vi "CRYAnalysis Editor.vi"() -> ()   [LabVIEW 2013]
uses:
  <vilib>/Utility/miscctls.llb/LVBoundsTypeDef.ctl
  Typedef Control/CRYAnalysis Cluster.ctl
  CRYProject/CRYProject Editor Global.vi
  CRYMainGlobal.vi
  Hardware/CRYHardware Global.vi
  CRYStepSetup/CRYStepSetup Global.vi
panel:
  out "Changed Curve 2":string[][](array[string])
  out "Analysis Bk":T1={"Name"="", "Harmonics"=[1.0], " Algorithm"=0, "delay"=0.0, "THD(%)"=FALSE, "Rub&Buzz"=FALSE, "Imp"=FALSE, "Imp Ref resistor"=1.0, "Y data"=0, "Y prefix"="", "Y unit"="", "Y dB ref"=1.0, "Custom Curve Names"=[], "har list items"=[""], "Envelope"=FALSE, "use custom unit"=FALSE, "autodelay ch"=0.0, "impulse"=FALSE, " start ms"=1.0, " stop ms"=1.0, "Scaling"=1, "Default Overlap "=FALSE, "Advanced View"=FALSE, "Loose Particle"=FALSE, "Use default"=FALSE, "Auto-Correlation(Stimulus)"=FALSE, "Auto-Correlation(Response)"=FALSE, "Deconvolved Response"=FALSE, "Mic Current"=FALSE, "M List Vaiues"=0, "Type"=0, "Delay Method"=3, "Apply Correction Out"=FALSE, "Apply Correction In"=FALSE, "Harmonics @ meas.frq"=FALSE, "THD Normalized(%)"=FALSE, "Total Distortion"=FALSE, "THD+Noise(%)"=FALSE, "Rub&Buzz Norm'd(%)"=FALSE, "Standard Error"=FALSE, "Confidence Limits"=FALSE, "Total Diff"=FALSE, "Total Noise"=FALSE, "Total DFD(%)"=FALSE, "Total IMD(%)"=FALSE, "Total IM"=FALSE, "Total DFD+Noise(%)"=FALSE, "Use Channel Name"=FALSE, "Waveform In"="", "Waveform Out"="", "Method"=3, "Spectral Scaling"=3, "Appliied Unit"=1, "Length Unit"=1, "Applied Units"=1, "Sens Item"=0, "Tab"=1, "Distance Unit"=0, "discard cycles"=1.0, "Weigting"="", "Averaging Time"=0.0, "Max duration"=0.0, "Min duration"=0.0, "Attack Threshold"=0.0, "Hysteresis Up"=0.0, "Fmin(Hz)"=0.0, "Fmax(Hz)"=0.0, "Freq.Resolution"=0.0, "Over-samples Res."=0.0, "Win Resolution"=0.0, "distance"=0.0, "samples"=1.0, "Overlap"=1.0, "Record Length"=1.0, "No.of FFTs"=0.0, "Hz"=1.0, "record delay"=1.0, " Std Err"=1.0, "Response"=FALSE, "Coherent Power*"=FALSE, "Stimulus"=FALSE, "Measurement Confidence"=FALSE, "Auto Spectrum(Response)*"=FALSE, "Auto Spectrum(Stimulus)*"=FALSE, "Cross Spectrum*"=FALSE, "functions"=FALSE, "Frequency Response"=FALSE, "Non-Coherent Power*"=FALSE, "Coherence (%)"=FALSE, "Non-Coherence (%)"=FALSE, "Signal-Noise Ratio (dB)"=FALSE, "Non-Coherenct Distirtion*"=FALSE, "Result Waveforms"=FALSE, "Coupling"=FALSE, "Averaging"=0, "Harmonics"=0, "Custom Curve Names"=0, "unLabel"="", "Custom Curve Names"="", "Unit"="", "Total IMD + Noise(%) "=FALSE, "ResponseMe"=1, "Intermod"=[1.0], "Diff\n"=[1.0], "Cross-Correlation"=FALSE, "IM list items"=[""], "Diff list items"=[""], "TSR Window Type"="", "Help"="", "Custom Curve IDs"=[], "Default Curve Names"=[], "Loose Particle waveform"=FALSE, "Perceptual Rub&Buzz"=FALSE, "Imp Auto Mode"=0, "Mic Auto Mode"=0, "Mic Ref resistor"=1.0, "Curve Resolution"=3, "Curve Resolution Hz"=0.0, "Polarity"=FALSE} {"Curve Resolution Hz" format="%.2f"; "Mic Ref resistor" format="%.2f"; "Diff" format="%.2f"; "Intermod" format="%.2f"; "ResponseMe" items=["Absolute", "Relative"]; "Std Err" format="%.1f"; "record delay" format="%.1f"; "Hz" format="%.1f"; "No.of FFTs" format="%.2f"; "Record Length" format="%.1f"; "Overlap" format="%.1f"; "samples" format="%.1f"; "distance" format="%.2f"; "Win Resolution" format="%.2f"; "Over-samples Res." format="%.2f"; "Freq.Resolution" format="%.2f"; "Fmax(Hz)" format="%.2f"; "Fmin(Hz)" format="%.2f"; "Hysteresis Up" format="%.2f"; "Attack Threshold" format="%.2f"; "Min duration" format="%.2f"; "Max duration" format="%.2f"; "Averaging Time" format="%.2f"; "Distance Unit" items=["Absolute", "Relative"]; "Sens Item" items=["x", "y", "z"]; "Applied Units" items=["Absolute", "Relative"]; "Length Unit" items=["Absolute", "Relative"]; "Appliied Unit" items=["Absolute", "Relative"]; "Spectral Scaling" items=["Absolute", "Relative"]; "M List Vaiues" items=["x", "y", "z"]; "Scaling" format="%.1f"; "stop ms" format="%.1f"; "start ms" format="%.1f"; "Y data" items=["dB", "Lin"]; "Y dB ref" format="%.1f"; "Imp Ref resistor" format="%.2f"; "Harmonics" format="%.2f"; "delay" format="%.2f"}
  in  "CurLibChange":bool caption="Add Lib"
  in  "Change Use Channel?":bool
  in  "Manual Apply":bool caption="Apply"
  in  "Mode":string
  out "Old Name":string[](array[string])
  out "Changed Curve":string[][](array[string])
  in  "Change Curve Name?":bool
  out "EndFlag":bool
  in  "Add Lib":bool
  in  "AddStep":bool
  in  "CurveUpdate":bool
  out "Wave In Fs":dbl
  out "Wave Ou Sn":dbl
  out "Wave Out Fs":dbl
  in  "Delay Treat":u16(slide)
  out "Common dB #":u16
  out "Wave In Sn":i32
  in  "distance":dbl
  in  "Visible Update":bool
  in  "Diff checkoffs":bool[](array[boolean])
  out "Diff array out":dbl[](array[numeric]) format="%.2f"
  in  "IM checkoffs":bool[](array[boolean])
  out "IM array out":dbl[](array[numeric]) format="%.2f"
  out "Harmonics array out":dbl[](array[numeric]) format="%.2f"
  out "CurveArrayByType":string[](array[string])
  in  "Hardware In Fs":dbl
  out "Analysis":T1={"Name"="", "Harmonics"=[1.0], " Algorithm"=0, "delay"=0.0, "THD(%)"=FALSE, "Rub&Buzz"=FALSE, "Imp"=FALSE, "Imp Ref resistor"=1.0, "Y data"=0, "Y prefix"="", "Y unit"="", "Y dB ref"=1.0, "Custom Curve Names"=[], "har list items"=[""], "Envelope"=FALSE, "use custom unit"=FALSE, "autodelay ch"=0.0, "impulse"=FALSE, " start ms"=1.0, " stop ms"=1.0, "Scaling"=1, "Default Overlap "=FALSE, "Advanced View"=FALSE, "Loose Particle"=FALSE, "Use default"=FALSE, "Auto-Correlation(Stimulus)"=FALSE, "Auto-Correlation(Response)"=FALSE, "Deconvolved Response"=FALSE, "Mic Current"=FALSE, "M List Vaiues"=0, "Type"=0, "Delay Method"=3, "Apply Correction Out"=FALSE, "Apply Correction In"=FALSE, "Harmonics @ meas.frq"=FALSE, "THD Normalized(%)"=FALSE, "Total Distortion"=FALSE, "THD+Noise(%)"=FALSE, "Rub&Buzz Norm'd(%)"=FALSE, "Standard Error"=FALSE, "Confidence Limits"=FALSE, "Total Diff"=FALSE, "Total Noise"=FALSE, "Total DFD(%)"=FALSE, "Total IMD(%)"=FALSE, "Total IM"=FALSE, "Total DFD+Noise(%)"=FALSE, "Use Channel Name"=FALSE, "Waveform In"="", "Waveform Out"="", "Method"=3, "Spectral Scaling"=3, "Appliied Unit"=1, "Length Unit"=1, "Applied Units"=1, "Sens Item"=0, "Tab"=1, "Distance Unit"=0, "discard cycles"=1.0, "Weigting"="", "Averaging Time"=0.0, "Max duration"=0.0, "Min duration"=0.0, "Attack Threshold"=0.0, "Hysteresis Up"=0.0, "Fmin(Hz)"=0.0, "Fmax(Hz)"=0.0, "Freq.Resolution"=0.0, "Over-samples Res."=0.0, "Win Resolution"=0.0, "distance"=0.0, "samples"=1.0, "Overlap"=1.0, "Record Length"=1.0, "No.of FFTs"=0.0, "Hz"=1.0, "record delay"=1.0, " Std Err"=1.0, "Response"=FALSE, "Coherent Power*"=FALSE, "Stimulus"=FALSE, "Measurement Confidence"=FALSE, "Auto Spectrum(Response)*"=FALSE, "Auto Spectrum(Stimulus)*"=FALSE, "Cross Spectrum*"=FALSE, "functions"=FALSE, "Frequency Response"=FALSE, "Non-Coherent Power*"=FALSE, "Coherence (%)"=FALSE, "Non-Coherence (%)"=FALSE, "Signal-Noise Ratio (dB)"=FALSE, "Non-Coherenct Distirtion*"=FALSE, "Result Waveforms"=FALSE, "Coupling"=FALSE, "Averaging"=0, "Harmonics"=0, "Custom Curve Names"=0, "unLabel"="", "Custom Curve Names"="", "Unit"="", "Total IMD + Noise(%) "=FALSE, "ResponseMe"=1, "Intermod"=[1.0], "Diff\n"=[1.0], "Cross-Correlation"=FALSE, "IM list items"=[""], "Diff list items"=[""], "TSR Window Type"="", "Help"="", "Custom Curve IDs"=[], "Default Curve Names"=[], "Loose Particle waveform"=FALSE, "Perceptual Rub&Buzz"=FALSE, "Imp Auto Mode"=0, "Mic Auto Mode"=0, "Mic Ref resistor"=1.0, "Curve Resolution"=3, "Curve Resolution Hz"=0.0, "Polarity"=FALSE} {"Curve Resolution Hz" format="%.2f"; "Mic Ref resistor" format="%.2f"; "Diff" format="%.2f"; "Intermod" format="%.2f"; "ResponseMe" items=["Absolute", "Relative"]; "Std Err" format="%.1f"; "record delay" format="%.1f"; "Hz" format="%.1f"; "No.of FFTs" format="%.2f"; "Record Length" format="%.1f"; "Overlap" format="%.1f"; "samples" format="%.1f"; "distance" format="%.2f"; "Win Resolution" format="%.2f"; "Over-samples Res." format="%.2f"; "Freq.Resolution" format="%.2f"; "Fmax(Hz)" format="%.2f"; "Fmin(Hz)" format="%.2f"; "Hysteresis Up" format="%.2f"; "Attack Threshold" format="%.2f"; "Min duration" format="%.2f"; "Max duration" format="%.2f"; "Averaging Time" format="%.2f"; "Distance Unit" items=["Absolute", "Relative"]; "Sens Item" items=["x", "y", "z"]; "Applied Units" items=["Absolute", "Relative"]; "Length Unit" items=["Absolute", "Relative"]; "Appliied Unit" items=["Absolute", "Relative"]; "Spectral Scaling" items=["Absolute", "Relative"]; "M List Vaiues" items=["x", "y", "z"]; "Scaling" format="%.1f"; "stop ms" format="%.1f"; "start ms" format="%.1f"; "Y data" items=["dB", "Lin"]; "Y dB ref" format="%.1f"; "Imp Ref resistor" format="%.2f"; "Harmonics" format="%.2f"; "delay" format="%.2f"}
  in  "Load Test":bool
  out "Proper VI No":i32
  in  "Autodelay Channel":dbl
  out "VIMiniumBound":T2
  in  "Board Tab":enum32{"Page 1", "Page 2"}(tab)
  in  "Cancel":bool caption="Apply"
  in  "OK":bool caption="Apply"
  in  "Main Tab":T3(tab)
  in  "Use default":bool=TRUE caption="使用默认"
  in  "Use Channel Name":bool caption="使用频道名称"
  in  "Custom Curve Names":string[][](table) caption="自定义的曲线名称"
  in  "units":bool
  in  "Unit":string="Pa" caption="单位"
  in  "Applied Units":u16(ring) caption="应用单位" items=["seconds", "samples", "inches", "meters"]
  in  "Hz":dbl format="%#.3p"
  in  "LR":u16(ring) items=["unity cal-in sens-in", "CRY33x Mic 1 sens-in", "CRY33x Mic 2 sens-in", "CRY33x Mic 3 sens-in", "CRY33x Mic 4 sens-in", "USB In L sens-in", "USB In R sens-in", "unity cal-out sens-out", "CRY602 Mouth 1 sens-out", "CRY602 Mouth 2 sens-out", "USB Out R sens-out"]
  in  "Distance Unit":u16(ring) items=["英寸", "米"]
  in  "samples":dbl=44100000.0 caption="样本" min=1.0 format="%#.0f"
  in  "s":dbl caption="秒" format="%#.4f"
  in  "distance":dbl caption="距离" min=0.0 format="%#.2f"
  in  "Delay Method":u16(slide) caption="延迟方法"
  in  "Maxis":u16(slide) scale=0.0..2.0
  out "CurveLibValues":bool caption="曲线值"
  out "Record Delay":bool caption="记录延迟"
  in  "Polarity":bool caption="极性"
  out "Curve Resolution":bool caption="曲线分辨"
  out "Spectra":bool caption="频谱"
  in  "Auto-Spectrum(Response)*":bool caption="自动频谱(响应)"
  in  "Auto-Spectrum(Stimulus)*":bool caption="自动频谱(激励)"
  in  "Spectral Scaling*":u16(ring) caption="频谱缩放*" items=["有效值", "频谱密度"]
  in  "Non-Coherent Power*":bool caption="非相干功率*"
  in  "Coherent Power*":bool caption="相干功率*"
  in  "Cross-Spectrum*":bool caption="交叉频谱*"
  out "Functions":bool caption="功能"
  in  "Frequency Response":bool caption="频率响应"
  in  "Coherence (%)":bool=TRUE caption="相干(%)"
  in  "Non-Coherence (%)":bool=TRUE caption="非相干(%)"
  in  "Signal-Noise Ratio (dB)":bool=TRUE caption="信噪比(dB)"
  in  "Non-Coherent Distortion*":bool=TRUE caption="非相干失真"
  in  "Averaging1":u16(slide)
  out "Averaging":bool caption="平均"
  in  "Curve Step Resolution":u16(ring) caption="Resolution" items=["R10(1/3 Oct.)"=0, "R20(1/6 Oct.)"=1, "R40(1/12 Oct.)"=2, "R80(1/24 Oct.)"=3, "User Defined, Log"=5, "User Defined,Linear"=6]
  in  "Curve Resolution Hz":dbl=10.0 caption="Hz" min=0.0 max=100000000.0 format="%#_10p"
  in  "Hysteresis Up(dB)":dbl=20.0 caption="磁滞现象上升(dB)" format="%#_6p"
  in  "Min duration(s)":dbl=20.0 caption="最小持续时间(s)" min=0.001 format="%#_6p"
  in  "Attack Threshold(dB)":dbl=20.0 caption="激发界限(dB)" min=0.0 format="%#_6p"
  in  "Max duration(s)":dbl=20.0 caption="最大持续时间(s)" min=0.0 format="%#_6p"
  in  "Loose Particle":bool caption="松散离子"
  in  "Averaging Time(s)":dbl=20.0 caption="平均时间(s)" min=0.0 format="%#_6p"
  in  "Loose Particle Waveform":bool=TRUE caption="松散离子波形"
  out "Channel in":string="L" caption="输入通道"
  out "Type in":string="Frequency Stepped Sweep" caption="输入类型"
  in  "Waveforms In":u16(ring) caption="输入波形"
  in  "Apply Correction in":bool caption="应用输入修正"
  out "Channel Out":string="L" caption="输出通道"
  out "Type Out":string="Frequency Stepped Sweep" caption="输出类型"
  in  "Waveforms Out":u16(ring) caption="输出波形"
  in  "Apply Correction Out":bool caption="应用输出修正"
  out "Stimulus":bool caption="激励"
  out "Response":bool caption="响应"
  out "Response Measurement":bool caption="响应测量"
  in  "Response Measurement1":u16(slide)
  in  "Perceptual Rub & Buzz(phons)":bool caption="感知异音(phons)"
  in  "Total DFD + Noise(%)":bool caption="共有DFD+噪声(%)"
  in  "Total DFD (%)":bool caption="共有DFD(%)"
  in  "Total Diff":bool caption="总差异"
  in  "THD + Noise (%)":bool caption="总谐波失真+噪声(%)"
  in  "THD Normalized(%)":bool caption="总谐波失真(归一化)(%)"
  in  "Rub & Buzz Norm'd(%)":bool caption="异音(归一化)(%)"
  in  "Rub & Buzz(%)":bool
  in  "Total Distortion":bool caption="总失真"
  in  "Harmonics @ meas.frq":bool caption="谐波测量频率"
  in  "Total IMD + Noise(%)":bool caption="共有IMD+噪声(%)"
  in  "Total IMD(%)":bool caption="共有IMD(%)"
  in  "Total IM":bool caption="共有IM"
  in  "Total Noise":bool caption="总噪声"
  in  "+/-":dbl=1.0 caption="标准错误" min=1.0 max=6.0 format="%#_6p"
  in  "Confidence Limits":bool caption="置信界限"
  in  "Standard Error":bool caption="标准差"
  in  "THD(%)":bool caption="总谐波失真(%)"
  out "Measurement Confidence":bool caption="测量置信度"
  in  "Edit List":bool
  in  "Method":u16(slide)
  in  "Type":u16(slide) caption="类型"
  in  "Harmonics":i32(listbox) caption="谐波"
  in  "Orders IM":i32(listbox) caption="次数"
  in  "Orders Diff":i32(listbox) caption="次数"
  in  "TSR Window Type":u16(ring) caption="TSR窗函数类型" items=["None", "Cosine Tapered", "Half-Cosine Tapered", "Exponential", "Adrienne", "Half-Hanning", "Half-BH4"]
  in  "Cross-Correlation":bool caption="互相关"
  out "No.of FFTs":i32=1 caption="FFT数量"
  out "Record Length (s)":dbl caption="FFT长度(s)" format="%#_3p"
  in  "Freq.Resolution(Hz)":dbl=10.0 caption="频率响应(Hz)" min=0.0 max=100000000.0 format="%#_10p"
  out "Windowed Resolution(Hz)":dbl=40.0 caption="窗函数分辨率(Hz)" format="%#.3p"
  in  "Over-samples Res.(Hz)":dbl=5.0 caption="曲线分辨率(Hz)" min=0.0 format="%#_6p"
  in  "StopTime(s)":dbl=10.0 caption="停止时间(秒)" min=0.0 format="%#_6p"
  in  "Start Time(s)":dbl=14.0 caption="开始时间(秒)" min=0.0 format="%#_6p"
  in  "Auto-Correlation(Response)":bool caption="自动相关(响应)"
  in  "Auto-Correlation(Stimulus)":bool caption="自动相关(激励)"
  in  "Deconvolved Response":bool caption="逆卷积响应"
  in  "Discard Cycles":dbl caption="丢弃周期" min=0.0 max=1000.0 format="%#_6p"
  in  "Fmin(Hz)":dbl=20.0 caption="最低频率(Hz)" min=0.0 format="%#_6p"
  in  "Fmax(Hz)":dbl=20000.0 caption="最大频率(Hz)" min=0.0 format="%#_6p"
  in  "Default Overlap":bool caption="默认重叠"
  in  "Overlap(%)":dbl=85.0 caption="重叠(%)" min=0.0 max=100.0 format="%#_6p"
  in  "Weighting":u16(ring) caption="加权" items=["None"=0, "Hanning"=1, "4 Term B-Harris"=7, "7 Term B-Harris"=8, "Flat Top"=6]
  in  "Envelope?":bool caption="时间包络"
  in  "impulse resp?":bool caption="冲击响应"
  in  "Scaling":i32(ring) caption="刻度" items=["dB", "Linear"]
  out "Result Waveforms":bool caption="结果波形"
  in  "Mic Auto Mode":u16(slide) caption="File Name Mode1"
  in  "Mic Resistor(ohm)":dbl caption="麦克风电阻(ohm)" min=0.0 format="%#_6p"
  in  "Amp Auto Mode":u16(slide) caption="File Name Mode1"
  out "Impedance Frame":bool caption="阻抗"
  in  "Reference Resistor(ohm)":dbl caption="参考电阻(ohm)" min=0.0 format="%#_6p"
  in  "Mic Current":bool caption="麦克风电流"
  in  "Impedance":bool caption="阻抗"
  out "Mic Frame":bool caption="麦克风"
  in  "Help":string
  in  "Advanced View":bool caption="高级选项"
  in  "Apply":bool
  in  "Algorithm":u16(ring) caption="算法" items=["宽频带有效值分析", "FFT频谱", "谐波跟踪分析", "差频分析", "时间选择响应分析", "多音分析", "传递函数分析"]
  in  "Save As...":bool caption="Apply"
  in  "Revert":bool caption="Apply"
  in  "Load...":bool caption="Apply"
  in  "har checkoffs":bool[](array[boolean])
  in  "stop":bool
  in  "Y data":u16(ring)=1 items=["dB", "Lin"]
  in  "Y dB ref":dbl=1.0 format="%.1f"
  in  "Y unit":string
  in  "Y prefix":string
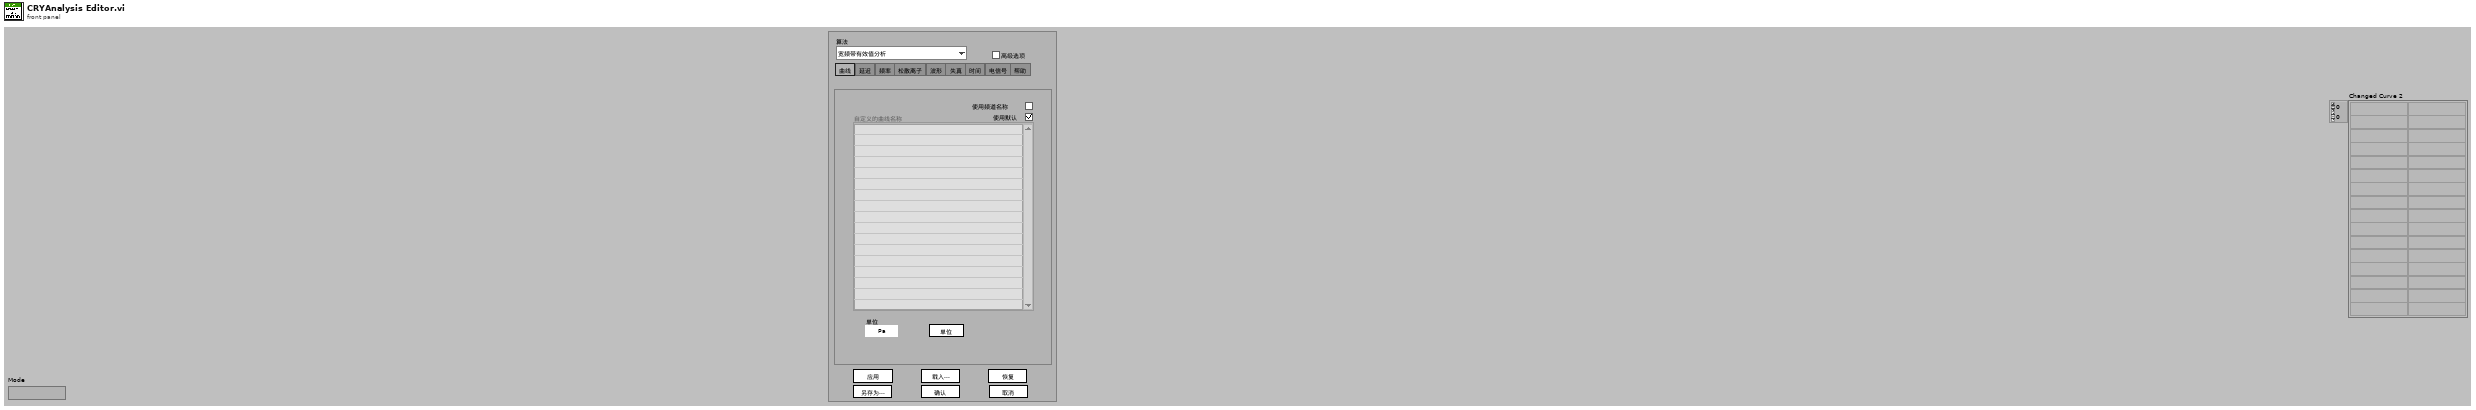
[diagram p1: front panel]
types:
  T1 = typedef "CRYAnalysis Cluster.ctl" = cluster{"Name":string, "Harmonics":dbl[], " Algorithm":u16, "delay":dbl, "THD(%)":bool, "Rub&Buzz":bool, "Imp":bool, "Imp Ref resistor":dbl, "Y data":u16, "Y prefix":string, "Y unit":string, "Y dB ref":dbl, "Custom Curve Names":string[], "har list items":string[], "Envelope":bool, "use custom unit":bool, "autodelay ch":dbl, "impulse":bool, " start ms":dbl, " stop ms":dbl, "Scaling":i32, "Default Overlap ":bool, "Advanced View":bool, "Loose Particle":bool, "Use default":bool, "Auto-Correlation(Stimulus)":bool, "Auto-Correlation(Response)":bool, "Deconvolved Response":bool, "Mic Current":bool, "M List Vaiues":u16, "Type":u16, "Delay Method":u16, "Apply Correction Out":bool, "Apply Correction In":bool, "Harmonics @ meas.frq":bool, "THD Normalized(%)":bool, "Total Distortion":bool, "THD+Noise(%)":bool, "Rub&Buzz Norm'd(%)":bool, "Standard Error":bool, "Confidence Limits":bool, "Total Diff":bool, "Total Noise":bool, "Total DFD(%)":bool, "Total IMD(%)":bool, "Total IM":bool, "Total DFD+Noise(%)":bool, "Use Channel Name":bool, "Waveform In":string, "Waveform Out":string, "Method":u16, "Spectral Scaling":u16, "Appliied Unit":u16, "Length Unit":u16, "Applied Units":u16, "Sens Item":u16, "Tab":i32, "Distance Unit":u16, "discard cycles":dbl, "Weigting":string, "Averaging Time":dbl, "Max duration":dbl, "Min duration":dbl, "Attack Threshold":dbl, "Hysteresis Up":dbl, "Fmin(Hz)":dbl, "Fmax(Hz)":dbl, "Freq.Resolution":dbl, "Over-samples Res.":dbl, "Win Resolution":dbl, "distance":dbl, "samples":dbl, "Overlap":dbl, "Record Length":dbl, "No.of FFTs":dbl, "Hz":dbl, "record delay":dbl, " Std Err":dbl, "Response":bool, "Coherent Power*":bool, "Stimulus":bool, "Measurement Confidence":bool, "Auto Spectrum(Response)*":bool, "Auto Spectrum(Stimulus)*":bool, "Cross Spectrum*":bool, "functions":bool, "Frequency Response":bool, "Non-Coherent Power*":bool, "Coherence (%)":bool, "Non-Coherence (%)":bool, "Signal-Noise Ratio (dB)":bool, "Non-Coherenct Distirtion*":bool, "Result Waveforms":bool, "Coupling":bool, "Averaging":u16, "Harmonics":i32, "Custom Curve Names":i32, "unLabel":string, "Custom Curve Names":string, "Unit":string, "Total IMD + Noise(%) ":bool, "ResponseMe":u16, "Intermod":dbl[], "Diff\n":dbl[], "Cross-Correlation":bool, "IM list items":string[], "Diff list items":string[], "TSR Window Type":string, "Help":string, "Custom Curve IDs":i32[], "Default Curve Names":string[], "Loose Particle waveform":bool, "Perceptual Rub&Buzz":bool, "Imp Auto Mode":u16, "Mic Auto Mode":u16, "Mic Ref resistor":dbl, "Curve Resolution":u16, "Curve Resolution Hz":dbl, "Polarity":bool}
  T2 = typedef "LVBoundsTypeDef.ctl" = cluster{"Width":u32, "Height":u32}
  T3 = enum32{"Curves", "Delay", "Frequency", "Loose Part    ", "Waveforms", "Distortion", "Time", "Eelectrical", "Help"}
  T4 = typedef "CRYStep.ctl" = cluster{"No.VI":i32, "Category":string, "StepName":string, "Seq setup flattened":string, "Comment":string, "Steps config.":bool[], "Jump config":i32[], "Start":dbl, "Increment":dbl, "Name":string, "Unit":string, "Y data":u16, "Y prefix":string, "Y dB ref":dbl, "Y unit":string, "Repeat State Array":cluster{"Start":dbl, "Increment":dbl, "Count":i32, "Num":i32}[]}
  T5 = typedef "CRYData Cluster Array.ctl" = T6[]
  T6 = typedef "CRYData Cluster.ctl" = cluster{"Name":string, "Curve":cluster{"x":dbl, "y":dbl, "z":dbl}[], "X data":u16, "Y data":u16, "Z data":u16, "X axis":u16, "Y axis":u16, "Z axis":u16, "X unit":string, "Y unit":string, "Z unit":string, "X dB ref":dbl, "Y dB ref":dbl, "Z dB ref":dbl, "single val":bool, "protected":bool, "display X":bool, "display Y":bool, "display Z":bool, "Test Info":string, "Step No.":i32, "Plot Settings":cluster{"Color":u32, "Interpolation":u8, "Point Style":u8, "Line Style":u8, "Point Color":u32, "Line Width":u8, "Bar Plot Style":u8, "Fill To":i16}, "AutoProtect":bool}
  T7 = enum16{"OK", "Yes", "YesNo", "YesNoCancel", "ReplaceAppend"}
  T8 = enum32{"Page Enabled", "Page Disabled", "Page Disabled & Grayed"}
  T9 = enum32{"Curves", "Delay", "Frequency", "Loose Part    ", "Waveforms", "Distortion", "Time", "Eelectrical"}
  T10 = enum16{"Broadband RMS", "Spectrum", "Hamonic Track", "Heterodyne", "Time Selective Response", "Multitone", "Transfer Function"}
  T11 = enum8{"Enabled", "Disabled", "Disabled and Grayed Out"}
  T12 = typedef "CRYWaveform Cluster Array.ctl" = T13[]
  T13 = typedef "CRYWaveform Cluster.ctl" = cluster{"Waveform":cluster{"X0":dbl, "dX":dbl, "Y":sgl[]}, "X data":u16, "Y data":u16, "Y axis":u16, "X unit":string, "Y unit":string, "Y dB ref":dbl, "display Y":bool, "display X":bool, "Overload?":bool, "Test Info":string, "Step No.":i32, "Name":string, "protected":bool, "Sqc history":string[], "Signal Channel ID":i32, "Plot Settings":cluster{"Color":u32, "Interpolation":u8, "Point Style":u8, "Line Style":u8, "Point Color":u32, "Line Width":u8, "Bar Plot Style":u8, "Fill To":i16}, "AutoProtect":bool}
  T14 = cluster{"Custom Curve Names":string, "Custom Curve IDs":i32, "Default Curve Names":string}[]
  T15 = typedef "CRYStimulus Test Infor Cluster.ctl" = cluster{"Stimulus Type":string, "Signal Type":string, "In/Out":bool, "FAPS":cluster{"freq":dbl, "ampl":dbl, "cycles":dbl, "samples":i32}[], "Sampling Rate":dbl, "Samples":i32, "Analysis Param":string, "Resolution":u16, "Steps":u32, "Analysis Value":dbl[], "Diff Freq":dbl, "FStart":dbl, "FStop":dbl, "Calibration Param":string, "Anti Alias":dbl, "Level Out1":dbl, "Level Out2":dbl, "EQ":bool}
  T16 = typedef "CRYCalibration All Cluster.ctl" = cluster{"Calibration 2D":T17[], "Help":string, "Tab Value":i32, "Input Signal Type":string, "Output Signal Type":string}
  T17 = typedef "CRYCalibration 2DCluster.ctl" = cluster{"Calibration":T18, "Corr Curve":T6, "EQ Curve":T6, "Sens Curve":T6}
  T18 = typedef "CRYCalibration Cluster.ctl" = cluster{"Calibration Step Name":string, "Device":string, "Correction Curve Name":string, "Equalization Curve Name":string, "Sensitivity Curve Name":string, "Corr Folder and File":string, "EQ Folder and File":string, "Sens Folder and File":string, "Corr Step size":u16, "EQ Step size":u16, "Input":bool, "Last Cal Date (sec)":timestamp, "Cha Name":string, "Corr Curve Found":bool, "EQ Curve Found":bool, "Sens Curve Found":bool, "Signal Type":string, "Calibrated Device":string, "Hz":u32}
  T19 = typedef "CRYHardware Channel Info.ctl" = cluster{"ID":i32, "Name":string, "Digital":bool, "Input":bool, "Device Name":string, "Hardware Ch ID":u8, "Vmax (V)":dbl, "Latency (samples)":dbl, "Sampling Rate (Hz)":u32, "Bit Depth":u32, "Anti-aliasing Factor (%fs)":sgl, "DAQmx Channel":tag, "term config":i32, "Coupling":i32, "IEPE en":bool, "ASIOChannel Name":string, "Audio Driver":u16, "ASIOChannel Index":u8}
  T20 = cluster{bool, "Check Option":string, "use custom unit":bool, "Custom Curve Names":string[], "Custom Curve IDs":i32[], "Default Curve Names":string[], "Use default":bool}
  T21 = typedef "CRYAnalysis CurveName Cluster.ctl" = cluster{"Custom Curve Name":string, "Custom Curve ID":i32, "Default Curve Name":string}[]
  T22 = cluster{"Custom Curve Name":string, "Custom Curve ID":i32, "Default Curve Name":string}
  T23 = cluster{bool, "units":bool, "Edit List":bool, "Load Test":bool, "Add Lib":bool, "OK":bool, "Cancel":bool}
  T24 = cluster{"Scale visible?":bool, "use custom unit":bool}
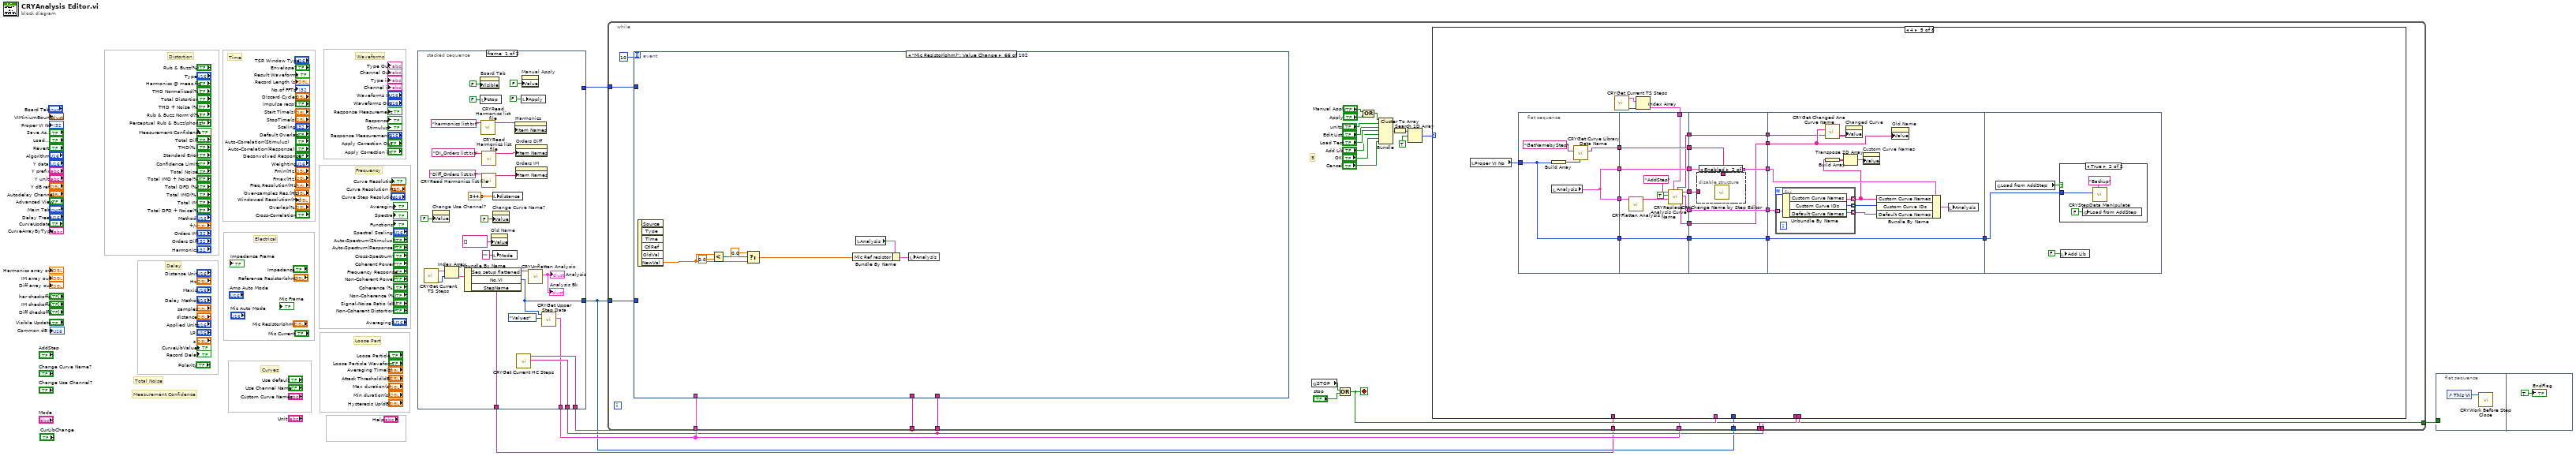
[diagram p0: block diagram]
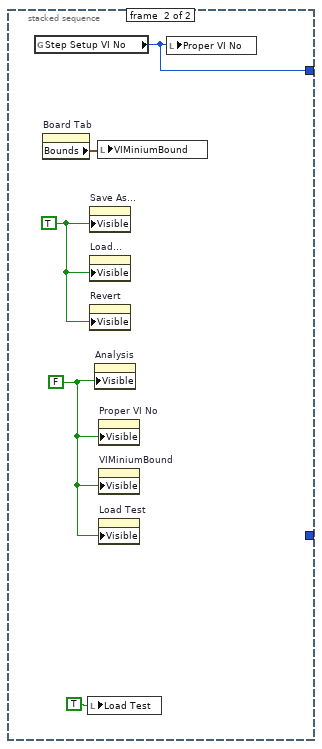
[diagram p2: hidden frame]
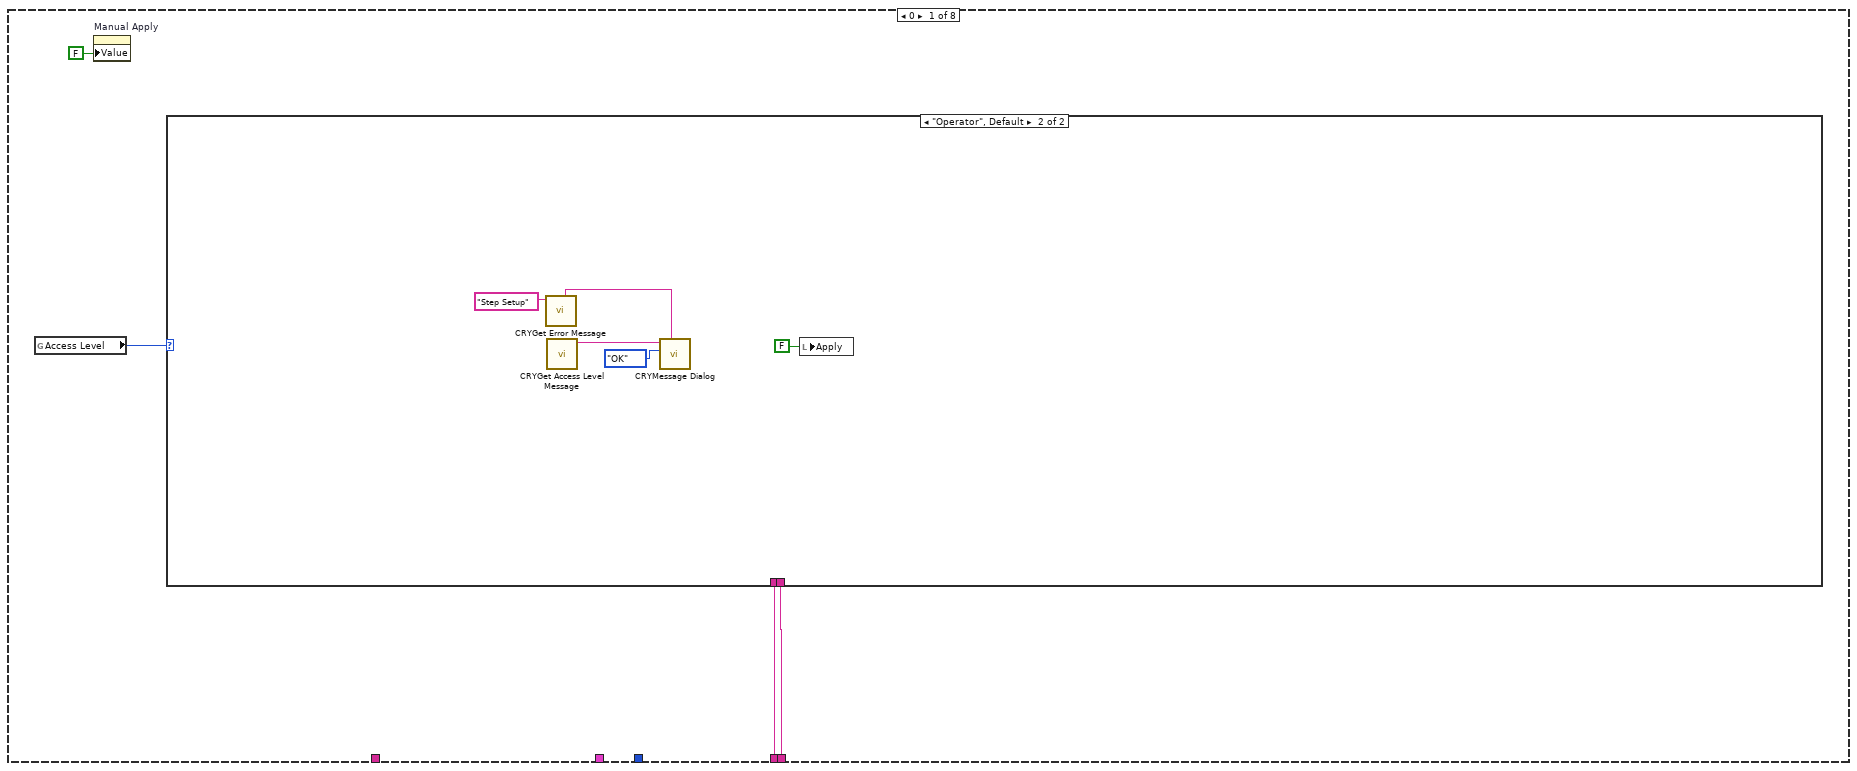
[diagram p3: hidden frame]
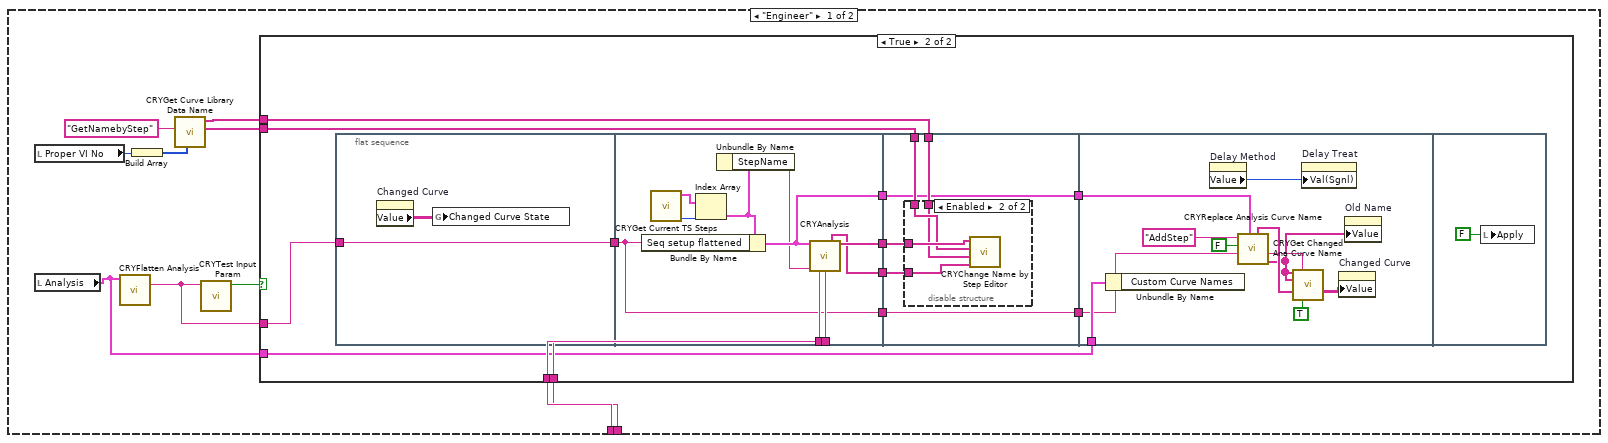
[diagram p4: hidden frame]
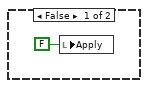
[diagram p5: hidden frame]
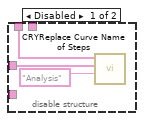
[diagram p6: hidden frame]
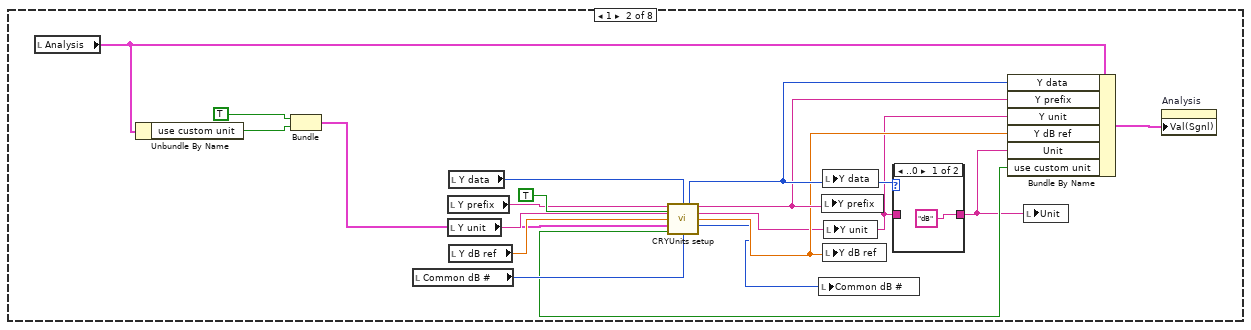
[diagram p7: hidden frame]
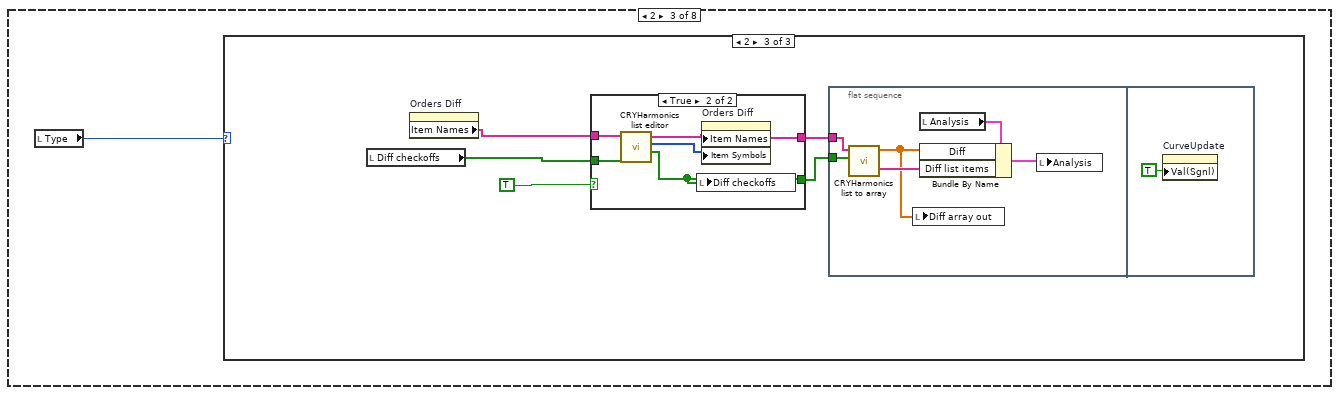
[diagram p9: hidden frame]
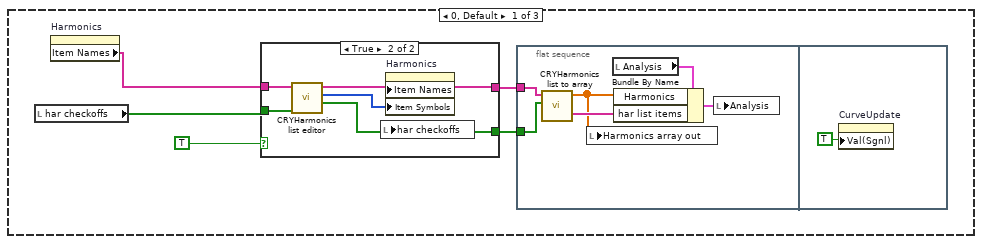
[diagram p10: hidden frame]
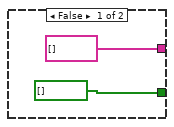
[diagram p11: hidden frame]
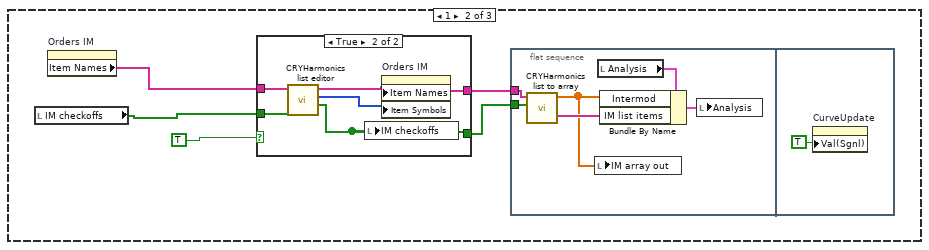
[diagram p12: hidden frame]
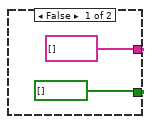
[diagram p13: hidden frame]
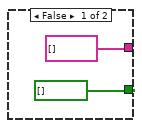
[diagram p14: hidden frame]
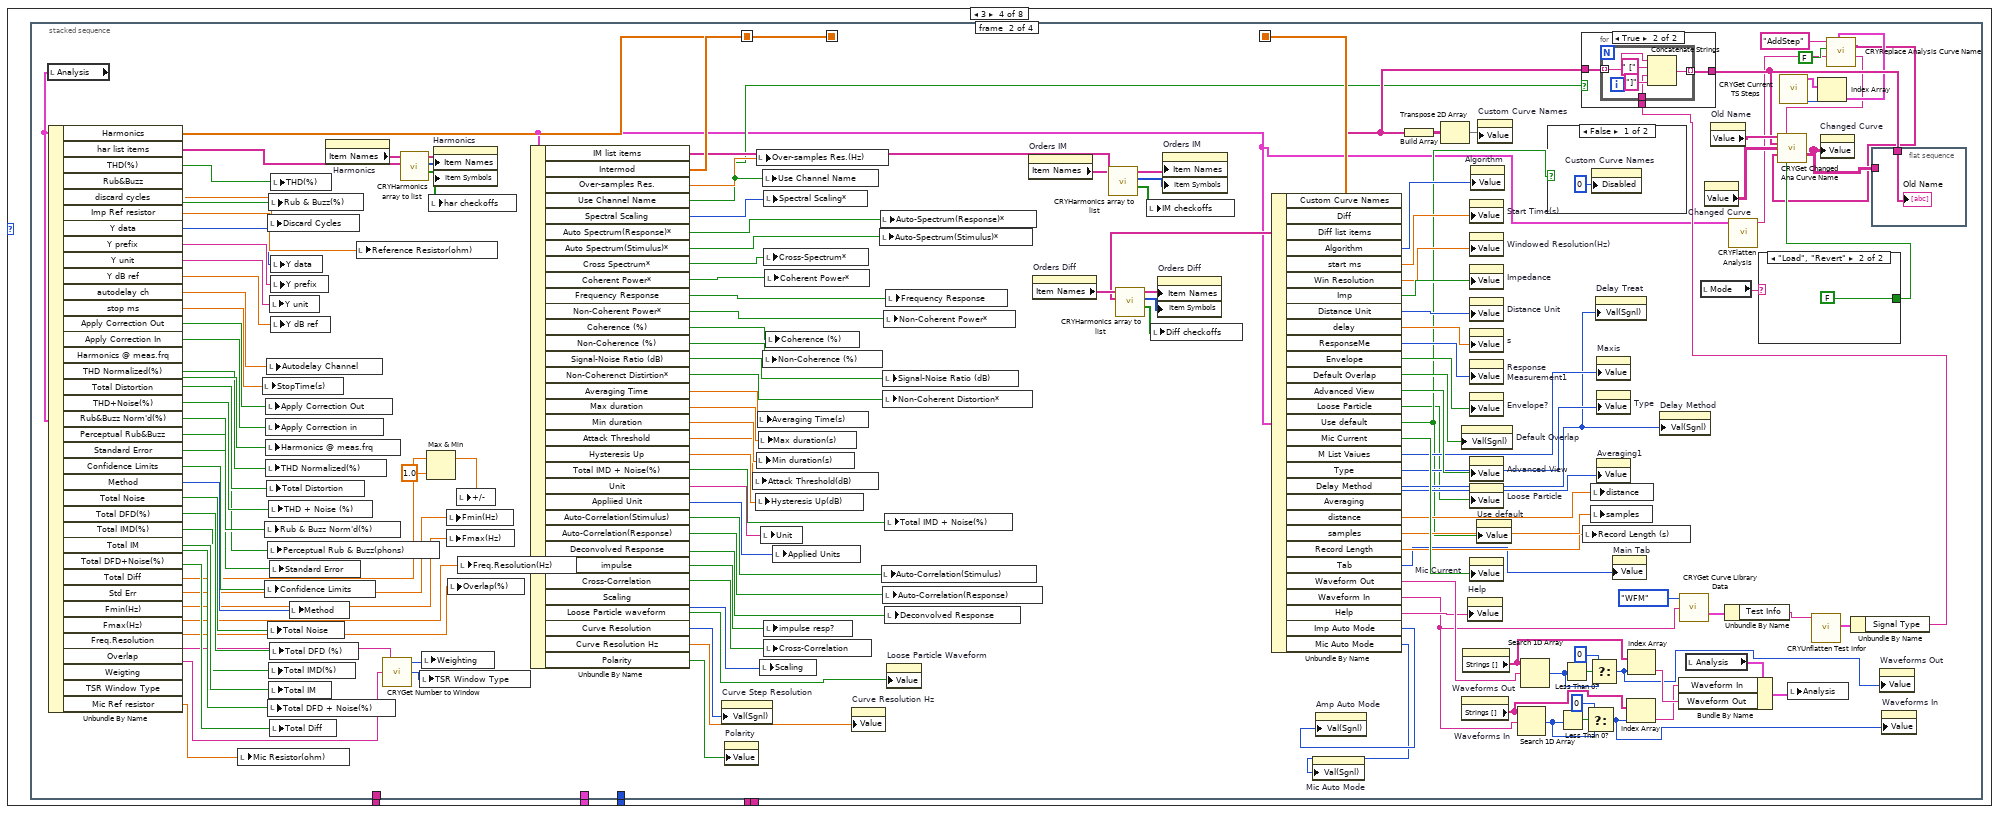
[diagram p15: hidden frame]
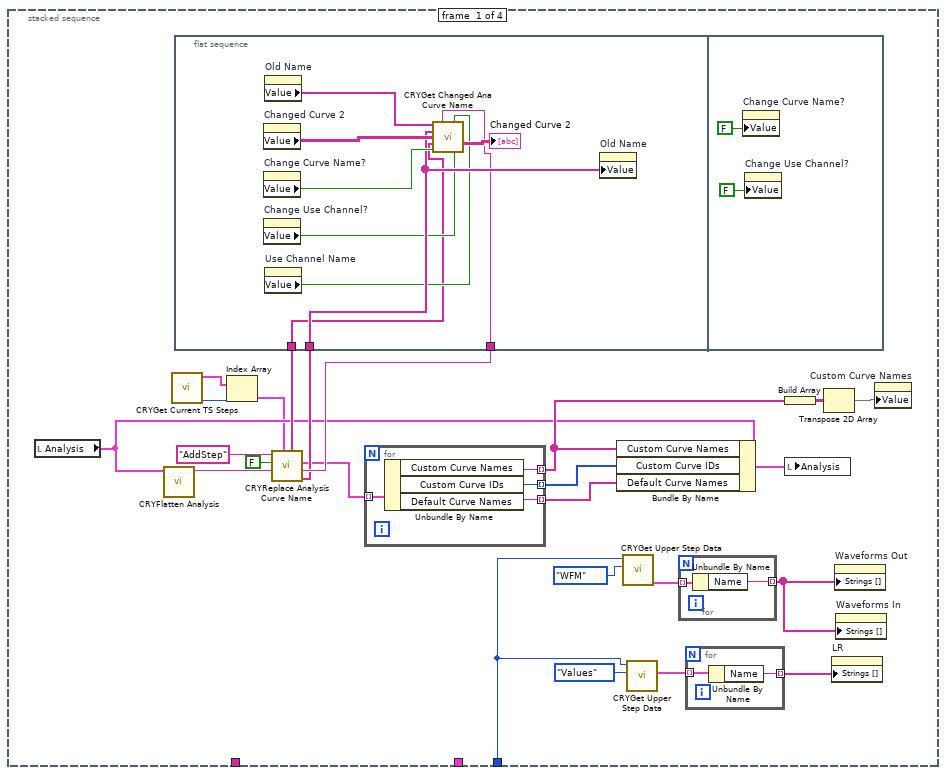
[diagram p16: hidden frame]
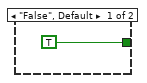
[diagram p18: hidden frame]
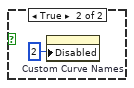
[diagram p19: hidden frame]
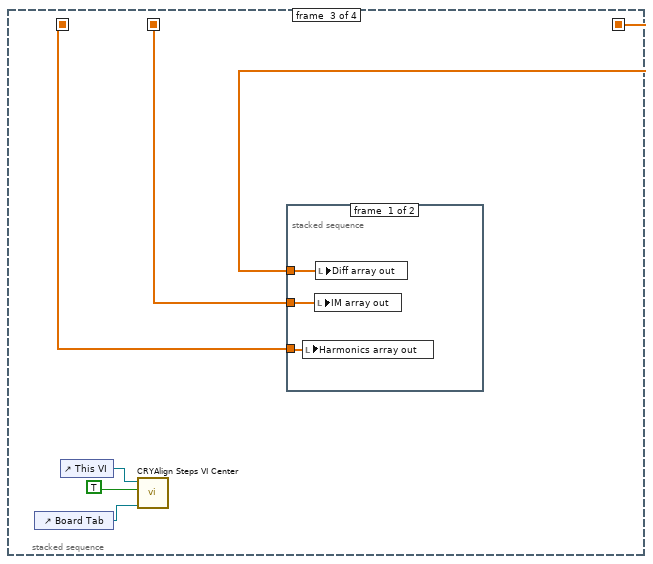
[diagram p20: hidden frame]
diagram:
  # "Measurement Confidence"
  # "Total Noise"
  # "Loose Part"
  # "Frequency"
  # "Delay"
  # "Curves"
  # "Electrical"
  # "Distortion"
  # "Waveforms"
  # "Time"
  n1 = stacked-sequence {
    tunnel: [w30 _] -> w7
    tunnel: [w29 _] -> w4
    tunnel: [w27 _] -> w6
    tunnel: [_ w37] -> w5
    tunnel: [w11 _] -> w1
    tunnel: [w8 _] -> w2
    frame #0 {
      n2 = call "CRYGet Current TS Steps.vi"() -> ("SelectStepNumber in Tree"=w17:i32, "Steps"=w18:T4[])  [unwired: 1 in, 9 out]
      n3 = property on="Change Use Channel?" class="Bool (strict)"("Value"=FALSE ("Change Use Channel?")) -> ()  [unwired: 2 in, 2 out]
      n4 = Index Array(array=w18, index=w17) -> (element=w19:T4)
      n5 = Unbundle By Name(w19) -> ("Seq setup flattened"=w20:string, "No.VI"=w11:i32, "StepName"=w8:string)
      n6 = property on="Board Tab" class="TabCtl (strict)"("Visible"=FALSE) -> ()  [unwired: 2 in, 2 out]
      n7 = local write "stop"(FALSE ("continue loop?")) -> ()
      n8 = call "CRYRead Harmonics list file.vi"("String"="harmonics list.txt") -> ("Harmonics list"=w26:string[])  [unwired: 10 out]
      n9 = call "CRYRead Harmonics list file.vi"("String"="DI_Orders list.txt") -> ("Harmonics list"=w24:string[])  [unwired: 10 out]
      n10 = call "CRYRead Harmonics list file.vi"("String"="Diff_Orders list.txt") -> ("Harmonics list"=w22:string[])  [unwired: 10 out]
      n11 = property on="Old Name" class="Arr (strict)"("Value"=string[] [] ("Old Name")) -> ()  [unwired: 2 in, 2 out]
      n12 = local write "distance"(344.0 ("distance")) -> ()
      n13 = property on="Change Curve Name?" class="Bool (strict)"("Value"=FALSE ("Change Curve Name?")) -> ()  [unwired: 2 in, 2 out]
      n14 = local write "Mode"("" ("Mode")) -> ()
      n15 = property on="Harmonics" class="LstBox (strict)"("Item Names"=w26) -> ()  [unwired: 2 in, 2 out]
      n16 = property on="Orders Diff" class="LstBox (strict)"("Item Names"=w24) -> ()  [unwired: 2 in, 2 out]
      n17 = property on="Orders IM" class="LstBox (strict)"("Item Names"=w22) -> ()  [unwired: 2 in, 2 out]
      n18 = call "CRYGet Current HC Steps.vi"() -> ("Calibration setup flattened Out"=w29:string, "Hardware setup flattened Out"=w30:string)  [unwired: 10 out]
      n19 = local write "Apply"(FALSE ("Apply")) -> ()
      n20 = property on="Manual Apply" class="Bool (strict)"("Value"=FALSE ("Manual Apply")) -> ()  [unwired: 2 in, 2 out]
      n21 = call "CRYUnflatten Analysis.vi"("Unflatten Analysis"=w20) -> ("Analysis"=→"Analysis" →"Analysis Bk":T1)  [unwired: 10 out]
      n22 = call "CRYGet Upper Step Data.vi"("Type In"=enum16{"Curves", "Values", "Results", "WFM"}."Values", "No.VI"=w11) -> ("Value array"=w27:T5)  [unwired: 9 out]
    }
    frame #1 {
      w35 = TRUE ("Visible")
      w34 = FALSE ("Visible")
      n23 = global read "CRYProject Editor Global.vi" "Step Setup VI No"() -> (w37:i32)
      n24 = property on="Board Tab" class="TabCtl (strict)"() -> ("Bounds"=w36:T2)  [unwired: 2 in, 2 out]
      n25 = local write "Load Test"(TRUE ("Visible")) -> ()
      n26 = property on="Save As..." class="Bool (strict)"("Visible"=w35) -> ()  [unwired: 2 in, 2 out]
      n27 = property on="Load..." class="Bool (strict)"("Visible"=w35) -> ()  [unwired: 2 in, 2 out]
      n28 = property on="Revert" class="Bool (strict)"("Visible"=w35) -> ()  [unwired: 2 in, 2 out]
      n29 = property on="Analysis" class="Clust (strict)"("Visible"=w34) -> ()  [unwired: 2 in, 2 out]
      n30 = local write "VIMiniumBound"(w36) -> ()
      n31 = property on="Proper VI No" class="DigNum (strict)"("Visible"=w34) -> ()  [unwired: 2 in, 2 out]
      n32 = property on="VIMiniumBound" class="Clust (strict)"("Visible"=w34) -> ()  [unwired: 2 in, 2 out]
      n33 = property on="Load Test" class="Bool (strict)"("Visible"=w34) -> ()  [unwired: 2 in, 2 out]
      n34 = local write "Proper VI No"(w37) -> ()
    }
  }
  n35 = while {
    tunnel: w7 -> [w57]
    tunnel: w4 -> [w51]
    tunnel: w7 -> [w56]
    tunnel: w6 -> [w55]
    tunnel: w6 -> [w54]
    tunnel: w5 -> [w50]
    tunnel: w4 -> [w48]
    tunnel: w1 -> [w45]
    tunnel: [w44] -> w3
    tunnel: w2 -> [w40]
    tunnel: w1 -> [w39]
    stop <- w44 stop-if-true
    # "5"
    n36 = event shown="[65] \"Mic Resistor(ohm)\": Value Change" {
      selector: _ -> [_ _ _ _ _ _ _ _ _ _ _ _ _ _ _ _ _ _ _ _ _ _ _ _ _ _ _ _ _ _ _ _ _ _ _ _ _ _ _ _ _ _ _ _ _ _ _ _ _ _ _ _ _ _ _ _ _ _ _ _ _ _ _ _ _ _ _ _ _ _ _ _ _ _ _ _ _ _ _ _ _ _ _ _ _ _ _ _ _ _ _ _ _ _ _ _ _ _ _ _ _ _]
      dyn-events: _ -> [_ _ _ _ _ _ _ _ _ _ _ _ _ _ _ _ _ _ _ _ _ _ _ _ _ _ _ _ _ _ _ _ _ _ _ _ _ _ _ _ _ _ _ _ _ _ _ _ _ _ _ _ _ _ _ _ _ _ _ _ _ _ _ _ _ _ _ _ _ _ _ _ _ _ _ _ _ _ _ _ _ _ _ _ _ _ _ _ _ _ _ _ _ _ _ _ _ _ _ _ _ _]
      timeout: 10 -> [_ _ _ _ _ _ _ _ _ _ _ _ _ _ _ _ _ _ _ _ _ _ _ _ _ _ _ _ _ _ _ _ _ _ _ _ _ _ _ _ _ _ _ _ _ _ _ _ _ _ _ _ _ _ _ _ _ _ _ _ _ _ _ _ _ _ _ _ _ _ _ _ _ _ _ _ _ _ _ _ _ _ _ _ _ _ _ _ _ _ _ _ _ _ _ _ _ _ _ _ _ _]
      tunnel: w56 -> [_ _ _ _ _ _ _ _ _ _ _ _ _ _ w1149 _ _ _ _ _ _ _ _ _ _ _ _ _ _ _ _ _ _ _ _ _ _ _ _ _ _ _ _ _ _ _ _ _ _ _ _ _ _ _ _ _ _ _ _ _ _ _ _ _ _ _ _ _ _ _ _ _ _ _ _ _ _ _ _ _ _ _ _ _ _ _ _ _ _ _ _ _ _ _ _ _ _ _ _ _ _ _]
      tunnel: w54 -> [_ _ _ _ _ _ _ _ _ _ _ _ _ _ _ _ _ _ _ _ _ _ _ _ _ _ _ _ _ _ _ w1297 _ _ _ _ _ _ _ _ _ _ _ _ _ _ _ _ _ _ _ _ _ _ _ _ _ _ _ _ _ _ _ _ _ _ _ _ _ _ _ _ _ _ _ _ _ _ _ _ _ _ _ _ _ _ _ _ _ _ _ _ _ _ _ _ _ _ _ _ _ _]
      tunnel: w50 -> [_ _ _ _ _ _ _ _ _ _ _ _ _ _ _ _ _ _ _ _ _ _ _ _ _ _ _ _ _ _ _ _ _ _ _ _ _ _ _ _ _ _ _ _ _ _ _ _ _ _ _ _ _ _ _ _ _ _ _ _ _ _ _ _ _ _ _ _ _ _ _ _ _ _ _ _ _ _ _ _ _ _ _ _ _ _ _ _ _ _ _ _ _ _ _ _ _ _ _ _ _ _]
      tunnel: w48 -> [_ _ _ _ _ _ _ _ _ _ _ _ _ _ w1140 _ _ _ _ _ _ _ _ _ _ _ _ _ _ _ _ _ _ _ _ _ _ _ _ _ _ _ _ _ _ _ _ _ _ _ _ _ _ _ _ _ _ _ _ _ _ _ _ _ _ _ _ _ _ _ _ _ _ _ _ _ _ _ _ _ _ _ _ _ _ _ _ _ _ _ _ _ _ _ _ _ _ _ _ _ _ _]
      tunnel: w45 -> [_ _ _ _ _ _ w596 _ _ _ _ _ _ _ _ _ _ _ _ _ _ _ _ _ _ _ _ _ _ _ _ _ _ _ _ _ _ _ _ _ _ _ _ _ _ _ _ _ _ _ _ _ _ _ _ _ _ _ _ _ _ _ _ _ _ _ _ _ _ _ _ _ _ _ _ _ _ _ _ _ _ _ _ _ _ _ _ _ _ _ _ _ _ _ _ _ _ _ _ _ _ _]
      event Timeout {
        n37 = event-data() -> ()  [unwired: 3 out]
      }
      event Pane Size {
        n38 = event-data() -> ()  [unwired: 7 out]
        n39 = control-ref of="Board Tab"() -> (w535:refnum<vi>)
        n40 = control-ref of="This VI"() -> (w536:refnum<vi>)
        n41 = call "CRYAlign Steps VI Center.vi"("Tab2"=w535, "Input/Output"=TRUE ("Preview"), "VIRef"=w536) -> ()  [unwired: 1 in, 8 out]
      }
      event "Load...": Value Change {
        n42 = event-data() -> ("CtlRef"=w538:refnum<vi>)  [unwired: 6 out]
        n43 = property class="Bool (strict)"(reference=w538, "Value"=FALSE) -> ()  [unwired: 1 in, 2 out]
        n44 = local read "Load Test"() -> (w540:bool)
        n45 = case shown="False" w540 {
          frame True {
          }
          frame False {
            n46 = global read "CRYMainGlobal.vi" "Steps path"() -> (w546:path)
            n47 = local read "Proper VI No"() -> (w542:i32)
            n48 = Build Path(base path=w546, name or relative path="CRYAnalysis") -> (appended path=w545:path)
            n49 = call "CRYStep Read.vi"("Category Name"="Analysis" ("Step File Name"), "Proper VI No"=w542, "Step File Path"=w545) -> ("status"=w544:bool, "selected path"=w541:path, "Flatten Step"=w543:string)  [unwired: 1 in, 3 out]
            n50 = case shown="True" w544 {
              tunnel: w543 -> [_ w550]
              tunnel: w542 -> [_ w551]
              tunnel: w541 -> [_ w549]
              frame False {
              }
              frame True {
                n51 = call "CRYUnflatten Analysis.vi"("Unflatten Analysis"=w550) -> ("Error?"=w552:bool, "Analysis"=w553:T1)  [unwired: 1 in, 8 out]
                n52 = case shown="False" w552 {
                  tunnel: w553 -> [w559 _]
                  tunnel: w551 -> [w556 _]
                  tunnel: w550 -> [w555 _]
                  tunnel: w549 -> [w554 _]
                  frame False {
                    n53 = flat-sequence {
                      tunnel: w559 -> [w572]
                      tunnel: [w572] -> w557
                      tunnel: w556 -> [w569]
                      tunnel: w555 -> [w568]
                      tunnel: w554 -> [w567]
                      tunnel: [w573] -> w558
                      tunnel: w557 -> [w573]
                      tunnel: w558 -> [w575]
                      frame #0 {
                        n54 = Strip Path(path=w567) -> (name=w562:string)  [unwired: 1 out]
                        n55 = Reverse String(1:w562) -> (0:w564:string)
                        n56 = Match Pattern(string=w564, regular expression="[.]") -> (after substring=w565:string)  [unwired: 4 out]
                        n57 = Reverse String(1:w565) -> (0:w561:string)
                        n58 = call "CRYPreUpdate Sequence.vi"("EventName"="Load", "StepName Arg3"=w561, "Proper VI No"=w569, "Project View Step Name Identifier Arg1"="", "Step flattened Arg2"=w568, "AllChangeFlg"=TRUE ("Name/Identifier")) -> ()  [unwired: 10 in]
                        n59 = local write "Mode"("Load" ("Mode")) -> ()
                        n60 = local write "Analysis"(w572) -> ()
                      }
                      frame #1 {
                        n61 = local write "Load Test"(TRUE ("Load Test")) -> ()
                      }
                      frame #2 {
                        n62 = disable-structure shown="Disabled" {
                          disable-tunnel: w575 -> [w576 _]
                          frame Disabled {
                            n63 = property on="Analysis" class="Clust (strict)"("Val(Sgnl)"=w576) -> ()  [unwired: 2 in, 2 out]
                          }
                          frame Enabled {
                          }
                        }
                      }
                    }
                  }
                  frame True {
                  }
                }
              }
            }
          }
        }
      }
      event "Save As...": Value Change {
        n64 = event-data() -> ("CtlRef"=w577:refnum<vi>)  [unwired: 6 out]
        n65 = property class="Bool (strict)"(reference=w577, "Value"=FALSE) -> ()  [unwired: 1 in, 2 out]
        n66 = local read "Analysis"() -> (w579:T1)
        n67 = call "CRYFlatten Analysis.vi"("Analysis"=w579) -> ("Analysis flattened"=w580:string)  [unwired: 10 out]
        n68 = global read "CRYMainGlobal.vi" "Steps path"() -> (w582:path)
        n69 = local read "Proper VI No"() -> (w587:i32)
        n70 = Build Path(base path=w582, name or relative path="CRYAnalysis") -> (appended path=w581:path)
        n71 = call "CRYStep Write.vi"("StepIdentifier"="", "Default"=FALSE, "Proper VI No"=w587, "Category Name"="Analysis" ("Step File Name"), "Step File Path"=w581, "Step flattened"=w580, "Step File Name"="Analysis") -> ()  [unwired: 1 in, 4 out]
      }
      event "Revert": Value Change {
        n72 = event-data() -> ("CtlRef"=w590:refnum<vi>)  [unwired: 6 out]
        n73 = property class="Bool (strict)"(reference=w590, "Value"=FALSE) -> ()  [unwired: 1 in, 2 out]
        n74 = flat-sequence {
          frame #0 {
            n75 = local read "Analysis Bk"() -> (w591:T1)
            n76 = local write "Mode"("Revert" ("Mode")) -> ()
            n77 = local write "Analysis"(w591) -> ()
          }
          frame #1 {
            n78 = local write "Load Test"(TRUE ("Visible")) -> ()
          }
        }
      }
      event Panel Close {
        n79 = event-data() -> ()  [unwired: 5 out]
        n80 = control-ref of="This VI"() -> (w595:refnum<vi>)
        n81 = local write "Cancel"(TRUE ("Cancel")) -> ()
        n82 = call "CRYWork Before Step Close.vi"("StepVI Ref"=w595) -> ()  [unwired: 11 in]
      }
      event "CurLibChange": Value Change {
        n83 = event-data() -> ()  [unwired: 7 out]
        n84 = flat-sequence {
          tunnel: [w601] -> w598
          tunnel: [w600] -> w597
          tunnel: w596 -> [w599]
          frame #0 {
            n85 = call "CRYGet Upper Step Data.vi"("Type In"=enum16{"Curves", "Values", "Results", "WFM"}."Values", "No.VI"=w599) -> ("Value array"=w602:T5)  [unwired: 9 out]
            n86 = call "CRYGet Upper Step Data.vi"("Type In"=enum16{"Curves", "Values", "Results", "WFM"}."WFM" ("Type"), "No.VI"=w599) -> ("Waveform Array"=w604:T12)  [unwired: 6 in, 3 out]
            n87 = for {
              tunnel: w602 -> [w609] mode=indexing
              tunnel: [w608] -> w601 mode=indexing
              n88 = Unbundle By Name(w609) -> ("Name"=w608:string)
            }
            n89 = for {
              tunnel: w604 -> [w607] mode=indexing
              tunnel: [w606] -> w600 mode=indexing
              n90 = Unbundle By Name(w607) -> ("Name"=w606:string)
            }
            n91 = property on="LR" class="Ring (strict)"("Strings []"=w601) -> ()  [unwired: 2 in, 2 out]
            n92 = property on="Waveforms Out" class="Ring (strict)"("Strings []"=w600) -> ()  [unwired: 2 in, 2 out]
            n93 = property on="Waveforms In" class="Ring (strict)"("Strings []"=w600) -> ()  [unwired: 2 in, 2 out]
          }
        }
        n94 = flat-sequence {
          tunnel: w598 -> [w615]
          tunnel: w597 -> [w613]
          frame #0 {
            n95 = local read "Analysis"() -> (w614:T1)
            n96 = Unbundle By Name(w614) -> ("Waveform Out"=w612:string, "Waveform In"=w611:string, "unLabel"=w610:string)
            n97 = Search 1D Array(1D array=w615, element=w610) -> (index of element=w618:i32)  [unwired: 1 out]
            n98 = Search 1D Array(1D array=w613, element=w611) -> (index of element=w626:i32)  [unwired: 1 out]
            n99 = Search 1D Array(1D array=w613, element=w612) -> (index of element=w624:i32)  [unwired: 1 out]
            n100 = Not Equal?(x=w618, y=-1) -> (x != y?=w620:bool)
            n101 = Less Than 0?(x=w626) -> (x < 0?=w628:bool)
            n102 = Less Than 0?(x=w624) -> (x < 0?=w623:bool)
            n103 = Select(t=w618, s=w620, f=0) -> (s? t:f=w617:i32)
            n104 = Select(t=0 ("index of element"), s=w628, f=w626) -> (s? t:f=w622:i32)
            n105 = Select(t=0 ("index of element"), s=w623, f=w624) -> (s? t:f=w621:i32)
            n106 = local write "LR"(w617) -> ()
            n107 = property on="Waveforms In" class="Ring (strict)"("Val(Sgnl)"=w622) -> ()  [unwired: 2 in, 2 out]
            n108 = property on="Waveforms Out" class="Ring (strict)"("Val(Sgnl)"=w621) -> ()  [unwired: 2 in, 2 out]
          }
        }
      }
      event "Algorithm": Value Change {
        n109 = event-data() -> ("NewVal"=w630:u16)  [unwired: 6 out]
        n110 = case shown="5" w630 {
          tunnel: [u16 0 ("Algorithm") u16 1 ("Algorithm") u16 2 ("Algorithm") u16 3 ("Algorithm") u16 4 ("Algorithm") u16 5 ("Algorithm") u16 6 ("Algorithm")] -> w629
          frame 0, Default {
          }
          frame 1 {
          }
          frame 2 {
          }
          frame 3 {
          }
          frame 4 {
          }
          frame 5 {
          }
          frame 6 {
          }
        }
        n111 = flat-sequence {
          tunnel: w629 -> [w633]
          frame #0 {
            n112 = local read "Analysis"() -> (w634:T1)
            n113 = Bundle By Name(cluster=w634, "Algorithm"=w633) -> (w632:T1)
            n114 = local write "Analysis"(w632) -> ()
          }
          frame #1 {
            n115 = property on="CurveUpdate" class="Bool (strict)"("Val(Sgnl)"=TRUE ("Value (Signaling)")) -> ()  [unwired: 2 in, 2 out]
          }
        }
        n116 = property on="Visible Update" class="Bool (strict)"("Val(Sgnl)"=TRUE ("Value (Signaling)")) -> ()  [unwired: 2 in, 2 out]
      }
      event "Visible Update": Value Change {
        n117 = event-data() -> ("CtlRef"=w646:refnum<vi>)  [unwired: 6 out]
        n118 = property class="Bool (strict)"(reference=w646, "Value"=FALSE) -> ()  [unwired: 1 in, 2 out]
        n119 = property on="Advanced View" class="Bool (strict)"() -> ("Value"=w644:bool)  [unwired: 2 in, 2 out]
        n120 = property on="Algorithm" class="Ring (strict)"() -> ("Value"=w643:u16)  [unwired: 2 in, 2 out]
        n121 = stacked-sequence {
          tunnel: w644 -> [w678 w946]
          tunnel: w643 -> [w661 w959]
          frame #0 {
            # "Time"
            n122 = case shown="True" w678 {
              tunnel: w661 -> [w709 w821]
              tunnel: [w692 TRUE ("Visible")] -> w677
              tunnel: [w701 w819] -> w653
              tunnel: [w700 w818] -> w676
              tunnel: [w699 w817] -> w675
              tunnel: [w698 w816] -> w674
              tunnel: [w697 w815] -> w673
              tunnel: [w696 w814] -> w672
              tunnel: [w708 w813] -> w671
              tunnel: [w705 w812] -> w670
              tunnel: [w704 w811] -> w669
              tunnel: [w707 w810] -> w668
              tunnel: [w706 w809] -> w667
              tunnel: [w703 w808] -> w666
              tunnel: [w695 w807] -> w665
              tunnel: [w694 w806] -> w664
              tunnel: [w693 w805] -> w663
              tunnel: [w702 w804] -> w662
              tunnel: [w692 w803] -> w655
              frame False {
                w692 = FALSE ("Visible")
                n123 = case shown="4" w709 {
                  tunnel: [_ w724 _ _ w762 w774 w790] -> w708
                  tunnel: [_ w724 _ _ w762 w774 w790] -> w707
                  tunnel: [_ w724 _ _ w762 w774 w790] -> w706
                  tunnel: [_ w723 _ _ w762 w772 w788] -> w705
                  tunnel: [_ w723 _ _ w762 w772 w788] -> w704
                  tunnel: [_ w723 _ _ w762 w773 w788] -> w703
                  tunnel: [_ w723 _ _ w762 w773 w788] -> w702
                  tunnel: [_ w722 _ _ w763 w772 w789] -> w701
                  tunnel: [_ w722 _ _ w763 w772 w789] -> w700
                  tunnel: [_ w722 _ _ w763 w772 w789] -> w699
                  tunnel: [_ w722 _ _ w763 w772 w789] -> w698
                  tunnel: [_ w722 _ _ w762 w772 w789] -> w697
                  tunnel: [_ w722 _ _ w762 w772 w789] -> w696
                  tunnel: [_ w722 _ _ w762 w772 w789] -> w695
                  tunnel: [_ w722 _ _ w762 w772 w789] -> w694
                  tunnel: [_ w722 _ _ w762 w772 w789] -> w693
                  frame 0, Default {
                    n124 = property on="Main Tab" class="TabCtl (strict)"() -> ("Pages"=w710:refnum<vi>[])  [unwired: 2 in, 2 out]
                    n125 = for {
                      N: 8 -> [_]
                      tunnel: w710 -> [w715]
                      i -> [w714]
                      n126 = Index Array(array=w715, index=w714) -> (element=w712:refnum<vi>)
                      n127 = case shown="0..2, 5, 6" w714 {
                        selector: w714 -> [_ w719]
                        tunnel: [T8."Page Enabled" ("Page Enabled State") T8."Page Disabled & Grayed" ("Page Enabled State")] -> w713
                        frame Default {
                        }
                        frame 0..2, 5, 6 {
                          n128 = property on="Main Tab" class="TabCtl (strict)"() -> ("Value"=w720:T3)  [unwired: 2 in, 2 out]
                          n129 = Equal?(x=w720, y=w719) -> (x = y?=w718:bool)
                          n130 = case shown="True" w718 {
                            frame False {
                            }
                            frame True {
                              n131 = property on="Main Tab" class="TabCtl (strict)"("Value"=T9."Waveforms" ("Tab")) -> ()  [unwired: 2 in, 2 out]
                            }
                          }
                        }
                      }
                      n132 = property class="Page"(reference=w712, "PageEnb"=w713) -> ()  [unwired: 1 in, 2 out]
                    }
                  }
                  frame 1 {
                    w722 = FALSE ("Visible")
                    w723 = FALSE ("Visible")
                    w724 = TRUE ("Visible")
                    w725 = u8 2 ("Disabled")
                    n133 = property on="Main Tab" class="TabCtl (strict)"() -> ("Pages"=w726:refnum<vi>[])  [unwired: 2 in, 2 out]
                    n134 = for {
                      N: 8 -> [_]
                      tunnel: w726 -> [w731]
                      i -> [w730]
                      n135 = Index Array(array=w731, index=w730) -> (element=w728:refnum<vi>)
                      n136 = case shown="0..2, 5, 7" w730 {
                        selector: w730 -> [_ w735]
                        tunnel: [T8."Page Enabled" ("Page Enabled State") T8."Page Disabled & Grayed" ("Page Enabled State")] -> w729
                        frame Default {
                        }
                        frame 0..2, 5, 7 {
                          n137 = property on="Main Tab" class="TabCtl (strict)"() -> ("Value"=w736:T3)  [unwired: 2 in, 2 out]
                          n138 = Equal?(x=w736, y=w735) -> (x = y?=w734:bool)
                          n139 = case shown="True" w734 {
                            frame False {
                            }
                            frame True {
                              n140 = property on="Main Tab" class="TabCtl (strict)"("Value"=T9."Waveforms" ("Tab")) -> ()  [unwired: 2 in, 2 out]
                            }
                          }
                        }
                      }
                      n141 = property class="Page"(reference=w728, "PageEnb"=w729) -> ()  [unwired: 1 in, 2 out]
                    }
                    n142 = property on="Auto-Spectrum(Stimulus)*" class="Bool (strict)"("Disabled"=w725) -> ()  [unwired: 2 in, 2 out]
                    n143 = property on="Response Measurement1" class="Slide (strict)"("Disabled"=w725) -> ()  [unwired: 2 in, 2 out]
                  }
                  frame 2 {
                    n144 = property on="Main Tab" class="TabCtl (strict)"() -> ("Pages"=w738:refnum<vi>[])  [unwired: 2 in, 2 out]
                    n145 = for {
                      N: 8 -> [_]
                      tunnel: w738 -> [w743]
                      i -> [w742]
                      n146 = Index Array(array=w743, index=w742) -> (element=w740:refnum<vi>)
                      n147 = case shown="0..2, 6" w742 {
                        selector: w742 -> [_ w747]
                        tunnel: [T8."Page Enabled" ("Page Enabled State") T8."Page Disabled & Grayed" ("Page Enabled State")] -> w741
                        frame Default {
                        }
                        frame 0..2, 6 {
                          n148 = property on="Main Tab" class="TabCtl (strict)"() -> ("Value"=w748:T3)  [unwired: 2 in, 2 out]
                          n149 = Equal?(x=w748, y=w747) -> (x = y?=w746:bool)
                          n150 = case shown="True" w746 {
                            frame False {
                            }
                            frame True {
                              n151 = property on="Main Tab" class="TabCtl (strict)"("Value"=T9."Waveforms" ("Tab")) -> ()  [unwired: 2 in, 2 out]
                            }
                          }
                        }
                      }
                      n152 = property class="Page"(reference=w740, "PageEnb"=w741) -> ()  [unwired: 1 in, 2 out]
                    }
                  }
                  frame 3 {
                    n153 = property on="Main Tab" class="TabCtl (strict)"() -> ("Pages"=w750:refnum<vi>[])  [unwired: 2 in, 2 out]
                    n154 = for {
                      N: 8 -> [_]
                      tunnel: w750 -> [w755]
                      i -> [w754]
                      n155 = Index Array(array=w755, index=w754) -> (element=w752:refnum<vi>)
                      n156 = case shown="0..2, 5, 6" w754 {
                        selector: w754 -> [_ w759]
                        tunnel: [T8."Page Enabled" ("Page Enabled State") T8."Page Disabled & Grayed" ("Page Enabled State")] -> w753
                        frame Default {
                        }
                        frame 0..2, 5, 6 {
                          n157 = property on="Main Tab" class="TabCtl (strict)"() -> ("Value"=w760:T3)  [unwired: 2 in, 2 out]
                          n158 = Equal?(x=w760, y=w759) -> (x = y?=w758:bool)
                          n159 = case shown="True" w758 {
                            frame False {
                            }
                            frame True {
                              n160 = property on="Main Tab" class="TabCtl (strict)"("Value"=T9."Waveforms" ("Tab")) -> ()  [unwired: 2 in, 2 out]
                            }
                          }
                        }
                      }
                      n161 = property class="Page"(reference=w752, "PageEnb"=w753) -> ()  [unwired: 1 in, 2 out]
                    }
                  }
                  frame 4 {
                    w762 = FALSE ("Visible")
                    w763 = TRUE ("Visible")
                    n162 = property on="Main Tab" class="TabCtl (strict)"() -> ("Pages"=w764:refnum<vi>[])  [unwired: 2 in, 2 out]
                    n163 = for {
                      N: 8 -> [_]
                      tunnel: w764 -> [w769]
                      i -> [w768]
                      n164 = Index Array(array=w769, index=w768) -> (element=w766:refnum<vi>)
                      n165 = case shown="Default" w768 {
                        tunnel: [T8."Page Enabled" ("Page Enabled State") T8."Page Disabled & Grayed" ("Page Enabled State")] -> w767
                        frame Default {
                        }
                        frame 0, 1 {
                        }
                      }
                      n166 = property class="Page"(reference=w766, "PageEnb"=w767) -> ()  [unwired: 1 in, 2 out]
                    }
                  }
                  frame 5 {
                    w772 = FALSE ("Visible")
                    w773 = FALSE ("Visible")
                    w774 = TRUE ("Visible")
                    n167 = property on="Main Tab" class="TabCtl (strict)"() -> ("Pages"=w776:refnum<vi>[])  [unwired: 2 in, 2 out]
                    n168 = for {
                      N: 8 -> [_]
                      tunnel: w776 -> [w781]
                      i -> [w780]
                      n169 = Index Array(array=w781, index=w780) -> (element=w778:refnum<vi>)
                      n170 = case shown="0..2, 5" w780 {
                        selector: w780 -> [_ w785]
                        tunnel: [T8."Page Enabled" ("Page Enabled State") T8."Page Disabled & Grayed" ("Page Enabled State")] -> w779
                        frame Default {
                        }
                        frame 0..2, 5 {
                          n171 = property on="Main Tab" class="TabCtl (strict)"() -> ("Value"=w786:T3)  [unwired: 2 in, 2 out]
                          n172 = Equal?(x=w786, y=w785) -> (x = y?=w784:bool)
                          n173 = case shown="True" w784 {
                            frame False {
                            }
                            frame True {
                              n174 = property on="Main Tab" class="TabCtl (strict)"("Value"=T9."Waveforms" ("Tab")) -> ()  [unwired: 2 in, 2 out]
                            }
                          }
                        }
                      }
                      n175 = property class="Page"(reference=w778, "PageEnb"=w779) -> ()  [unwired: 1 in, 2 out]
                    }
                    n176 = property on="Auto-Spectrum(Stimulus)*" class="Bool (strict)"("Disabled"=u8 0) -> ()  [unwired: 2 in, 2 out]
                  }
                  frame 6 {
                    w789 = FALSE ("Visible")
                    w788 = FALSE ("Visible")
                    w790 = TRUE ("Visible")
                    n177 = property on="Main Tab" class="TabCtl (strict)"() -> ("Pages"=w791:refnum<vi>[])  [unwired: 2 in, 2 out]
                    n178 = for {
                      N: 8 -> [_]
                      tunnel: w791 -> [w796]
                      i -> [w795]
                      n179 = Index Array(array=w796, index=w795) -> (element=w793:refnum<vi>)
                      n180 = case shown="1, 2, 5" w795 {
                        selector: w795 -> [_ w800]
                        tunnel: [T8."Page Enabled" ("Page Enabled State") T8."Page Disabled & Grayed" ("Page Enabled State")] -> w794
                        frame Default {
                        }
                        frame 1, 2, 5 {
                          n181 = property on="Main Tab" class="TabCtl (strict)"() -> ("Value"=w801:T3)  [unwired: 2 in, 2 out]
                          n182 = Equal?(x=w801, y=w800) -> (x = y?=w799:bool)
                          n183 = case shown="True" w799 {
                            frame False {
                            }
                            frame True {
                              n184 = property on="Main Tab" class="TabCtl (strict)"("Value"=T9."Waveforms" ("Tab")) -> ()  [unwired: 2 in, 2 out]
                            }
                          }
                        }
                      }
                      n185 = property class="Page"(reference=w793, "PageEnb"=w794) -> ()  [unwired: 1 in, 2 out]
                    }
                  }
                }
              }
              frame True {
                n186 = case shown="6" w821 {
                  tunnel: [w824 w839 w857 w872 w893 w904 w929] -> w819
                  tunnel: [w824 w839 w857 w872 w893 w904 w929] -> w818
                  tunnel: [w824 w839 w857 w872 w893 w904 w929] -> w817
                  tunnel: [w824 w839 w857 w872 w893 w904 w929] -> w816
                  tunnel: [w824 w839 w857 w872 w893 w904 w926] -> w815
                  tunnel: [w824 w839 w857 w872 w893 w904 w929] -> w814
                  tunnel: [w824 w840 w857 w872 w892 w905 w930] -> w813
                  tunnel: [w824 w840 w858 TRUE ("Visible") w892 w905 w930] -> w812
                  tunnel: [w824 w840 w857 w873 w892 w905 w930] -> w811
                  tunnel: [w824 w840 w857 w873 w892 w905 w930] -> w810
                  tunnel: [w824 w840 w857 w873 w892 w905 w930] -> w809
                  tunnel: [w824 w840 w857 w873 w892 w905 w930] -> w808
                  tunnel: [w824 w839 w857 w872 w892 w904 w927] -> w807
                  tunnel: [w824 w839 w857 w872 w892 w904 w927] -> w806
                  tunnel: [w824 w839 w857 w872 w892 w904 w926] -> w805
                  tunnel: [TRUE ("Visible") FALSE ("Visible") w858 TRUE ("Visible") w892 FALSE ("Visible") FALSE ("Visible")] -> w804
                  tunnel: [w822 w838 w856 w871 w888 w903 w920] -> w803
                  frame 0, Default {
                    w824 = FALSE ("Visible")
                    n187 = property on="Main Tab" class="TabCtl (strict)"() -> ("Pages"=w825:refnum<vi>[])  [unwired: 2 in, 2 out]
                    n188 = for {
                      N: 8 -> [_]
                      tunnel: w825 -> [w830]
                      i -> [w829]
                      n189 = Index Array(array=w830, index=w829) -> (element=w827:refnum<vi>)
                      n190 = case shown="2, 5" w829 {
                        selector: w829 -> [_ w834]
                        tunnel: [T8."Page Enabled" ("Page Enabled State") T8."Page Disabled & Grayed" ("Page Enabled State")] -> w828
                        frame Default {
                        }
                        frame 2, 5 {
                          n191 = property on="Main Tab" class="TabCtl (strict)"() -> ("Value"=w835:T3)  [unwired: 2 in, 2 out]
                          n192 = Equal?(x=w835, y=w834) -> (x = y?=w833:bool)
                          n193 = case shown="True" w833 {
                            frame False {
                            }
                            frame True {
                              n194 = property on="Main Tab" class="TabCtl (strict)"("Value"=T9."Waveforms" ("Tab")) -> ()  [unwired: 2 in, 2 out]
                            }
                          }
                        }
                      }
                      n195 = property class="Page"(reference=w827, "PageEnb"=w828) -> ()  [unwired: 1 in, 2 out]
                    }
                    n196 = local read "Envelope?"() -> (w822:bool)
                  }
                  frame 1 {
                    w839 = FALSE ("Visible")
                    w840 = TRUE ("Visible")
                    w843 = u16 1 items=["Complex", "Power"] ("Averaging")
                    w842 = u8 2 ("Disabled")
                    n197 = property on="Main Tab" class="TabCtl (strict)"() -> ("Pages"=w844:refnum<vi>[])  [unwired: 2 in, 2 out]
                    n198 = for {
                      N: 8 -> [_]
                      tunnel: w844 -> [w849]
                      i -> [w848]
                      n199 = Index Array(array=w849, index=w848) -> (element=w846:refnum<vi>)
                      n200 = case shown="5, 7" w848 {
                        selector: w848 -> [_ w853]
                        tunnel: [T8."Page Enabled" ("Page Enabled State") T8."Page Disabled & Grayed" ("Page Enabled State")] -> w847
                        frame Default {
                        }
                        frame 5, 7 {
                          n201 = property on="Main Tab" class="TabCtl (strict)"() -> ("Value"=w854:T3)  [unwired: 2 in, 2 out]
                          n202 = Equal?(x=w854, y=w853) -> (x = y?=w852:bool)
                          n203 = case shown="True" w852 {
                            frame False {
                            }
                            frame True {
                              n204 = property on="Main Tab" class="TabCtl (strict)"("Value"=T9."Waveforms" ("Tab")) -> ()  [unwired: 2 in, 2 out]
                            }
                          }
                        }
                      }
                      n205 = property class="Page"(reference=w846, "PageEnb"=w847) -> ()  [unwired: 1 in, 2 out]
                    }
                    n206 = property on="Auto-Spectrum(Response)*" class="Bool (strict)"("Disabled"=w842) -> ()  [unwired: 2 in, 2 out]
                    n207 = property on="Averaging1" class="Slide (strict)"("Disabled"=w842) -> ()  [unwired: 2 in, 2 out]
                    n208 = property on="Response Measurement1" class="Slide (strict)"("Disabled"=w842) -> ()  [unwired: 2 in, 2 out]
                    n209 = property on="Auto-Spectrum(Response)*" class="Bool (strict)"("Value"=TRUE ("Auto-Spectrum(Response)*")) -> ()  [unwired: 2 in, 2 out]
                    n210 = property on="Averaging1" class="Slide (strict)"("Value"=w843) -> ()  [unwired: 2 in, 2 out]
                    n211 = local read "Envelope?"() -> (w838:bool)
                  }
                  frame 2 {
                    w857 = FALSE ("Visible")
                    w858 = TRUE ("Visible")
                    n212 = property on="Main Tab" class="TabCtl (strict)"() -> ("Pages"=w859:refnum<vi>[])  [unwired: 2 in, 2 out]
                    n213 = for {
                      N: 8 -> [_]
                      tunnel: w859 -> [w864]
                      i -> [w863]
                      n214 = Index Array(array=w864, index=w863) -> (element=w861:refnum<vi>)
                      n215 = case shown="2" w863 {
                        selector: w863 -> [_ w868]
                        tunnel: [T8."Page Enabled" ("Page Enabled State") T8."Page Disabled & Grayed" ("Page Enabled State")] -> w862
                        frame Default {
                        }
                        frame 2 {
                          n216 = property on="Main Tab" class="TabCtl (strict)"() -> ("Value"=w869:T3)  [unwired: 2 in, 2 out]
                          n217 = Equal?(x=w869, y=w868) -> (x = y?=w867:bool)
                          n218 = case shown="True" w867 {
                            frame False {
                            }
                            frame True {
                              n219 = property on="Main Tab" class="TabCtl (strict)"("Value"=T9."Waveforms" ("Tab")) -> ()  [unwired: 2 in, 2 out]
                            }
                          }
                        }
                      }
                      n220 = property class="Page"(reference=w861, "PageEnb"=w862) -> ()  [unwired: 1 in, 2 out]
                    }
                    n221 = local read "Envelope?"() -> (w856:bool)
                  }
                  frame 3 {
                    w872 = FALSE ("Visible")
                    w873 = FALSE ("Visible")
                    n222 = property on="Main Tab" class="TabCtl (strict)"() -> ("Pages"=w876:refnum<vi>[])  [unwired: 2 in, 2 out]
                    n223 = for {
                      N: 8 -> [_]
                      tunnel: w876 -> [w881]
                      i -> [w880]
                      n224 = Index Array(array=w881, index=w880) -> (element=w878:refnum<vi>)
                      n225 = case shown="2, 5" w880 {
                        selector: w880 -> [_ w885]
                        tunnel: [T8."Page Enabled" ("Page Enabled State") T8."Page Disabled & Grayed" ("Page Enabled State")] -> w879
                        frame Default {
                        }
                        frame 2, 5 {
                          n226 = property on="Main Tab" class="TabCtl (strict)"() -> ("Value"=w886:T3)  [unwired: 2 in, 2 out]
                          n227 = Equal?(x=w886, y=w885) -> (x = y?=w884:bool)
                          n228 = case shown="True" w884 {
                            frame False {
                            }
                            frame True {
                              n229 = property on="Main Tab" class="TabCtl (strict)"("Value"=T9."Waveforms" ("Tab")) -> ()  [unwired: 2 in, 2 out]
                            }
                          }
                        }
                      }
                      n230 = property class="Page"(reference=w878, "PageEnb"=w879) -> ()  [unwired: 1 in, 2 out]
                    }
                    n231 = local read "Envelope?"() -> (w871:bool)
                  }
                  frame 4 {
                    w892 = FALSE ("Visible")
                    w893 = TRUE ("Visible")
                    n232 = property on="Main Tab" class="TabCtl (strict)"() -> ("Pages"=w894:refnum<vi>[])  [unwired: 2 in, 2 out]
                    n233 = for {
                      N: 8 -> [_]
                      tunnel: w894 -> [w899]
                      i -> [w898]
                      n234 = Index Array(array=w899, index=w898) -> (element=w896:refnum<vi>)
                      n235 = case shown="Default" w898 {
                        tunnel: [T8."Page Enabled" ("Page Enabled State") T8."Page Enabled" ("Page Enabled State")] -> w897
                        frame Default {
                        }
                        frame 2 {
                        }
                      }
                      n236 = property class="Page"(reference=w896, "PageEnb"=w897) -> ()  [unwired: 1 in, 2 out]
                    }
                    n237 = local read "Deconvolved Response"() -> (w890:bool)
                    n238 = local read "impulse resp?"() -> (w889:bool)
                    n239 = local read "Envelope?"() -> (w891:bool)
                    n240 = Compound Arithmetic op=OR(w889, w890, w891) -> (w888:bool)
                  }
                  frame 5 {
                    w904 = FALSE ("Visible")
                    w905 = TRUE ("Visible")
                    w902 = u8 0 ("Disabled")
                    n241 = property on="Main Tab" class="TabCtl (strict)"() -> ("Pages"=w907:refnum<vi>[])  [unwired: 2 in, 2 out]
                    n242 = for {
                      N: 8 -> [_]
                      tunnel: w907 -> [w912]
                      i -> [w911]
                      n243 = Index Array(array=w912, index=w911) -> (element=w909:refnum<vi>)
                      n244 = case shown="5" w911 {
                        selector: w911 -> [_ w916]
                        tunnel: [T8."Page Enabled" ("Page Enabled State") T8."Page Disabled & Grayed" ("Page Enabled State")] -> w910
                        frame Default {
                        }
                        frame 5 {
                          n245 = property on="Main Tab" class="TabCtl (strict)"() -> ("Value"=w917:T3)  [unwired: 2 in, 2 out]
                          n246 = Equal?(x=w917, y=w916) -> (x = y?=w915:bool)
                          n247 = case shown="True" w915 {
                            frame False {
                            }
                            frame True {
                              n248 = property on="Main Tab" class="TabCtl (strict)"("Value"=T9."Waveforms" ("Tab")) -> ()  [unwired: 2 in, 2 out]
                            }
                          }
                        }
                      }
                      n249 = property class="Page"(reference=w909, "PageEnb"=w910) -> ()  [unwired: 1 in, 2 out]
                    }
                    n250 = property on="Averaging1" class="Slide (strict)"("Disabled"=w902) -> ()  [unwired: 2 in, 2 out]
                    n251 = property on="Auto-Spectrum(Stimulus)*" class="Bool (strict)"("Disabled"=w902) -> ()  [unwired: 2 in, 2 out]
                    n252 = property on="Auto-Spectrum(Response)*" class="Bool (strict)"("Disabled"=w902) -> ()  [unwired: 2 in, 2 out]
                    n253 = local read "Envelope?"() -> (w903:bool)
                  }
                  frame 6 {
                    w919 = u8 0 ("Disabled")
                    w929 = FALSE ("Visible")
                    w930 = TRUE ("Visible")
                    n254 = property on="Main Tab" class="TabCtl (strict)"() -> ("Pages"=w932:refnum<vi>[])  [unwired: 2 in, 2 out]
                    n255 = local read "Auto-Correlation(Stimulus)"() -> (w923:bool)
                    n256 = local read "Auto-Correlation(Response)"() -> (w922:bool)
                    n257 = local read "impulse resp?"() -> (w924:bool)
                    n258 = local read "Cross-Correlation"() -> (w921:bool)
                    n259 = local read "Envelope?"() -> (w925:bool)
                    n260 = for {
                      N: 8 -> [_]
                      tunnel: w932 -> [w940]
                      i -> [w939]
                      n261 = Index Array(array=w940, index=w939) -> (element=w937:refnum<vi>)
                      n262 = case shown="Default" w939 {
                        tunnel: [T8."Page Enabled" ("Page Enabled State") T8."Page Disabled & Grayed" ("Page Enabled State")] -> w938
                        frame Default {
                        }
                        frame 5 {
                        }
                      }
                      n263 = property class="Page"(reference=w937, "PageEnb"=w938) -> ()  [unwired: 1 in, 2 out]
                    }
                    n264 = Compound Arithmetic op=OR(w924, w925, w923, w922, w921) -> (w920:bool)
                    n265 = property on="Averaging1" class="Slide (strict)"("Disabled"=w919) -> ()  [unwired: 2 in, 2 out]
                    n266 = property on="Auto-Spectrum(Stimulus)*" class="Bool (strict)"("Disabled"=w919) -> ()  [unwired: 2 in, 2 out]
                    n267 = property on="Auto-Spectrum(Response)*" class="Bool (strict)"("Disabled"=w919) -> ()  [unwired: 2 in, 2 out]
                    n268 = local read "Averaging1"() -> (w928:u16)
                    n269 = case shown="1" w928 {
                      tunnel: [w934 TRUE ("Visible")] -> w927
                      tunnel: [w934 FALSE ("Visible")] -> w926
                      frame 0, Default {
                        w934 = TRUE ("Visible")
                      }
                      frame 1 {
                      }
                    }
                  }
                }
              }
            }
            n270 = property on="Start Time(s)" class="DigNum (strict)"("Visible"=w653) -> ()  [unwired: 2 in, 2 out]
            n271 = property on="StopTime(s)" class="DigNum (strict)"("Visible"=w675) -> ()  [unwired: 2 in, 2 out]
            n272 = property on="Windowed Resolution(Hz)" class="DigNum (strict)"("Visible"=w674) -> ()  [unwired: 2 in, 2 out]
            n273 = property on="impulse resp?" class="Bool (strict)"("Visible"=w673) -> ()  [unwired: 2 in, 2 out]
            n274 = property on="Deconvolved Response" class="Bool (strict)"("Visible"=w672) -> ()  [unwired: 2 in, 2 out]
            n275 = property on="Weighting" class="Ring (strict)"("Visible"=w670) -> ()  [unwired: 2 in, 2 out]
            n276 = property on="Default Overlap" class="Bool (strict)"("Visible"=w669) -> ()  [unwired: 2 in, 2 out]
            n277 = property on="Record Length (s)" class="DigNum (strict)"("Visible"=w668) -> ()  [unwired: 2 in, 2 out]
            n278 = property on="No.of FFTs" class="DigNum (strict)"("Visible"=w667) -> ()  [unwired: 2 in, 2 out]
            n279 = property on="Overlap(%)" class="DigNum (strict)"("Visible"=w666) -> ()  [unwired: 2 in, 2 out]
            n280 = property on="Discard Cycles" class="DigNum (strict)"("Visible"=w662) -> ()  [unwired: 2 in, 2 out]
            n281 = property on="Impedance" class="Bool (strict)"() -> ("Value"=w652:bool)  [unwired: 2 in, 2 out]
            n282 = local read "Envelope?"() -> (w654:bool)
            n283 = property on="TSR Window Type" class="Ring (strict)"("Visible"=w653) -> ()  [unwired: 2 in, 2 out]
            n284 = case shown="True" w652 {
              tunnel: w661 -> [w682 w689]
              tunnel: [w681 u8 2 ("Disabled")] -> w660
              tunnel: [w680 w687] -> w659
              frame False {
                n285 = case shown="0, Default" w682 {
                  tunnel: [u8 0 ("Disabled") u8 2 ("Disabled")] -> w681
                  tunnel: [w683 w685] -> w680
                  frame 0, Default {
                    n286 = property on="Response Measurement1" class="Slide (strict)"() -> ("Value"=w683:u16)  [unwired: 2 in, 2 out]
                  }
                  frame 1 {
                    w685 = u16 0 items=["Absolute", "Relative"] ("Response Measurement")
                  }
                }
              }
              frame True {
                n287 = case shown="1" w689 {
                  tunnel: [w690 w691] -> w687
                  frame 0, Default {
                    w690 = u16 1 items=["Absolute", "Relative"] ("Response Measurement")
                  }
                  frame 1 {
                    w691 = u16 0 items=["Absolute", "Relative"] ("Response Measurement")
                  }
                }
              }
            }
            n288 = disable-structure shown="Disabled" {
              disable-tunnel: w676 -> [w679 _]
              frame Disabled {
                n289 = property on="Over-samples Res.(Hz)" class="DigNum (strict)"("Visible"=w679) -> ()  [unwired: 2 in, 2 out]
              }
              frame Enabled {
              }
            }
            n290 = property on="Reference Resistor(ohm)" class="DigNum (strict)"("Visible"=w652) -> ()  [unwired: 2 in, 2 out]
            n291 = property on="Amp Auto Mode" class="Slide (strict)"("Visible"=w652) -> ("Value"=w651:u16)  [unwired: 2 in, 2 out]
            n292 = Select(t=u8 0 ("Disabled"), s=w654, f=u8 2 ("Disabled")) -> (s? t:f=w656:u8)
            n293 = property on="Freq.Resolution(Hz)" class="DigNum (strict)"("Visible"=w671) -> ()  [unwired: 2 in, 2 out]
            n294 = property on="Auto-Correlation(Stimulus)" class="Bool (strict)"("Visible"=w665) -> ()  [unwired: 2 in, 2 out]
            n295 = property on="Auto-Correlation(Response)" class="Bool (strict)"("Visible"=w664) -> ()  [unwired: 2 in, 2 out]
            n296 = property on="Cross-Correlation" class="Bool (strict)"("Visible"=w663) -> ()  [unwired: 2 in, 2 out]
            n297 = Equal To 0?(x=w651) -> (x = 0?=w650:bool)
            n298 = Select(t=u8 2 ("Disabled"), s=w650, f=u8 0 ("Disabled")) -> (s? t:f=w647:u8)
            n299 = property on="Result Waveforms" class="Bool (strict)"("Visible"=w677) -> ()  [unwired: 2 in, 2 out]
            n300 = property on="Envelope?" class="Bool (strict)"("Visible"=w677) -> ()  [unwired: 2 in, 2 out]
            n301 = property on="Fmin(Hz)" class="DigNum (strict)"("Visible"=w677) -> ()  [unwired: 2 in, 2 out]
            n302 = property on="Fmax(Hz)" class="DigNum (strict)"("Visible"=w677) -> ()  [unwired: 2 in, 2 out]
            n303 = property on="Scaling" class="Ring (strict)"("Visible"=w655) -> ()  [unwired: 2 in, 2 out]
            n304 = property on="Response Measurement1" class="Slide (strict)"("Disabled"=w660) -> ()  [unwired: 2 in, 2 out]
            n305 = property on="Response Measurement1" class="Slide (strict)"("Value"=w659) -> ()  [unwired: 2 in, 2 out]
            n306 = property on="Reference Resistor(ohm)" class="DigNum (strict)"("DisabledEnum"=w647) -> ()  [unwired: 2 in, 2 out]
            n307 = property on="Fmax(Hz)" class="DigNum (strict)"("Disabled"=w656) -> ()  [unwired: 2 in, 2 out]
            n308 = property on="Fmin(Hz)" class="DigNum (strict)"("Disabled"=w656) -> ()  [unwired: 2 in, 2 out]
          }
          frame #1 {
            # "LooseParticle"
            # "Waveform"
            # "Electrical"
            # "Distortion"
            # "Frequency"
            n309 = local read "Loose Particle"() -> (w961:bool)
            n310 = property on="Apply Correction Out" class="Bool (strict)"("Visible"=w946) -> ()  [unwired: 2 in, 2 out]
            n311 = property on="Waveforms Out" class="Ring (strict)"("Visible"=w946) -> ()  [unwired: 2 in, 2 out]
            n312 = property on="Type Out" class="Str"("Visible"=w946) -> ()  [unwired: 2 in, 2 out]
            n313 = property on="Channel Out" class="Str"("Visible"=w946) -> ()  [unwired: 2 in, 2 out]
            n314 = property on="Stimulus" class="Bool (strict)"("Visible"=w946) -> ()  [unwired: 2 in, 2 out]
            n315 = case shown="False" w946 {
              tunnel: w961 -> [w1054 w1055]
              frame False {
                w1053 = FALSE ("Visible")
                n316 = property on="Loose Particle Waveform" class="Bool (strict)"("Visible"=w1053) -> ()  [unwired: 2 in, 2 out]
                n317 = property on="Attack Threshold(dB)" class="DigNum (strict)"("Visible"=w1054) -> ()  [unwired: 2 in, 2 out]
                n318 = property on="Min duration(s)" class="DigNum (strict)"("Visible"=w1053) -> ()  [unwired: 2 in, 2 out]
                n319 = property on="Hysteresis Up(dB)" class="DigNum (strict)"("Visible"=w1053) -> ()  [unwired: 2 in, 2 out]
                n320 = property on="Averaging Time(s)" class="DigNum (strict)"("Visible"=w1053) -> ()  [unwired: 2 in, 2 out]
                n321 = property on="Max duration(s)" class="DigNum (strict)"("Visible"=w1053) -> ()  [unwired: 2 in, 2 out]
              }
              frame True {
                n322 = property on="Min duration(s)" class="DigNum (strict)"("Visible"=w1055) -> ()  [unwired: 2 in, 2 out]
                n323 = property on="Hysteresis Up(dB)" class="DigNum (strict)"("Visible"=w1055) -> ()  [unwired: 2 in, 2 out]
                n324 = property on="Attack Threshold(dB)" class="DigNum (strict)"("Visible"=w1055) -> ()  [unwired: 2 in, 2 out]
                n325 = property on="Averaging Time(s)" class="DigNum (strict)"("Visible"=w1055) -> ()  [unwired: 2 in, 2 out]
                n326 = property on="Max duration(s)" class="DigNum (strict)"("Visible"=w1055) -> ()  [unwired: 2 in, 2 out]
                n327 = property on="Loose Particle Waveform" class="Bool (strict)"("Visible"=w1055) -> ()  [unwired: 2 in, 2 out]
              }
            }
            n328 = property on="Response" class="Bool (strict)"("Visible"=w946) -> ()  [unwired: 2 in, 2 out]
            n329 = property on="Apply Correction in" class="Bool (strict)"("Visible"=w946) -> ()  [unwired: 2 in, 2 out]
            n330 = property on="Waveforms In" class="Ring (strict)"("Visible"=w946) -> ()  [unwired: 2 in, 2 out]
            n331 = property on="Type in" class="Str"("Visible"=w946) -> ()  [unwired: 2 in, 2 out]
            n332 = property on="Channel in" class="Str"("Visible"=w946) -> ()  [unwired: 2 in, 2 out]
            n333 = case shown="True" w946 {
              tunnel: w959 -> [w981 w1021]
              tunnel: [_ w1020] -> w943
              tunnel: [_ w1019] -> w958
              tunnel: [w980 w1018] -> w947
              tunnel: [w969 w1017] -> w957
              tunnel: [w972 w1016] -> w956
              tunnel: [w971 w1015] -> w955
              tunnel: [w970 w1014] -> w954
              tunnel: [w974 w1013] -> w953
              tunnel: [w973 w1012] -> w952
              tunnel: [w979 w1011] -> w951
              tunnel: [w978 w1010] -> w950
              tunnel: [w977 w1009] -> w949
              tunnel: [w976 w1008] -> w948
              tunnel: [w975 w1007] -> w945
              frame False {
                n334 = case shown="2" w981 {
                  tunnel: [_ FALSE ("Visible") FALSE ("Visible")] -> w980
                  tunnel: [_ FALSE ("Visible") FALSE ("Visible")] -> w969
                  tunnel: [_ w991 w1005] -> w972
                  tunnel: [_ w990 w1003] -> w971
                  tunnel: [_ w989 w1003] -> w970
                  tunnel: [_ w988 w1003] -> w974
                  tunnel: [_ w987 w1003] -> w973
                  tunnel: [_ w986 w1003] -> w979
                  tunnel: [_ w985 w1005] -> w978
                  tunnel: [_ w984 w1003] -> w977
                  tunnel: [_ w983 w1003] -> w976
                  tunnel: [_ w982 w1003] -> w975
                  frame Default {
                  }
                  frame 2 {
                    n335 = local read "Type"() -> (w992:u16)
                    n336 = case shown="0, Default" w992 {
                      tunnel: [TRUE ("Visible") w999 w1001] -> w991
                      tunnel: [w995 w998 w1001] -> w990
                      tunnel: [w995 w999 w1002] -> w989
                      tunnel: [w995 w998 w1001] -> w988
                      tunnel: [w995 w999 w1002] -> w987
                      tunnel: [w995 w1000 w1001] -> w986
                      tunnel: [w996 w1000 w1001] -> w985
                      tunnel: [w995 w1000 w1001] -> w984
                      tunnel: [w996 w1000 w1001] -> w983
                      tunnel: [w995 w1000 w1001] -> w982
                      frame 0, Default {
                        w995 = FALSE ("Visible")
                        w996 = TRUE ("Visible")
                      }
                      frame 1 {
                        w998 = TRUE ("Visible")
                        w1000 = FALSE ("Visible")
                        w999 = FALSE ("Visible")
                      }
                      frame 2 {
                        w1002 = TRUE ("Visible")
                        w1001 = FALSE ("Visible")
                      }
                    }
                  }
                  frame 4 {
                    w1005 = TRUE ("Visible")
                    w1003 = FALSE ("Visible")
                  }
                }
              }
              frame True {
                n337 = case shown="5, 6" w1021 {
                  tunnel: [FALSE ("Visible") _ w1046 TRUE ("Visible") _] -> w1020
                  tunnel: [FALSE ("Visible") _ w1046 w1050 _] -> w1019
                  tunnel: [_ TRUE ("Visible") w1046 _ _] -> w1018
                  tunnel: [_ TRUE ("Visible") TRUE ("Visible") _ _] -> w1017
                  tunnel: [_ w1033 w1049 _ _] -> w1016
                  tunnel: [_ w1032 w1047 _ _] -> w1015
                  tunnel: [_ w1031 w1047 _ _] -> w1014
                  tunnel: [_ w1030 w1047 _ _] -> w1013
                  tunnel: [_ w1029 w1047 _ _] -> w1012
                  tunnel: [_ w1028 w1049 _ _] -> w1011
                  tunnel: [_ w1027 w1049 _ _] -> w1010
                  tunnel: [_ w1026 w1049 _ _] -> w1009
                  tunnel: [_ w1025 w1047 _ _] -> w1008
                  tunnel: [_ w1024 w1049 _ _] -> w1007
                  frame 1 {
                  }
                  frame 2 {
                    n338 = local read "Type"() -> (w1034:u16)
                    n339 = case shown="2" w1034 {
                      tunnel: [TRUE ("Visible") w1040 w1044] -> w1033
                      tunnel: [w1037 w1041 w1044] -> w1032
                      tunnel: [w1037 w1040 w1043] -> w1031
                      tunnel: [w1037 w1041 w1044] -> w1030
                      tunnel: [w1037 w1040 w1043] -> w1029
                      tunnel: [w1038 w1042 w1045] -> w1028
                      tunnel: [w1038 w1042 w1045] -> w1027
                      tunnel: [w1038 w1042 w1045] -> w1026
                      tunnel: [w1038 w1042 w1045] -> w1025
                      tunnel: [w1038 w1042 w1045] -> w1024
                      frame 0, Default {
                        w1038 = TRUE ("Visible")
                        w1037 = FALSE ("Visible")
                      }
                      frame 1 {
                        w1041 = TRUE ("Visible")
                        w1042 = FALSE ("Visible")
                        w1040 = FALSE ("Visible")
                      }
                      frame 2 {
                        w1044 = FALSE ("Visible")
                        w1043 = TRUE ("Visible")
                        w1045 = FALSE ("Visible")
                      }
                    }
                  }
                  frame 4 {
                    w1049 = TRUE ("Visible")
                    w1047 = FALSE ("Visible")
                    w1046 = FALSE ("Visible")
                  }
                  frame 5, 6 {
                    n340 = local read "Averaging1"() -> (w1051:u16)
                    n341 = Equal To 0?(x=w1051) -> (x = 0?=w1050:bool)
                  }
                  frame Default {
                  }
                }
              }
            }
            n342 = Equal?(x=w959, y=T10."Broadband RMS") -> (x = y?=w944:bool)
            n343 = property on="Mic Frame" class="Bool (strict)"("Visible"=w944) -> ()  [unwired: 2 in, 2 out]
            n344 = property on="Mic Current" class="Bool (strict)"("Visible"=w944) -> ()  [unwired: 2 in, 2 out]
            n345 = case shown="True" w944 {
              selector: w944 -> [w962 _]
              frame False {
                n346 = property on="Mic Resistor(ohm)" class="DigNum (strict)"("Visible"=w962) -> ()  [unwired: 2 in, 2 out]
                n347 = property on="Mic Auto Mode" class="Slide (strict)"("Visible"=w962) -> ()  [unwired: 2 in, 2 out]
              }
              frame True {
                n348 = property on="Mic Current" class="Bool (strict)"() -> ("Value"=w968:bool)  [unwired: 2 in, 2 out]
                n349 = property on="Mic Resistor(ohm)" class="DigNum (strict)"("Visible"=w968) -> ()  [unwired: 2 in, 2 out]
                n350 = property on="Mic Auto Mode" class="Slide (strict)"("Visible"=w968) -> ("Value"=w964:u16)  [unwired: 2 in, 2 out]
                n351 = Equal To 0?(x=w964) -> (x = 0?=w965:bool)
                n352 = Select(t=u8 2 ("Disabled"), s=w965, f=u8 0 ("Disabled")) -> (s? t:f=w963:u8)
                n353 = property on="Mic Resistor(ohm)" class="DigNum (strict)"("DisabledEnum"=w963) -> ()  [unwired: 2 in, 2 out]
              }
            }
            n354 = property on="Harmonics @ meas.frq" class="Bool (strict)"("Visible"=w951) -> ()  [unwired: 2 in, 2 out]
            n355 = property on="Total Distortion" class="Bool (strict)"("Visible"=w950) -> ()  [unwired: 2 in, 2 out]
            n356 = property on="THD(%)" class="Bool (strict)"("Visible"=w950) -> ()  [unwired: 2 in, 2 out]
            n357 = property on="Rub & Buzz(%)" class="Bool (strict)"("Visible"=w950) -> ()  [unwired: 2 in, 2 out]
            n358 = property on="THD Normalized(%)" class="Bool (strict)"("Visible"=w949) -> ()  [unwired: 2 in, 2 out]
            n359 = property on="THD + Noise (%)" class="Bool (strict)"("Visible"=w948) -> ()  [unwired: 2 in, 2 out]
            n360 = property on="Rub & Buzz Norm'd(%)" class="Bool (strict)"("Visible"=w945) -> ()  [unwired: 2 in, 2 out]
            n361 = property on="Harmonics" class="LstBox (strict)"("Visible"=w956) -> ()  [unwired: 2 in, 2 out]
            n362 = property on="Orders IM" class="LstBox (strict)"("Visible"=w955) -> ()  [unwired: 2 in, 2 out]
            n363 = property on="Orders Diff" class="LstBox (strict)"("Visible"=w954) -> ()  [unwired: 2 in, 2 out]
            n364 = property on="Method" class="Slide (strict)"("Visible"=w957) -> ()  [unwired: 2 in, 2 out]
            n365 = property on="Perceptual Rub & Buzz(phons)" class="Bool (strict)"("Visible"=w945) -> ()  [unwired: 2 in, 2 out]
            n366 = property on="Total IM" class="Bool (strict)"("Visible"=w953) -> ()  [unwired: 2 in, 2 out]
            n367 = property on="Total IMD(%)" class="Bool (strict)"("Visible"=w953) -> ()  [unwired: 2 in, 2 out]
            n368 = property on="Total IMD + Noise(%)" class="Bool (strict)"("Visible"=w953) -> ()  [unwired: 2 in, 2 out]
            n369 = property on="Type" class="Slide (strict)"("Visible"=w947) -> ()  [unwired: 2 in, 2 out]
            n370 = property on="Measurement Confidence" class="Bool (strict)"("Visible"=w947) -> ()  [unwired: 2 in, 2 out]
            n371 = property on="Standard Error" class="Bool (strict)"("Visible"=w947) -> ()  [unwired: 2 in, 2 out]
            n372 = property on="Confidence Limits" class="Bool (strict)"("Visible"=w947) -> ()  [unwired: 2 in, 2 out]
            n373 = property on="+/-" class="DigNum (strict)"("Visible"=w947) -> ()  [unwired: 2 in, 2 out]
            n374 = property on="Total Noise" class="Bool (strict)"("Visible"=w947) -> ()  [unwired: 2 in, 2 out]
            n375 = property on="Total Diff" class="Bool (strict)"("Visible"=w952) -> ()  [unwired: 2 in, 2 out]
            n376 = property on="Total DFD (%)" class="Bool (strict)"("Visible"=w952) -> ()  [unwired: 2 in, 2 out]
            n377 = property on="Total DFD + Noise(%)" class="Bool (strict)"("Visible"=w952) -> ()  [unwired: 2 in, 2 out]
            n378 = property on="Auto-Spectrum(Stimulus)*" class="Bool (strict)"("Visible"=w943) -> ()  [unwired: 2 in, 2 out]
            n379 = property on="Frequency Response" class="Bool (strict)"("Visible"=w943) -> ()  [unwired: 2 in, 2 out]
            n380 = property on="Coherent Power*" class="Bool (strict)"("Visible"=w958) -> ()  [unwired: 2 in, 2 out]
            n381 = property on="Non-Coherent Power*" class="Bool (strict)"("Visible"=w958) -> ()  [unwired: 2 in, 2 out]
            n382 = property on="Cross-Spectrum*" class="Bool (strict)"("Visible"=w958) -> ()  [unwired: 2 in, 2 out]
            n383 = property on="Coherence (%)" class="Bool (strict)"("Visible"=w958) -> ()  [unwired: 2 in, 2 out]
            n384 = property on="Non-Coherence (%)" class="Bool (strict)"("Visible"=w958) -> ()  [unwired: 2 in, 2 out]
            n385 = property on="Signal-Noise Ratio (dB)" class="Bool (strict)"("Visible"=w958) -> ()  [unwired: 2 in, 2 out]
            n386 = property on="Non-Coherenct Dustortion*" class="Bool (strict)"("Visible"=w958) -> ()  [unwired: 2 in, 2 out]
            n387 = property on="Averaging" class="Bool (strict)"("Visible"=w943) -> ()  [unwired: 2 in, 2 out]
            n388 = property on="Averaging1" class="Slide (strict)"("Visible"=w943) -> ()  [unwired: 2 in, 2 out]
            n389 = property on="Functions" class="Bool (strict)"("Visible"=w943) -> ()  [unwired: 2 in, 2 out]
            n390 = property on="Spectra" class="Bool (strict)"("Visible"=w943) -> ()  [unwired: 2 in, 2 out]
            n391 = property on="Spectral Scaling*" class="Ring (strict)"("Visible"=w943) -> ()  [unwired: 2 in, 2 out]
            n392 = property on="Auto-Spectrum(Response)*" class="Bool (strict)"("Visible"=w943) -> ()  [unwired: 2 in, 2 out]
          }
        }
      }
      event "CurveUpdate": Value Change {
        n393 = event-data() -> ("CtlRef"=w1074:refnum<vi>)  [unwired: 6 out]
        n394 = property class="Bool (strict)"(reference=w1074, "Value"=FALSE) -> ()  [unwired: 1 in, 2 out]
        n395 = local read "Analysis"() -> (w1060:T1)
        n396 = call "CRYFlatten Analysis.vi"("Analysis"=w1060) -> ("Analysis flattened"=w1067:string)  [unwired: 10 in]
        n397 = call "CRYGet Current TS Steps.vi"() -> ("SelectStepNumber in Tree"=w1070:i32, "Steps"=w1069:T4[])  [unwired: 1 in, 9 out]
        n398 = flat-sequence {
          tunnel: w1058 -> [w1079]
          tunnel: w1057 -> [w1076]
          tunnel: w1056 -> [w1075]
          frame #0 {
            n399 = property on="Changed Curve" class="Arr (strict)"() -> ("Value"=w1081:string[][])  [unwired: 2 in, 2 out]
            n400 = property on="Change Curve Name?" class="Bool (strict)"() -> ("Value"=w1083:bool)  [unwired: 2 in, 2 out]
            n401 = property on="Change Use Channel?" class="Bool (strict)"() -> ("Value"=w1078:bool)  [unwired: 2 in, 2 out]
            n402 = property on="Old Name" class="Arr (strict)"() -> ("Value"=w1080:string[])  [unwired: 2 in, 2 out]
            n403 = property on="Use Channel Name" class="Bool (strict)"() -> ("Value"=w1077:bool)  [unwired: 2 in, 2 out]
            n404 = call "CRYGet Changed Ana Curve Name.vi"("Old Name"=w1080, "Signal Tyep"=w1076, "Use Channel Name?"=w1077, "Current Name"=w1079, "Changed Name Table in"=w1081, "New Custom Type( Channel case)"=w1075, "Change State"=w1083, "Change Use Channel"=w1078) -> ("Changed Name Table  out"=→"Changed Curve":string[][])  [unwired: 7 in]
            n405 = property on="Old Name" class="Arr (strict)"("Value"=w1079) -> ()  [unwired: 2 in, 2 out]
          }
          frame #1 {
            n406 = property on="Change Curve Name?" class="Bool (strict)"("Value"=FALSE ("Change Curve Name?")) -> ()  [unwired: 2 in, 2 out]
            n407 = property on="Change Use Channel?" class="Bool (strict)"("Value"=FALSE ("Change Use Channel?")) -> ()  [unwired: 2 in, 2 out]
          }
        }
        n408 = Index Array(array=w1069, index=w1070) -> (element=w1071:T4)
        n409 = call "CRYReplace Analysis Curve Name.vi"("Setup in"=w1071, "Step Setup In"=w1067, "InsertSocket?"=FALSE, "Type In"="AddStep") -> ("New Custom Name( Channel case)"=w1058:string[], "Signal Type"=w1057:string, "Curve Info Array Out"=w1072:T14, "New Custom Type( Channel case)"=w1056:string[])  [unwired: 3 in, 1 out]
        n410 = for {
          tunnel: w1072 -> [w1089] mode=indexing
          tunnel: [w1088] -> w1059 mode=indexing
          tunnel: [w1087] -> w1065 mode=indexing
          tunnel: [w1086] -> w1064 mode=indexing
          n411 = Unbundle By Name(w1089) -> ("Custom Curve Names"=w1088:string, "Custom Curve IDs"=w1087:i32, "Default Curve Names"=w1086:string)
        }
        n412 = Bundle By Name(cluster=w1060, "Custom Curve Names"=w1059, "Custom Curve IDs"=w1065, "Default Curve Names"=w1064) -> (w1061:T1)
        n413 = Build Array(w1059) -> (w1063:string[][])
        n414 = local write "Analysis"(w1061) -> ()
        n415 = Transpose 2D Array(2D array=w1063) -> (transposed array=w1062:string[][])
        n416 = property on="Custom Curve Names" class="Tbl (strict)"("Value"=w1062) -> ()  [unwired: 2 in, 2 out]
      }
      event "Custom Curve Names": Value Change {
        n417 = event-data() -> ("NewVal"=w1090:string[][])  [unwired: 6 out]
        n418 = flat-sequence {
          tunnel: w1090 -> [w1095]
          frame #0 {
            n419 = Index Array(array=w1095, index (col)=0 ("disabled index (col)")) -> (element=w1093:string[])  [unwired: 1 in]
            n420 = local read "Analysis"() -> (w1096:T1)
            n421 = Bundle By Name(cluster=w1096, "Custom Curve Names"=w1093) -> (w1092:T1)
            n422 = property on="Change Curve Name?" class="Bool (strict)"("Value"=TRUE ("Change Curve Name?")) -> ()  [unwired: 2 in, 2 out]
            n423 = local write "Analysis"(w1092) -> ()
          }
          frame #1 {
            n424 = property on="CurveUpdate" class="Bool (strict)"("Val(Sgnl)"=TRUE ("Value (Signaling)")) -> ()  [unwired: 2 in, 2 out]
          }
        }
      }
      event "Cross-Correlation": Value Change {
        n425 = event-data() -> ("NewVal"=w1099:bool)  [unwired: 6 out]
        n426 = flat-sequence {
          tunnel: w1099 -> [w1101]
          frame #0 {
            n427 = local read "Analysis"() -> (w1102:T1)
            n428 = Bundle By Name(cluster=w1102, "Cross-Correlation"=w1101) -> (w1100:T1)
            n429 = local write "Analysis"(w1100) -> ()
          }
          frame #1 {
            n430 = property on="CurveUpdate" class="Bool (strict)"("Val(Sgnl)"=TRUE ("Value (Signaling)")) -> ()  [unwired: 2 in, 2 out]
          }
        }
        n431 = property on="Visible Update" class="Bool (strict)"("Val(Sgnl)"=TRUE ("Value (Signaling)")) -> ()  [unwired: 2 in, 2 out]
      }
      event "s": Value Change {
        n432 = event-data() -> ("NewVal"=w1108:dbl)  [unwired: 6 out]
        n433 = property on="Distance Unit" class="Ring (strict)"() -> ("Value"=w1111:u16)  [unwired: 2 in, 2 out]
        n434 = case shown="0, Default" w1111 {
          tunnel: w1108 -> [w1116 w1119]
          tunnel: [w1113 w1118] -> w1105
          tunnel: "distance" -> [w1112 w1117]
          frame 0, Default {
            n435 = Multiply(x=w1116, y=w1112) -> (x*y=w1114:dbl)
            n436 = Multiply(x=w1114, y=39.37) -> (x*y=w1113:dbl)
          }
          frame 1 {
            n437 = Multiply(x=w1119, y=w1117) -> (x*y=w1118:dbl)
          }
        }
        n438 = Multiply(x=w1108, y="Hardware In Fs") -> (x*y=w1110:dbl)
        n439 = property on="samples" class="DigNum (strict)"("Value"=w1110) -> ()  [unwired: 2 in, 2 out]
        n440 = local read "Analysis"() -> (w1109:T1)
        n441 = Bundle By Name(cluster=w1109, "delay"=w1108, "samples"=w1110, "distance"=w1105) -> (w1104:T1)
        n442 = property on="distance" class="DigNum (strict)"("Value"=w1105) -> ()  [unwired: 2 in, 2 out]
        n443 = local write "Analysis"(w1104) -> ()
      }
      event "Waveforms Out": Value Change {
        n444 = event-data() -> ("NewVal"=w1130:u16)  [unwired: 6 out]
        n445 = property on="Waveforms Out" class="Ring (strict)"() -> ("Strings []"=w1131:string[])  [unwired: 2 in, 2 out]
        n446 = Index Array(array=w1131, index=w1130) -> (element=w1128:string)
        n447 = call "CRYGet Curve Library Data.vi"("Type"=enum16{"Curves", "Values", "Results", "WFM"}."WFM", "Data Name"=w1128) -> ("Wave"=w1127:T13)  [unwired: 4 out]
        n448 = local read "Analysis"() -> (w1132:T1)
        n449 = Bundle By Name(cluster=w1132, "Waveform Out"=w1128) -> (w1120:T1)
        n450 = Unbundle By Name(w1127) -> ("Test Info"=w1125:string)
        n451 = local write "Analysis"(w1120) -> ()
        n452 = call "CRYUnflatten Test Infor.vi"("Falattend test infor"=w1125) -> ("unflattened test infor data"=w1126:T15)  [unwired: 9 out]
        n453 = Unbundle By Name(w1126) -> ("Stimulus Type"=w1122:string, "Signal Type"=w1121:string, "Sampling Rate"=→"Wave Out Fs":dbl, "Samples"=→"Wave Ou Sn":i32)
        n454 = local write "Type Out"(w1122) -> ()
        n455 = local write "Channel Out"(w1121) -> ()
      }
      event "Waveforms In": Value Change {
        n456 = event-data() -> ("NewVal"=w1153:u16)  [unwired: 6 out]
        n457 = property on="Waveforms In" class="Ring (strict)"() -> ("Strings []"=w1154:string[])  [unwired: 2 in, 2 out]
        n458 = Index Array(array=w1154, index=w1153) -> (element=w1150:string)
        n459 = call "CRYGet Curve Library Data.vi"("Type"=enum16{"Curves", "Values", "Results", "WFM"}."WFM", "Data Name"=w1150) -> ("Wave"=w1151:T13)  [unwired: 4 out]
        n460 = local read "Analysis"() -> (w1155:T1)
        n461 = Bundle By Name(cluster=w1155, "Waveform In"=w1150) -> (w1142:T1)
        n462 = Unbundle By Name(w1151) -> ("Test Info"=w1148:string)
        n463 = local write "Analysis"(w1142) -> ()
        n464 = call "CRYUnflatten Test Infor.vi"("Falattend test infor"=w1148) -> ("unflattened test infor data"=w1147:T15)  [unwired: 9 out]
        n465 = Unbundle By Name(w1147) -> ("Stimulus Type"=w1146:string, "Signal Type"=w1137:string, "Samples"=w1145:i32, "Sampling Rate"=w1143:dbl)
        n466 = Build Array(w1137) -> (w1136:string[])
        n467 = call "CRYUnflatten Calibration 2D.vi"("Flattened Calibration"=w1140) -> ("Calibration Step Out"=w1138:T16)  [unwired: 8 in, 2 out]
        n468 = call "CRYGet Channel From Signal Type.vi"("Calibration"=w1138, "Signal Type Name Array In"=w1136, "In/Out?"=TRUE) -> ("Channel Name Array Out"=w1135:string[])  [unwired: 7 in, 1 out]
        n469 = flat-sequence {
          tunnel: w1146 -> [w1158]
          tunnel: w1137 -> [w1157]
          tunnel: w1145 -> [w1160]
          tunnel: w1143 -> [w1159]
          tunnel: w1133 -> [w1156]
          frame #0 {
            n470 = local write "Channel in"(w1157) -> ()
            n471 = local write "Type in"(w1158) -> ()
            n472 = local write "Hardware In Fs"(w1156) -> ()
            "Wave In Sn" <- w1160
            "Wave In Fs" <- w1159
          }
          frame #1 {
            n473 = property on="Freq.Resolution(Hz)" class="DigNum (strict)"() -> ("Value"=w1162:dbl)  [unwired: 2 in, 2 out]
            n474 = property on="s" class="DigNum (strict)"() -> ("Value"=w1161:dbl)  [unwired: 2 in, 2 out]
            n475 = property on="s" class="DigNum (strict)"("Val(Sgnl)"=w1161) -> ()  [unwired: 2 in, 2 out]
            n476 = property on="Freq.Resolution(Hz)" class="DigNum (strict)"("Val(Sgnl)"=w1162) -> ()  [unwired: 2 in, 2 out]
          }
        }
        n477 = Index Array(array=w1135) -> (element=w1134:string)  [unwired: 1 in]
        n478 = call "CRYGet Info From Channel Name.vi"("Channel Name"=w1134, "Hardware In"=w1149) -> ("In_ChannelInfo"=w1144:T19)  [unwired: 9 out]
        n479 = Unbundle By Name(w1144) -> ("Sampling Rate (Hz)"=w1141:u32)
        n480 = To Double Precision Float(number=w1141) -> (double precision float=w1133:dbl)
      }
      event "Apply Correction Out": Value Change {
        n481 = event-data() -> ("NewVal"=w1164:bool)  [unwired: 6 out]
        n482 = local read "Analysis"() -> (w1165:T1)
        n483 = Bundle By Name(cluster=w1165, "Apply Correction Out"=w1164) -> (w1163:T1)
        n484 = local write "Analysis"(w1163) -> ()
      }
      event "Apply Correction in": Value Change {
        n485 = event-data() -> ("NewVal"=w1167:bool)  [unwired: 6 out]
        n486 = local read "Analysis"() -> (w1168:T1)
        n487 = Bundle By Name(cluster=w1168, "Apply Correction In"=w1167) -> (w1166:T1)
        n488 = local write "Analysis"(w1166) -> ()
      }
      event "Harmonics @ meas.frq": Value Change {
        n489 = event-data() -> ("NewVal"=w1169:bool)  [unwired: 6 out]
        n490 = flat-sequence {
          tunnel: w1169 -> [w1171]
          frame #0 {
            n491 = local read "Analysis"() -> (w1172:T1)
            n492 = Bundle By Name(cluster=w1172, "Harmonics @ meas.frq"=w1171) -> (w1170:T1)
            n493 = local write "Analysis"(w1170) -> ()
          }
          frame #1 {
            n494 = property on="CurveUpdate" class="Bool (strict)"("Val(Sgnl)"=TRUE ("Value (Signaling)")) -> ()  [unwired: 2 in, 2 out]
          }
        }
      }
      event "Distance Unit": Value Change {
        n495 = event-data() -> ("NewVal"=w1177:u16)  [unwired: 6 out]
        n496 = property on="distance" class="DigNum (strict)"() -> ("Value"=w1176:dbl)  [unwired: 2 in, 2 out]
        n497 = case shown="1" w1177 {
          tunnel: [w1180 w1183] -> w1175
          tunnel: w1176 -> [w1179 w1182]
          frame 0, Default {
            n498 = Multiply(x=w1179, y=39.37 ("distance")) -> (x*y=w1180:dbl)
          }
          frame 1 {
            n499 = Divide(x=w1182, y=39.37 ("distance")) -> (x/y=w1183:dbl)
          }
        }
        n500 = property on="distance" class="DigNum (strict)"("Value"=w1175) -> ()  [unwired: 2 in, 2 out]
        n501 = local read "Analysis"() -> (w1178:T1)
        n502 = Bundle By Name(cluster=w1178, "Distance Unit"=w1177, "distance"=w1175) -> (w1174:T1)
        n503 = local write "Analysis"(w1174) -> ()
      }
      event "samples": Value Change {
        n504 = event-data() -> ("NewVal"=w1189:dbl)  [unwired: 6 out]
        n505 = local read "Hardware In Fs"() -> (w1188:dbl)
        n506 = local read "distance"() -> (w1187:dbl)
        n507 = property on="Distance Unit" class="Ring (strict)"() -> ("Value"=w1192:u16)  [unwired: 2 in, 2 out]
        n508 = case shown="0, Default" w1192 {
          tunnel: w1189 -> [w1199 w1204]
          tunnel: [w1196 w1201] -> w1186
          tunnel: w1188 -> [w1195 w1202]
          tunnel: w1187 -> [w1193 w1200]
          frame 0, Default {
            n509 = Divide(x=w1199, y=w1195) -> (x/y=w1197:dbl)
            n510 = Multiply(x=w1197, y=w1193) -> (x*y=w1194:dbl)
            n511 = Multiply(x=w1194, y=39.37) -> (x*y=w1196:dbl)
          }
          frame 1 {
            n512 = Divide(x=w1204, y=w1202) -> (x/y=w1203:dbl)
            n513 = Multiply(x=w1203, y=w1200) -> (x*y=w1201:dbl)
          }
        }
        n514 = Divide(x=w1189, y=w1188) -> (x/y=w1190:dbl)
        n515 = property on="s" class="DigNum (strict)"("Value"=w1190) -> ()  [unwired: 2 in, 2 out]
        n516 = property on="distance" class="DigNum (strict)"("Value"=w1186) -> ()  [unwired: 2 in, 2 out]
        n517 = local read "Analysis"() -> (w1191:T1)
        n518 = Bundle By Name(cluster=w1191, "samples"=w1189, "delay"=w1190, "distance"=w1186) -> (w1185:T1)
        n519 = local write "Analysis"(w1185) -> ()
      }
      event "distance": Value Change {
        n520 = event-data() -> ("NewVal"=w1210:dbl)  [unwired: 6 out]
        n521 = local read "Hardware In Fs"() -> (w1209:dbl)
        n522 = property on="Distance Unit" class="Ring (strict)"() -> ("Value"=w1211:u16)  [unwired: 2 in, 2 out]
        n523 = local read "distance"() -> (w1208:dbl)
        n524 = case shown="0, Default" w1211 {
          tunnel: w1210 -> [w1215 w1224]
          tunnel: w1209 -> [w1221 w1226]
          tunnel: w1208 -> [w1214 w1223]
          tunnel: [w1218 w1225] -> w1207
          tunnel: [w1213 w1222] -> w1206
          frame 0, Default {
            w1216 = 39.37 ("y")
            n525 = Multiply(x=w1215, y=w1221) -> (x*y=w1220:dbl)
            n526 = Divide(x=w1220, y=w1214) -> (x/y=w1219:dbl)
            n527 = Divide(x=w1215, y=w1214) -> (x/y=w1217:dbl)
            n528 = Divide(x=w1219, y=w1216) -> (x/y=w1218:dbl)
            n529 = Divide(x=w1217, y=w1216) -> (x/y=w1213:dbl)
          }
          frame 1 {
            n530 = Multiply(x=w1224, y=w1226) -> (x*y=w1227:dbl)
            n531 = Divide(x=w1227, y=w1223) -> (x/y=w1225:dbl)
            n532 = Divide(x=w1224, y=w1223) -> (x/y=w1222:dbl)
          }
        }
        n533 = local read "Analysis"() -> (w1212:T1)
        n534 = Bundle By Name(cluster=w1212, "delay"=w1206, "distance"=w1210, "samples"=w1207) -> (w1205:T1)
        n535 = property on="samples" class="DigNum (strict)"("Value"=w1207) -> ()  [unwired: 2 in, 2 out]
        n536 = property on="s" class="DigNum (strict)"("Value"=w1206) -> ()  [unwired: 2 in, 2 out]
        n537 = local write "Analysis"(w1205) -> ()
      }
      event "Start Time(s)": Value Change {
        n538 = event-data() -> ("NewVal"=w1229:dbl)  [unwired: 6 out]
        n539 = local read "StopTime(s)"() -> (w1233:dbl)
        n540 = Subtract(x=w1233, y=w1229) -> (x-y=w1232:dbl)
        n541 = Reciprocal(x=w1232) -> (1/x=w1230:dbl)
        n542 = local write "Windowed Resolution(Hz)"(w1230) -> ()
        n543 = local read "Analysis"() -> (w1231:T1)
        n544 = Bundle By Name(cluster=w1231, "start ms"=w1229, "Win Resolution"=w1230) -> (w1228:T1)
        n545 = local write "Analysis"(w1228) -> ()
      }
      event "TSR Window Type": Value Change {
        n546 = event-data() -> ()  [unwired: 7 out]
        n547 = property on="TSR Window Type" class="Ring (strict)"() -> ("RingText.Text"=w1235:string)  [unwired: 2 in, 2 out]
        n548 = local read "Analysis"() -> (w1236:T1)
        n549 = Bundle By Name(cluster=w1236, "TSR Window Type"=w1235) -> (w1234:T1)
        n550 = local write "Analysis"(w1234) -> ()
      }
      event "Impedance": Value Change {
        n551 = event-data() -> ("NewVal"=w1237:bool)  [unwired: 6 out]
        n552 = case shown="True" w1237 {
          frame False {
          }
          frame True {
            n553 = property on="Mic Current" class="Bool (strict)"("Val(Sgnl)"=FALSE ("Value (Signaling)")) -> ()  [unwired: 2 in, 2 out]
          }
        }
        n554 = flat-sequence {
          tunnel: w1237 -> [w1243]
          frame #0 {
            n555 = local read "Analysis"() -> (w1242:T1)
            n556 = Bundle By Name(cluster=w1242, "Imp"=w1243, "ResponseMe"=u16 1) -> (w1241:T1)
            n557 = local write "Analysis"(w1241) -> ()
          }
          frame #1 {
            n558 = property on="CurveUpdate" class="Bool (strict)"("Val(Sgnl)"=TRUE ("Value (Signaling)")) -> ()  [unwired: 2 in, 2 out]
          }
        }
        n559 = property on="Visible Update" class="Bool (strict)"("Val(Sgnl)"=TRUE ("Value (Signaling)")) -> ()  [unwired: 2 in, 2 out]
      }
      event "StopTime(s)": Value Change {
        n560 = event-data() -> ("NewVal"=w1247:dbl)  [unwired: 6 out]
        n561 = local read "Start Time(s)"() -> (w1249:dbl)
        n562 = Subtract(x=w1247, y=w1249) -> (x-y=w1250:dbl)
        n563 = Reciprocal(x=w1250) -> (1/x=w1246:dbl)
        n564 = local write "Windowed Resolution(Hz)"(w1246) -> ()
        n565 = local read "Analysis"() -> (w1248:T1)
        n566 = Bundle By Name(cluster=w1248, "stop ms"=w1247, "Win Resolution"=w1246) -> (w1245:T1)
        n567 = local write "Analysis"(w1245) -> ()
      }
      event "Averaging1": Value Change {
        n568 = event-data() -> ("NewVal"=w1252:u16)  [unwired: 6 out]
        n569 = flat-sequence {
          tunnel: w1252 -> [w1255]
          frame #0 {
            n570 = local read "Analysis"() -> (w1254:T1)
            n571 = Bundle By Name(cluster=w1254, "Averaging"=w1255) -> (w1253:T1)
            n572 = local write "Analysis"(w1253) -> ()
          }
          frame #1 {
            n573 = property on="CurveUpdate" class="Bool (strict)"("Val(Sgnl)"=TRUE ("Value (Signaling)")) -> ()  [unwired: 2 in, 2 out]
          }
        }
        n574 = property on="Visible Update" class="Bool (strict)"("Val(Sgnl)"=TRUE ("Value (Signaling)")) -> ()  [unwired: 2 in, 2 out]
      }
      event "Curve Step Resolution": Value Change {
        n575 = event-data() -> ("NewVal"=w1259:u16)  [unwired: 6 out]
        n576 = Greater Or Equal?(x=w1259, y=u16 5) -> (x >= y?=w1257:bool)
        n577 = local read "Analysis"() -> (w1261:T1)
        n578 = Bundle By Name(cluster=w1261, "Curve Resolution"=w1259) -> (w1260:T1)
        n579 = property on="Curve Resolution Hz" class="DigNum (strict)"("Visible"=w1257) -> ()  [unwired: 2 in, 2 out]
        n580 = local write "Analysis"(w1260) -> ()
      }
      event "Curve Resolution Hz": Value Change {
        n581 = event-data() -> ("NewVal"=w1264:dbl)  [unwired: 6 out]
        n582 = local read "Analysis"() -> (w1263:T1)
        n583 = Bundle By Name(cluster=w1263, "Curve Resolution Hz"=w1264) -> (w1262:T1)
        n584 = local write "Analysis"(w1262) -> ()
      }
      event "Loose Particle": Value Change {
        n585 = event-data() -> ("NewVal"=w1265:bool)  [unwired: 6 out]
        n586 = flat-sequence {
          tunnel: w1265 -> [w1269]
          frame #0 {
            n587 = local read "Analysis"() -> (w1268:T1)
            n588 = Bundle By Name(cluster=w1268, "Loose Particle"=w1269) -> (w1267:T1)
            n589 = local write "Analysis"(w1267) -> ()
          }
          frame #1 {
            n590 = property on="CurveUpdate" class="Bool (strict)"("Val(Sgnl)"=TRUE ("Value (Signaling)")) -> ()  [unwired: 2 in, 2 out]
          }
        }
        n591 = property on="Visible Update" class="Bool (strict)"("Val(Sgnl)"=TRUE ("Value (Signaling)")) -> ()  [unwired: 2 in, 2 out]
      }
      event "Loose Particle Waveform": Value Change {
        n592 = event-data() -> ("NewVal"=w1271:bool)  [unwired: 6 out]
        n593 = flat-sequence {
          tunnel: w1271 -> [w1275]
          frame #0 {
            n594 = local read "Analysis"() -> (w1274:T1)
            n595 = Bundle By Name(cluster=w1274, "Loose Particle waveform"=w1275) -> (w1273:T1)
            n596 = local write "Analysis"(w1273) -> ()
          }
          frame #1 {
            n597 = property on="CurveUpdate" class="Bool (strict)"("Val(Sgnl)"=TRUE ("Value (Signaling)")) -> ()  [unwired: 2 in, 2 out]
          }
        }
        n598 = property on="Visible Update" class="Bool (strict)"("Val(Sgnl)"=TRUE ("Value (Signaling)")) -> ()  [unwired: 2 in, 2 out]
      }
      event "Use default": Value Change {
        n599 = event-data() -> ("NewVal"=w1277:bool)  [unwired: 6 out]
        n600 = flat-sequence {
          tunnel: w1277 -> [w1281]
          frame #0 {
            n601 = local read "Analysis"() -> (w1280:T1)
            n602 = Bundle By Name(cluster=w1280, "Use default"=w1281) -> (w1279:T1)
            n603 = local write "Analysis"(w1279) -> ()
            n604 = property on="Change Curve Name?" class="Bool (strict)"("Value"=TRUE ("Change Curve Name?")) -> ()  [unwired: 2 in, 2 out]
          }
          frame #1 {
            n605 = property on="CurveUpdate" class="Bool (strict)"("Val(Sgnl)"=TRUE ("Value (Signaling)")) -> ()  [unwired: 2 in, 2 out]
          }
        }
        n606 = case shown="True" w1277 {
          frame False {
            n607 = property on="Custom Curve Names" class="Tbl (strict)"("Disabled"=u8 0) -> ()  [unwired: 2 in, 2 out]
          }
          frame True {
            n608 = property on="Custom Curve Names" class="Tbl (strict)"("Disabled"=u8 2) -> ()  [unwired: 2 in, 2 out]
          }
        }
      }
      event "Maxis": Value Change {
        n609 = event-data() -> ("NewVal"=w1299:u16)  [unwired: 6 out]
        n610 = property on="LR" class="Ring (strict)"() -> ("RingText.Text"=w1286:string)  [unwired: 2 in, 2 out]
        n611 = for {
          tunnel: w1297 -> [w1316] mode=indexing
          tunnel: w1286 -> [w1319]
          tunnel: [w1316] -> w1296
          stop <- w1317 stop-if-true
          n612 = Unbundle By Name(w1316) -> ("Name"=w1318:string)
          n613 = Equal?(x=w1319, y=w1318) -> (x = y?=w1317:bool)
        }
        n614 = Unbundle By Name(w1296) -> ("Curve"=w1295:cluster{"x":dbl, "y":dbl, "z":dbl}[], "X unit"=w1292:string, "Y unit"=w1291:string, "Z unit"=w1293:string)
        n615 = Index Array(array=w1295) -> (element=w1294:cluster{"x":dbl, "y":dbl, "z":dbl})  [unwired: 1 in]
        n616 = case shown="2" w1299 {
          tunnel: w1294 -> [w1322 w1325 w1328]
          tunnel: [w1320 w1324 w1327] -> w1287
          tunnel: [w1321 w1323 w1326] -> w1290
          tunnel: w1293 -> [_ _ w1326]
          tunnel: w1292 -> [w1321 _ _]
          tunnel: w1291 -> [_ w1323 _]
          frame 0, Default {
            n617 = Unbundle By Name(w1322) -> ("x"=w1320:dbl)
          }
          frame 1 {
            n618 = Unbundle By Name(w1325) -> ("y"=w1324:dbl)
          }
          frame 2 {
            n619 = Unbundle By Name(w1328) -> ("z"=w1327:dbl)
          }
        }
        n620 = local read "Applied Units"() -> (w1289:u16)
        n621 = local read "Distance Unit"() -> (w1288:u16)
        n622 = local write "Hz"(w1287) -> ()
        n623 = case shown="0, Default" w1289 {
          tunnel: w1288 -> [_ _ w1304 w1310]
          tunnel: w1287 -> [w1300 w1301 w1303 w1309]
          frame 0, Default {
            n624 = property on="s" class="DigNum (strict)"("Val(Sgnl)"=w1300) -> ()  [unwired: 2 in, 2 out]
          }
          frame 1 {
            n625 = property on="samples" class="DigNum (strict)"("Val(Sgnl)"=w1301) -> ()  [unwired: 2 in, 2 out]
          }
          frame 2 {
            n626 = case shown="1" w1304 {
              tunnel: [w1305 w1306] -> w1302
              tunnel: w1303 -> [w1305 w1308]
              frame 0, Default {
              }
              frame 1 {
                n627 = Divide(x=w1308, y=39.37 ("distance")) -> (x/y=w1306:dbl)
              }
            }
            n628 = property on="distance" class="DigNum (strict)"("Val(Sgnl)"=w1302) -> ()  [unwired: 2 in, 2 out]
          }
          frame 3 {
            n629 = case shown="0, Default" w1310 {
              tunnel: [w1312 w1315] -> w1311
              tunnel: w1309 -> [w1314 w1315]
              frame 0, Default {
                n630 = Multiply(x=w1314, y=39.37 ("distance")) -> (x*y=w1312:dbl)
              }
              frame 1 {
              }
            }
            n631 = property on="distance" class="DigNum (strict)"("Val(Sgnl)"=w1311) -> ()  [unwired: 2 in, 2 out]
          }
        }
        n632 = property on="Hz" class="DigNum (strict)"("Caption.Text"=w1290) -> ()  [unwired: 2 in, 2 out]
        n633 = local read "Analysis"() -> (w1298:T1)
        n634 = Bundle By Name(cluster=w1298, "M List Vaiues"=w1299, "Hz"=w1287) -> (w1285:T1)
        n635 = local write "Analysis"(w1285) -> ()
      }
      event "Advanced View": Value Change {
        n636 = event-data() -> ("NewVal"=w1331:bool)  [unwired: 6 out]
        n637 = local read "Analysis"() -> (w1332:T1)
        n638 = Bundle By Name(cluster=w1332, "Advanced View"=w1331) -> (w1329:T1)
        n639 = local write "Analysis"(w1329) -> ()
        n640 = property on="Visible Update" class="Bool (strict)"("Val(Sgnl)"=TRUE ("Value (Signaling)")) -> ()  [unwired: 2 in, 2 out]
      }
      event "Type": Value Change {
        n641 = event-data() -> ("NewVal"=w1334:u16)  [unwired: 6 out]
        n642 = flat-sequence {
          tunnel: w1334 -> [w1336]
          frame #0 {
            n643 = local read "Analysis"() -> (w1337:T1)
            n644 = Bundle By Name(cluster=w1337, "Type"=w1336) -> (w1335:T1)
            n645 = local write "Analysis"(w1335) -> ()
          }
          frame #1 {
            n646 = property on="CurveUpdate" class="Bool (strict)"("Val(Sgnl)"=TRUE ("Value (Signaling)")) -> ()  [unwired: 2 in, 2 out]
          }
        }
        n647 = property on="Visible Update" class="Bool (strict)"("Val(Sgnl)"=TRUE ("Value (Signaling)")) -> ()  [unwired: 2 in, 2 out]
      }
      event "Total Distortion": Value Change {
        n648 = event-data() -> ("NewVal"=w1339:bool)  [unwired: 6 out]
        n649 = flat-sequence {
          tunnel: w1339 -> [w1341]
          frame #0 {
            n650 = local read "Analysis"() -> (w1342:T1)
            n651 = Bundle By Name(cluster=w1342, "Total Distortion"=w1341) -> (w1340:T1)
            n652 = local write "Analysis"(w1340) -> ()
          }
          frame #1 {
            n653 = property on="CurveUpdate" class="Bool (strict)"("Val(Sgnl)"=TRUE ("Value (Signaling)")) -> ()  [unwired: 2 in, 2 out]
          }
        }
      }
      event "THD(%)": Value Change {
        n654 = event-data() -> ("NewVal"=w1344:bool)  [unwired: 6 out]
        n655 = flat-sequence {
          tunnel: w1344 -> [w1346]
          frame #0 {
            n656 = local read "Analysis"() -> (w1347:T1)
            n657 = Bundle By Name(cluster=w1347, "THD(%)"=w1346) -> (w1345:T1)
            n658 = local write "Analysis"(w1345) -> ()
          }
          frame #1 {
            n659 = property on="CurveUpdate" class="Bool (strict)"("Val(Sgnl)"=TRUE ("Value (Signaling)")) -> ()  [unwired: 2 in, 2 out]
          }
        }
      }
      event "THD Normalized(%)": Value Change {
        n660 = event-data() -> ("NewVal"=w1349:bool)  [unwired: 6 out]
        n661 = flat-sequence {
          tunnel: w1349 -> [w1351]
          frame #0 {
            n662 = local read "Analysis"() -> (w1352:T1)
            n663 = Bundle By Name(cluster=w1352, "THD Normalized(%)"=w1351) -> (w1350:T1)
            n664 = local write "Analysis"(w1350) -> ()
          }
          frame #1 {
            n665 = property on="CurveUpdate" class="Bool (strict)"("Val(Sgnl)"=TRUE ("Value (Signaling)")) -> ()  [unwired: 2 in, 2 out]
          }
        }
      }
      event "Total Noise": Value Change {
        n666 = event-data() -> ("NewVal"=w1354:bool)  [unwired: 6 out]
        n667 = flat-sequence {
          tunnel: w1354 -> [w1356]
          frame #0 {
            n668 = local read "Analysis"() -> (w1357:T1)
            n669 = Bundle By Name(cluster=w1357, "Total Noise"=w1356) -> (w1355:T1)
            n670 = local write "Analysis"(w1355) -> ()
          }
          frame #1 {
            n671 = property on="CurveUpdate" class="Bool (strict)"("Val(Sgnl)"=TRUE ("Value (Signaling)")) -> ()  [unwired: 2 in, 2 out]
          }
        }
      }
      event "Response Measurement1": Value Change {
        n672 = event-data() -> ("NewVal"=w1360:u16)  [unwired: 6 out]
        n673 = local read "Analysis"() -> (w1361:T1)
        n674 = Bundle By Name(cluster=w1361, "ResponseMe"=w1360) -> (w1359:T1)
        n675 = local write "Analysis"(w1359) -> ()
      }
      event "Rub & Buzz Norm'd(%)": Value Change {
        n676 = event-data() -> ("NewVal"=w1362:bool)  [unwired: 6 out]
        n677 = flat-sequence {
          tunnel: w1362 -> [w1364]
          frame #0 {
            n678 = local read "Analysis"() -> (w1365:T1)
            n679 = Bundle By Name(cluster=w1365, "Rub&Buzz Norm'd(%)"=w1364) -> (w1363:T1)
            n680 = local write "Analysis"(w1363) -> ()
          }
          frame #1 {
            n681 = property on="CurveUpdate" class="Bool (strict)"("Val(Sgnl)"=TRUE ("Value (Signaling)")) -> ()  [unwired: 2 in, 2 out]
          }
        }
      }
      event "Perceptual Rub & Buzz(phons)": Value Change {
        n682 = event-data() -> ("NewVal"=w1367:bool)  [unwired: 6 out]
        n683 = flat-sequence {
          tunnel: w1367 -> [w1369]
          frame #0 {
            n684 = local read "Analysis"() -> (w1370:T1)
            n685 = Bundle By Name(cluster=w1370, "Perceptual Rub&Buzz"=w1369) -> (w1368:T1)
            n686 = local write "Analysis"(w1368) -> ()
          }
          frame #1 {
            n687 = property on="CurveUpdate" class="Bool (strict)"("Val(Sgnl)"=TRUE ("Value (Signaling)")) -> ()  [unwired: 2 in, 2 out]
          }
        }
      }
      event "Rub & Buzz(%)": Value Change {
        n688 = event-data() -> ("NewVal"=w1372:bool)  [unwired: 6 out]
        n689 = flat-sequence {
          tunnel: w1372 -> [w1374]
          frame #0 {
            n690 = local read "Analysis"() -> (w1375:T1)
            n691 = Bundle By Name(cluster=w1375, "Rub&Buzz"=w1374) -> (w1373:T1)
            n692 = local write "Analysis"(w1373) -> ()
          }
          frame #1 {
            n693 = property on="CurveUpdate" class="Bool (strict)"("Val(Sgnl)"=TRUE ("Value (Signaling)")) -> ()  [unwired: 2 in, 2 out]
          }
        }
      }
      event "Method": Value Change {
        n694 = event-data() -> ("NewVal"=w1378:u16)  [unwired: 6 out]
        n695 = local read "Analysis"() -> (w1379:T1)
        n696 = Bundle By Name(cluster=w1379, "Method"=w1378) -> (w1377:T1)
        n697 = local write "Analysis"(w1377) -> ()
      }
      event "Delay Method": Value Change {
        n698 = event-data() -> ("NewVal"=w1384:u16)  [unwired: 6 out]
        n699 = Equal To 0?(x=w1384) -> (x = 0?=w1383:bool)
        n700 = property on="Delay Treat" class="Slide (strict)"("Val(Sgnl)"=w1384) -> ()  [unwired: 2 in, 2 out]
        n701 = Select(t=T11."Enabled" ("Disabled"), s=w1383, f=T11."Disabled and Grayed Out" ("Disabled")) -> (s? t:f=w1380:T11)
        n702 = flat-sequence {
          tunnel: w1384 -> [w1387]
          frame #0 {
            n703 = local read "Analysis"() -> (w1386:T1)
            n704 = Bundle By Name(cluster=w1386, "Delay Method"=w1387) -> (w1385:T1)
            n705 = local write "Analysis"(w1385) -> ()
          }
          frame #1 {
            n706 = property on="CurveUpdate" class="Bool (strict)"("Val(Sgnl)"=TRUE ("Value (Signaling)")) -> ()  [unwired: 2 in, 2 out]
          }
        }
        n707 = property on="Polarity" class="Bool (strict)"("DisabledEnum"=w1380) -> ()  [unwired: 2 in, 2 out]
      }
      event "Polarity": Value Change {
        n708 = event-data() -> ("NewVal"=w1389:bool)  [unwired: 6 out]
        n709 = flat-sequence {
          tunnel: w1389 -> [w1392]
          frame #0 {
            n710 = local read "Analysis"() -> (w1391:T1)
            n711 = Bundle By Name(cluster=w1391, "Polarity"=w1392) -> (w1390:T1)
            n712 = local write "Analysis"(w1390) -> ()
          }
          frame #1 {
            n713 = property on="CurveUpdate" class="Bool (strict)"("Val(Sgnl)"=TRUE ("Value (Signaling)")) -> ()  [unwired: 2 in, 2 out]
          }
        }
      }
      event "Delay Treat": Value Change {
        n714 = event-data() -> ("NewVal"=w1394:u16)  [unwired: 6 out]
        n715 = case shown="0, Default" w1394 {
          frame 0, Default {
            w1423 = FALSE
            w1424 = u8 2 ("Disabled")
            n716 = local read "Analysis"() -> (w1396:T1)
            n717 = Unbundle By Name(w1396) -> ("use custom unit"=w1417:bool, "Custom Curve Names"=w1416:string[], "Custom Curve IDs"=w1415:i32[], "Default Curve Names"=w1414:string[], "Use default"=w1413:bool, "Distance Unit"=w1422:u16)
            n718 = property on="s" class="DigNum (strict)"("Disabled"=w1424) -> ()  [unwired: 2 in, 2 out]
            n719 = property on="samples" class="DigNum (strict)"("Disabled"=w1424) -> ()  [unwired: 2 in, 2 out]
            n720 = property on="distance" class="DigNum (strict)"("Disabled"=w1424) -> ()  [unwired: 2 in, 2 out]
            n721 = property on="Maxis" class="Slide (strict)"("Visible"=w1423) -> ()  [unwired: 2 in, 2 out]
            n722 = property on="LR" class="Ring (strict)"("Visible"=w1423) -> ()  [unwired: 2 in, 2 out]
            n723 = property on="Hz" class="DigNum (strict)"("Visible"=w1423) -> ()  [unwired: 2 in, 2 out]
            n724 = property on="Applied Units" class="Ring (strict)"("Visible"=w1423) -> ()  [unwired: 2 in, 2 out]
            n725 = property on="CurveLibValues" class="Bool (strict)"("Visible"=w1423) -> ()  [unwired: 2 in, 2 out]
            n726 = Bundle(FALSE, "Check Option"="", "use custom unit"=w1417, "Custom Curve Names"=w1416, "Custom Curve IDs"=w1415, "Default Curve Names"=w1414, "Use default"=w1413) -> (w1421:T20)  [unwired: 1 in]
            n727 = call "CRYGet Auto Delay Curve array.vi"("Additive Info"=w1421, "Distance Unit"=w1422) -> ("Curve Info Array Out"=w1420:T21)  [unwired: 7 in, 2 out]
            n728 = Index Array(array=w1420) -> (element=w1397:T22)  [unwired: 1 in]
            n729 = Unbundle By Name(w1396) -> ("Use Channel Name"=w1401:bool, "Waveform In"=w1400:string)
            n730 = Not Equal?(x=w1400, y="") -> (x != y?=w1402:bool)
            n731 = And(x=w1401, y=w1402) -> (x .and. y?=w1399:bool)
            n732 = call "CRYGet Curve Library Data.vi"("Type"=enum16{"Curves", "Values", "Results", "WFM"}."WFM", "Data Name"=w1400) -> ("Wave"=w1406:T13)  [unwired: 4 out]
            n733 = Unbundle By Name(w1406) -> ("Test Info"=w1405:string)  [unwired: 1 out]
            n734 = call "CRYUnflatten Test Infor.vi"("Falattend test infor"=w1405) -> ("unflattened test infor data"=w1404:T15)  [unwired: 9 out]
            n735 = Unbundle By Name(w1404) -> ("Signal Type"=w1398:string)
            n736 = case shown="False" w1399 {
              tunnel: w1397 -> [w1426 w1432]
              tunnel: [w1425 w1430] -> w1395
              tunnel: w1398 -> [_ w1431]
              frame False {
                n737 = Unbundle By Name(w1426) -> ("Custom Curve Name"=w1425:string)
              }
              frame True {
                n738 = Unbundle By Name(w1432) -> ("Custom Curve Name"=w1427:string)
                n739 = Concatenate Strings(w1427, " [" ("RecordDelay"), w1431, "]" ("string")) -> (w1430:string)
              }
            }
            n740 = call "CRYGet Curve Library Data.vi"("Type"=enum16{"Curves", "Values", "Results", "WFM"}."Values", "Data Name"=w1395) -> ("Value"=w1411:T6)  [unwired: 4 out]
            n741 = Unbundle By Name(w1411) -> ("Curve"=w1410:cluster{"x":dbl, "y":dbl, "z":dbl}[])
            n742 = Index Array(array=w1410) -> (element=w1409:cluster{"x":dbl, "y":dbl, "z":dbl})  [unwired: 1 in]
            n743 = Unbundle By Name(w1409) -> ("x"=w1408:dbl)
            n744 = property on="s" class="DigNum (strict)"("Val(Sgnl)"=w1408) -> ()  [unwired: 2 in, 2 out]
          }
          frame 1 {
            w1433 = FALSE
            w1434 = u8 0 ("Disabled")
            n745 = property on="s" class="DigNum (strict)"("Disabled"=w1434) -> ()  [unwired: 2 in, 2 out]
            n746 = property on="samples" class="DigNum (strict)"("Disabled"=w1434) -> ()  [unwired: 2 in, 2 out]
            n747 = property on="distance" class="DigNum (strict)"("Disabled"=w1434) -> ()  [unwired: 2 in, 2 out]
            n748 = property on="CurveLibValues" class="Bool (strict)"("Visible"=w1433) -> ()  [unwired: 2 in, 2 out]
            n749 = property on="Maxis" class="Slide (strict)"("Visible"=w1433) -> ()  [unwired: 2 in, 2 out]
            n750 = property on="LR" class="Ring (strict)"("Visible"=w1433) -> ()  [unwired: 2 in, 2 out]
            n751 = property on="Hz" class="DigNum (strict)"("Visible"=w1433) -> ()  [unwired: 2 in, 2 out]
            n752 = property on="Applied Units" class="Ring (strict)"("Visible"=w1433) -> ()  [unwired: 2 in, 2 out]
          }
          frame 2 {
            w1437 = T11."Disabled and Grayed Out" ("Disabled")
            w1435 = TRUE
            n753 = property on="s" class="DigNum (strict)"("Disabled"=w1437) -> ()  [unwired: 2 in, 2 out]
            n754 = property on="samples" class="DigNum (strict)"("Disabled"=w1437) -> ()  [unwired: 2 in, 2 out]
            n755 = property on="distance" class="DigNum (strict)"("Disabled"=w1437) -> ()  [unwired: 2 in, 2 out]
            n756 = property on="Maxis" class="Slide (strict)"("Visible"=w1435) -> ()  [unwired: 2 in, 2 out]
            n757 = property on="LR" class="Ring (strict)"("Visible"=w1435) -> ()  [unwired: 2 in, 2 out]
            n758 = property on="Hz" class="DigNum (strict)"("Visible"=w1435) -> ()  [unwired: 2 in, 2 out]
            n759 = property on="Applied Units" class="Ring (strict)"("Visible"=w1435) -> ()  [unwired: 2 in, 2 out]
            n760 = property on="CurveLibValues" class="Bool (strict)"("Visible"=w1435) -> ()  [unwired: 2 in, 2 out]
            n761 = local read "Maxis"() -> (w1436:u16)
            n762 = property on="Maxis" class="Slide (strict)"("Val(Sgnl)"=w1436) -> ()  [unwired: 2 in, 2 out]
          }
        }
      }
      event "LR": Value Change {
        n763 = event-data() -> ()  [unwired: 7 out]
        n764 = property on="LR" class="Ring (strict)"() -> ("RingText.Text"=w1439:string)  [unwired: 2 in, 2 out]
        n765 = property on="Maxis" class="Slide (strict)"() -> ("Value"=w1440:u16)  [unwired: 2 in, 2 out]
        n766 = property on="Maxis" class="Slide (strict)"("Val(Sgnl)"=w1440) -> ()  [unwired: 2 in, 2 out]
        n767 = local read "Analysis"() -> (w1441:T1)
        n768 = Bundle By Name(cluster=w1441, "unLabel"=w1439) -> (w1438:T1)
        n769 = local write "Analysis"(w1438) -> ()
      }
      event "Main Tab": Value Change {
        n770 = event-data() -> ("NewVal"=w1443:T3)  [unwired: 6 out]
        n771 = local read "Analysis"() -> (w1444:T1)
        n772 = Bundle By Name(cluster=w1444, "Tab"=w1443) -> (w1442:T1)
        n773 = local write "Analysis"(w1442) -> ()
      }
      event "Applied Units": Value Change {
        n774 = event-data() -> ("NewVal"=w1448:u16)  [unwired: 6 out]
        n775 = local read "Distance Unit"() -> (w1446:u16)
        n776 = local read "Hz"() -> (w1447:dbl)
        n777 = case shown="0, Default" w1448 {
          tunnel: w1447 -> [w1450 w1451 w1453 w1460]
          tunnel: w1446 -> [_ _ w1454 w1461]
          frame 0, Default {
            n778 = property on="s" class="DigNum (strict)"("Val(Sgnl)"=w1450) -> ()  [unwired: 2 in, 2 out]
          }
          frame 1 {
            n779 = property on="samples" class="DigNum (strict)"("Val(Sgnl)"=w1451) -> ()  [unwired: 2 in, 2 out]
          }
          frame 2 {
            n780 = case shown="1" w1454 {
              tunnel: [w1455 w1458] -> w1452
              tunnel: w1453 -> [w1455 w1457]
              frame 0, Default {
              }
              frame 1 {
                n781 = Divide(x=w1457, y=39.37) -> (x/y=w1458:dbl)
              }
            }
            n782 = property on="distance" class="DigNum (strict)"("Val(Sgnl)"=w1452) -> ()  [unwired: 2 in, 2 out]
          }
          frame 3 {
            n783 = case shown="0, Default" w1461 {
              tunnel: [w1463 w1465] -> w1459
              tunnel: w1460 -> [w1464 w1465]
              frame 0, Default {
                n784 = Multiply(x=w1464, y=39.37) -> (x*y=w1463:dbl)
              }
              frame 1 {
              }
            }
            n785 = property on="distance" class="DigNum (strict)"("Val(Sgnl)"=w1459) -> ()  [unwired: 2 in, 2 out]
          }
        }
        n786 = local read "Analysis"() -> (w1449:T1)
        n787 = Bundle By Name(cluster=w1449, "Appliied Unit"=w1448) -> (w1445:T1)
        n788 = local write "Analysis"(w1445) -> ()
      }
      event "Default Overlap": Value Change {
        n789 = event-data() -> ("NewVal"=w1470:bool)  [unwired: 6 out]
        n790 = case shown="False" w1470 {
          tunnel: [u8 0 ("Disabled") u8 2 ("Disabled")] -> w1467
          frame False {
          }
          frame True {
          }
        }
        n791 = property on="Overlap(%)" class="DigNum (strict)"("Disabled"=w1467) -> ()  [unwired: 2 in, 2 out]
        n792 = local read "Analysis"() -> (w1469:T1)
        n793 = Bundle By Name(cluster=w1469, "Default Overlap"=w1470) -> (w1466:T1)
        n794 = property on="Weighting" class="Ring (strict)"() -> ("Value"=w1468:u16)  [unwired: 2 in, 2 out]
        n795 = local write "Analysis"(w1466) -> ()
        n796 = property on="Weighting" class="Ring (strict)"("Val(Sgnl)"=w1468) -> ()  [unwired: 2 in, 2 out]
      }
      event "Envelope?": Value Change {
        n797 = event-data() -> ("NewVal"=w1473:bool)  [unwired: 6 out]
        n798 = case shown="True" w1473 {
          frame False {
            n799 = property on="Fmin(Hz)" class="DigNum (strict)"("Disabled"=u8 2) -> ()  [unwired: 2 in, 2 out]
            n800 = property on="Fmax(Hz)" class="DigNum (strict)"("Disabled"=u8 2) -> ()  [unwired: 2 in, 2 out]
          }
          frame True {
            n801 = property on="Fmin(Hz)" class="DigNum (strict)"("Disabled"=u8 0) -> ()  [unwired: 2 in, 2 out]
            n802 = property on="Fmax(Hz)" class="DigNum (strict)"("Disabled"=u8 0) -> ()  [unwired: 2 in, 2 out]
          }
        }
        n803 = property on="Visible Update" class="Bool (strict)"("Val(Sgnl)"=TRUE ("Value (Signaling)")) -> ()  [unwired: 2 in, 2 out]
        n804 = flat-sequence {
          tunnel: w1473 -> [w1477]
          frame #0 {
            n805 = local read "Analysis"() -> (w1476:T1)
            n806 = Bundle By Name(cluster=w1476, "Envelope"=w1477) -> (w1475:T1)
            n807 = local write "Analysis"(w1475) -> ()
          }
          frame #1 {
            n808 = property on="CurveUpdate" class="Bool (strict)"("Val(Sgnl)"=TRUE ("Value (Signaling)")) -> ()  [unwired: 2 in, 2 out]
          }
        }
      }
      event "Auto-Correlation(Stimulus)": Value Change {
        n809 = event-data() -> ("NewVal"=w1484:bool)  [unwired: 6 out]
        n810 = flat-sequence {
          tunnel: w1484 -> [w1487]
          frame #0 {
            n811 = local read "Analysis"() -> (w1486:T1)
            n812 = Bundle By Name(cluster=w1486, "Auto-Correlation(Stimulus)"=w1487) -> (w1485:T1)
            n813 = local write "Analysis"(w1485) -> ()
          }
          frame #1 {
            n814 = property on="CurveUpdate" class="Bool (strict)"("Val(Sgnl)"=TRUE ("Value (Signaling)")) -> ()  [unwired: 2 in, 2 out]
          }
        }
        n815 = property on="Visible Update" class="Bool (strict)"("Val(Sgnl)"=TRUE ("Value (Signaling)")) -> ()  [unwired: 2 in, 2 out]
      }
      event "Auto-Correlation(Response)": Value Change {
        n816 = event-data() -> ("NewVal"=w1490:bool)  [unwired: 6 out]
        n817 = flat-sequence {
          tunnel: w1490 -> [w1493]
          frame #0 {
            n818 = local read "Analysis"() -> (w1492:T1)
            n819 = Bundle By Name(cluster=w1492, "Auto-Correlation(Response)"=w1493) -> (w1491:T1)
            n820 = local write "Analysis"(w1491) -> ()
          }
          frame #1 {
            n821 = property on="CurveUpdate" class="Bool (strict)"("Val(Sgnl)"=TRUE ("Value (Signaling)")) -> ()  [unwired: 2 in, 2 out]
          }
        }
        n822 = property on="Visible Update" class="Bool (strict)"("Val(Sgnl)"=TRUE ("Value (Signaling)")) -> ()  [unwired: 2 in, 2 out]
      }
      event "Deconvolved Response": Value Change {
        n823 = event-data() -> ("NewVal"=w1496:bool)  [unwired: 6 out]
        n824 = property on="Visible Update" class="Bool (strict)"("Val(Sgnl)"=TRUE ("Value (Signaling)")) -> ()  [unwired: 2 in, 2 out]
        n825 = flat-sequence {
          tunnel: w1496 -> [w1499]
          frame #0 {
            n826 = local read "Analysis"() -> (w1498:T1)
            n827 = Bundle By Name(cluster=w1498, "Deconvolved Response"=w1499) -> (w1497:T1)
            n828 = local write "Analysis"(w1497) -> ()
          }
          frame #1 {
            n829 = property on="CurveUpdate" class="Bool (strict)"("Val(Sgnl)"=TRUE ("Value (Signaling)")) -> ()  [unwired: 2 in, 2 out]
          }
        }
      }
      event "impulse resp?": Value Change {
        n830 = event-data() -> ("NewVal"=w1502:bool)  [unwired: 6 out]
        n831 = flat-sequence {
          tunnel: w1502 -> [w1505]
          frame #0 {
            n832 = local read "Analysis"() -> (w1504:T1)
            n833 = Bundle By Name(cluster=w1504, "impulse"=w1505) -> (w1503:T1)
            n834 = local write "Analysis"(w1503) -> ()
          }
          frame #1 {
            n835 = property on="CurveUpdate" class="Bool (strict)"("Val(Sgnl)"=TRUE ("Value (Signaling)")) -> ()  [unwired: 2 in, 2 out]
          }
        }
        n836 = property on="Visible Update" class="Bool (strict)"("Val(Sgnl)"=TRUE ("Value (Signaling)")) -> ()  [unwired: 2 in, 2 out]
      }
      event "Mic Current": Value Change {
        n837 = event-data() -> ("NewVal"=w1507:bool)  [unwired: 6 out]
        n838 = flat-sequence {
          tunnel: w1507 -> [w1510]
          frame #0 {
            n839 = local read "Analysis"() -> (w1512:T1)
            n840 = Bundle By Name(cluster=w1512, "Mic Current"=w1510) -> (w1511:T1)
            n841 = local write "Analysis"(w1511) -> ()
          }
          frame #1 {
            n842 = property on="CurveUpdate" class="Bool (strict)"("Val(Sgnl)"=TRUE ("Value (Signaling)")) -> ()  [unwired: 2 in, 2 out]
          }
        }
        n843 = case shown="True" w1507 {
          frame False {
          }
          frame True {
            n844 = property on="Impedance" class="Bool (strict)"("Val(Sgnl)"=FALSE ("Impedance")) -> ()  [unwired: 2 in, 2 out]
          }
        }
        n845 = property on="Visible Update" class="Bool (strict)"("Val(Sgnl)"=TRUE ("Value (Signaling)")) -> ()  [unwired: 2 in, 2 out]
      }
      event "Harmonics": Value Change {
        n846 = event-data() -> ("NewVal"=w1515:i32)  [unwired: 6 out]
        n847 = local read "har checkoffs"() -> (w1517:bool[])
        n848 = Greater Or Equal To 0?(x=w1515) -> (x >= 0?=w1516:bool)
        n849 = case shown="True" w1516 {
          tunnel: w1517 -> [_ w1528]
          tunnel: w1515 -> [_ w1527]
          tunnel: [bool[] [] ("har checkoffs") w1526] -> w1514
          frame False {
          }
          frame True {
            n850 = stacked-sequence {
              tunnel: w1528 -> [w1533 _]
              tunnel: w1527 -> [w1531 _]
              tunnel: [w1529 _] -> w1526
              frame #0 {
                n851 = Index Array(array=w1533, index=w1531) -> (element=w1532:bool)
                n852 = Not(x=w1532) -> (.not. x?=w1534:bool)
                n853 = Replace Array Subset(array=w1533, new element=w1534, index=w1531) -> (w1529:bool[])
                n854 = for {
                  tunnel: w1529 -> [w1538] mode=indexing
                  tunnel: [w1537] -> w1530 mode=indexing
                  n855 = Select(t=1, s=w1538, f=0) -> (s? t:f=w1537:i32)
                }
                n856 = local write "har checkoffs"(w1529) -> ()
                n857 = property on="Harmonics" class="LstBox (strict)"("Item Symbols"=w1530) -> ()  [unwired: 2 in, 2 out]
              }
              frame #1 {
                n858 = local write "Harmonics"(-1 ("Harmonics")) -> ()
              }
            }
          }
        }
        n859 = flat-sequence {
          tunnel: w1514 -> [w1521]
          frame #0 {
            n860 = property on="Harmonics" class="LstBox (strict)"() -> ("Item Names"=w1523:string[])  [unwired: 2 in, 2 out]
            n861 = call "CRYHarmonics list to array.vi"("Checkoffs"=w1521, "Harmonic list items"=w1523) -> ("List items checked"=w1522:string[], "Harmonics array out"=w1519:dbl[])  [unwired: 8 out]
            n862 = local read "Analysis"() -> (w1520:T1)
            n863 = Bundle By Name(cluster=w1520, "Harmonics"=w1519, "har list items"=w1522) -> (w1518:T1)
            n864 = local write "Harmonics array out"(w1519) -> ()
            n865 = local write "Analysis"(w1518) -> ()
          }
          frame #1 {
            n866 = property on="CurveUpdate" class="Bool (strict)"("Val(Sgnl)"=TRUE ("Value (Signaling)")) -> ()  [unwired: 2 in, 2 out]
          }
        }
      }
      event "Orders IM": Value Change {
        n867 = event-data() -> ("NewVal"=w1543:i32)  [unwired: 6 out]
        n868 = local read "IM checkoffs"() -> (w1540:bool[])
        n869 = Greater Or Equal To 0?(x=w1543) -> (x >= 0?=w1542:bool)
        n870 = case shown="True" w1542 {
          tunnel: w1540 -> [_ w1554]
          tunnel: w1543 -> [_ w1553]
          tunnel: [bool[] [] ("har checkoffs") w1552] -> w1541
          frame False {
          }
          frame True {
            n871 = stacked-sequence {
              tunnel: w1554 -> [w1559 _]
              tunnel: w1553 -> [w1557 _]
              tunnel: [w1555 _] -> w1552
              frame #0 {
                n872 = Index Array(array=w1559, index=w1557) -> (element=w1558:bool)
                n873 = Not(x=w1558) -> (.not. x?=w1560:bool)
                n874 = Replace Array Subset(array=w1559, new element=w1560, index=w1557) -> (w1555:bool[])
                n875 = for {
                  tunnel: w1555 -> [w1564] mode=indexing
                  tunnel: [w1563] -> w1556 mode=indexing
                  n876 = Select(t=1, s=w1564, f=0) -> (s? t:f=w1563:i32)
                }
                n877 = local write "IM checkoffs"(w1555) -> ()
                n878 = property on="Orders IM" class="LstBox (strict)"("Item Symbols"=w1556) -> ()  [unwired: 2 in, 2 out]
              }
              frame #1 {
                n879 = local write "Orders IM"(-1 ("Harmonics")) -> ()
              }
            }
          }
        }
        n880 = flat-sequence {
          tunnel: w1541 -> [w1548]
          frame #0 {
            n881 = property on="Orders IM" class="LstBox (strict)"() -> ("Item Names"=w1546:string[])  [unwired: 2 in, 2 out]
            n882 = call "CRYHarmonics list to array.vi"("Checkoffs"=w1548, "Harmonic list items"=w1546) -> ("List items checked"=w1549:string[], "Harmonics array out"=w1545:dbl[])  [unwired: 8 out]
            n883 = local read "Analysis"() -> (w1547:T1)
            n884 = Bundle By Name(cluster=w1547, "Intermod"=w1545, "IM list items"=w1549) -> (w1544:T1)
            n885 = local write "IM array out"(w1545) -> ()
            n886 = local write "Analysis"(w1544) -> ()
          }
          frame #1 {
            n887 = property on="CurveUpdate" class="Bool (strict)"("Val(Sgnl)"=TRUE ("Value (Signaling)")) -> ()  [unwired: 2 in, 2 out]
          }
        }
      }
      event "Orders Diff": Value Change {
        n888 = event-data() -> ("NewVal"=w1567:i32)  [unwired: 6 out]
        n889 = local read "Diff checkoffs"() -> (w1566:bool[])
        n890 = Greater Or Equal To 0?(x=w1567) -> (x >= 0?=w1569:bool)
        n891 = case shown="True" w1569 {
          tunnel: w1566 -> [_ w1580]
          tunnel: w1567 -> [_ w1579]
          tunnel: [bool[] [] ("har checkoffs") w1578] -> w1568
          frame False {
          }
          frame True {
            n892 = stacked-sequence {
              tunnel: w1580 -> [w1585 _]
              tunnel: w1579 -> [w1583 _]
              tunnel: [w1581 _] -> w1578
              frame #0 {
                n893 = Index Array(array=w1585, index=w1583) -> (element=w1584:bool)
                n894 = Not(x=w1584) -> (.not. x?=w1586:bool)
                n895 = Replace Array Subset(array=w1585, new element=w1586, index=w1583) -> (w1581:bool[])
                n896 = for {
                  tunnel: w1581 -> [w1590] mode=indexing
                  tunnel: [w1589] -> w1582 mode=indexing
                  n897 = Select(t=1, s=w1590, f=0) -> (s? t:f=w1589:i32)
                }
                n898 = local write "Diff checkoffs"(w1581) -> ()
                n899 = property on="Orders Diff" class="LstBox (strict)"("Item Symbols"=w1582) -> ()  [unwired: 2 in, 2 out]
              }
              frame #1 {
                n900 = local write "Orders Diff"(-1 ("Harmonics")) -> ()
              }
            }
          }
        }
        n901 = flat-sequence {
          tunnel: w1568 -> [w1574]
          frame #0 {
            n902 = property on="Orders Diff" class="LstBox (strict)"() -> ("Item Names"=w1572:string[])  [unwired: 2 in, 2 out]
            n903 = call "CRYHarmonics list to array.vi"("Checkoffs"=w1574, "Harmonic list items"=w1572) -> ("List items checked"=w1575:string[], "Harmonics array out"=w1571:dbl[])  [unwired: 8 out]
            n904 = local read "Analysis"() -> (w1573:T1)
            n905 = Bundle By Name(cluster=w1573, "Diff"=w1571, "Diff list items"=w1575) -> (w1570:T1)
            n906 = local write "Diff array out"(w1571) -> ()
            n907 = local write "Analysis"(w1570) -> ()
          }
          frame #1 {
            n908 = property on="CurveUpdate" class="Bool (strict)"("Val(Sgnl)"=TRUE ("Value (Signaling)")) -> ()  [unwired: 2 in, 2 out]
          }
        }
      }
      event "THD + Noise (%)": Value Change {
        n909 = event-data() -> ("NewVal"=w1592:bool)  [unwired: 6 out]
        n910 = flat-sequence {
          tunnel: w1592 -> [w1594]
          frame #0 {
            n911 = local read "Analysis"() -> (w1595:T1)
            n912 = Bundle By Name(cluster=w1595, "THD+Noise(%)"=w1594) -> (w1593:T1)
            n913 = local write "Analysis"(w1593) -> ()
          }
          frame #1 {
            n914 = property on="CurveUpdate" class="Bool (strict)"("Val(Sgnl)"=TRUE ("Value (Signaling)")) -> ()  [unwired: 2 in, 2 out]
          }
        }
      }
      event "+/-": Value Change {
        n915 = event-data() -> ("NewVal"=w1598:dbl)  [unwired: 6 out]
        n916 = local read "Analysis"() -> (w1599:T1)
        n917 = Bundle By Name(cluster=w1599, "Std Err"=w1598) -> (w1597:T1)
        n918 = local write "Analysis"(w1597) -> ()
      }
      event "Standard Error": Value Change {
        n919 = event-data() -> ("NewVal"=w1600:bool)  [unwired: 6 out]
        n920 = flat-sequence {
          tunnel: w1600 -> [w1602]
          frame #0 {
            n921 = local read "Analysis"() -> (w1603:T1)
            n922 = Bundle By Name(cluster=w1603, "Standard Error"=w1602) -> (w1601:T1)
            n923 = local write "Analysis"(w1601) -> ()
          }
          frame #1 {
            n924 = property on="CurveUpdate" class="Bool (strict)"("Val(Sgnl)"=TRUE ("Value (Signaling)")) -> ()  [unwired: 2 in, 2 out]
          }
        }
      }
      event "Confidence Limits": Value Change {
        n925 = event-data() -> ("NewVal"=w1605:bool)  [unwired: 6 out]
        n926 = flat-sequence {
          tunnel: w1605 -> [w1607]
          frame #0 {
            n927 = local read "Analysis"() -> (w1608:T1)
            n928 = Bundle By Name(cluster=w1608, "Confidence Limits"=w1607) -> (w1606:T1)
            n929 = local write "Analysis"(w1606) -> ()
          }
          frame #1 {
            n930 = property on="CurveUpdate" class="Bool (strict)"("Val(Sgnl)"=TRUE ("Value (Signaling)")) -> ()  [unwired: 2 in, 2 out]
          }
        }
      }
      event "Over-samples Res.(Hz)": Value Change {
        n931 = event-data() -> ("NewVal"=w1613:dbl)  [unwired: 6 out]
        n932 = Less Than 0?(x=w1613) -> (x < 0?=w1614:bool)
        n933 = Select(t=0.0, s=w1614, f=w1613) -> (s? t:f=w1611:dbl)
        n934 = property on="Over-samples Res.(Hz)" class="DigNum (strict)"("Value"=w1611) -> ()  [unwired: 2 in, 2 out]
        n935 = local read "Analysis"() -> (w1615:T1)
        n936 = Bundle By Name(cluster=w1615, "Over-samples Res."=w1611) -> (w1610:T1)
        n937 = local write "Analysis"(w1610) -> ()
      }
      event "Reference Resistor(ohm)": Value Change {
        n938 = event-data() -> ("NewVal"=w1618:dbl)  [unwired: 6 out]
        n939 = Less?(x=w1618, y=0.0) -> (x < y?=w1620:bool)
        n940 = Select(t=0.0, s=w1620, f=w1618) -> (s? t:f=w1616:dbl)
        n941 = local read "Analysis"() -> (w1622:T1)
        n942 = Bundle By Name(cluster=w1622, "Imp Ref resistor"=w1616) -> (w1617:T1)
        n943 = local write "Analysis"(w1617) -> ()
      }
      event "Mic Resistor(ohm)": Value Change {
        n944 = event-data() -> ("NewVal"=w1625:dbl)  [unwired: 6 out]
        n945 = Less?(x=w1625, y=0.0) -> (x < y?=w1627:bool)
        n946 = Select(t=0.0, s=w1627, f=w1625) -> (s? t:f=w1623:dbl)
        n947 = local read "Analysis"() -> (w1629:T1)
        n948 = Bundle By Name(cluster=w1629, "Mic Ref resistor"=w1623) -> (w1624:T1)
        n949 = local write "Analysis"(w1624) -> ()
      }
      event "Amp Auto Mode": Value Change {
        n950 = event-data() -> ("NewVal"=w1636:u16)  [unwired: 6 out]
        n951 = Equal To 0?(x=w1636) -> (x = 0?=w1635:bool)
        n952 = local read "Reference Resistor(ohm)"() -> (w1634:dbl)
        n953 = global read "CRYHardware Global.vi" "Impedance 1"() -> (w1631:i32)
        n954 = Index Array(array=i32[] [1, 33, 33, 150, 600, 750], index=w1631) -> (element=w1630:i32)
        n955 = Select(t=w1630, s=w1635, f=w1634) -> (s? t:f=w1633:dbl)
        n956 = local write "Reference Resistor(ohm)"(w1633) -> ()
        n957 = flat-sequence {
          tunnel: w1636 -> [w1638]
          tunnel: w1633 -> [w1637]
          frame #0 {
            n958 = local read "Analysis"() -> (w1640:T1)
            n959 = Bundle By Name(cluster=w1640, "Imp Auto Mode"=w1638, "Imp Ref resistor"=w1637) -> (w1639:T1)
            n960 = local write "Analysis"(w1639) -> ()
          }
          frame #1 {
            n961 = property on="Visible Update" class="Bool (strict)"("Val(Sgnl)"=TRUE ("Value (Signaling)")) -> ()  [unwired: 2 in, 2 out]
          }
        }
      }
      event "Mic Auto Mode": Value Change {
        n962 = event-data() -> ("NewVal"=w1646:u16)  [unwired: 6 out]
        n963 = Equal To 0?(x=w1646) -> (x = 0?=w1645:bool)
        n964 = local read "Mic Resistor(ohm)"() -> (w1643:dbl)
        n965 = global read "CRYHardware Global.vi" "Mic Resister"() -> (w1644:dbl)
        n966 = Select(t=w1644, s=w1645, f=w1643) -> (s? t:f=w1642:dbl)
        n967 = local write "Mic Resistor(ohm)"(w1642) -> ()
        n968 = flat-sequence {
          tunnel: w1646 -> [w1648]
          tunnel: w1642 -> [w1647]
          frame #0 {
            n969 = local read "Analysis"() -> (w1650:T1)
            n970 = Bundle By Name(cluster=w1650, "Mic Auto Mode"=w1648, "Mic Ref resistor"=w1647) -> (w1649:T1)
            n971 = local write "Analysis"(w1649) -> ()
          }
          frame #1 {
            n972 = property on="Visible Update" class="Bool (strict)"("Val(Sgnl)"=TRUE ("Value (Signaling)")) -> ()  [unwired: 2 in, 2 out]
          }
        }
      }
      event "Total IM": Value Change {
        n973 = event-data() -> ("NewVal"=w1652:bool)  [unwired: 6 out]
        n974 = flat-sequence {
          tunnel: w1652 -> [w1654]
          frame #0 {
            n975 = local read "Analysis"() -> (w1655:T1)
            n976 = Bundle By Name(cluster=w1655, "Total IM"=w1654) -> (w1653:T1)
            n977 = local write "Analysis"(w1653) -> ()
          }
          frame #1 {
            n978 = property on="CurveUpdate" class="Bool (strict)"("Val(Sgnl)"=TRUE ("Value (Signaling)")) -> ()  [unwired: 2 in, 2 out]
          }
        }
      }
      event "Use Channel Name": Value Change {
        n979 = event-data() -> ("NewVal"=w1657:bool)  [unwired: 6 out]
        n980 = flat-sequence {
          tunnel: w1657 -> [w1661]
          frame #0 {
            n981 = local read "Analysis"() -> (w1660:T1)
            n982 = Bundle By Name(cluster=w1660, "Use Channel Name"=w1661) -> (w1659:T1)
            n983 = property on="Change Use Channel?" class="Bool (strict)"("Value"=TRUE ("Change Use Channel?")) -> ()  [unwired: 2 in, 2 out]
            n984 = local write "Analysis"(w1659) -> ()
          }
          frame #1 {
            n985 = property on="CurveUpdate" class="Bool (strict)"("Val(Sgnl)"=TRUE ("Value (Signaling)")) -> ()  [unwired: 2 in, 2 out]
          }
        }
      }
      event "Total IMD(%)": Value Change {
        n986 = event-data() -> ("NewVal"=w1663:bool)  [unwired: 6 out]
        n987 = flat-sequence {
          tunnel: w1663 -> [w1665]
          frame #0 {
            n988 = local read "Analysis"() -> (w1666:T1)
            n989 = Bundle By Name(cluster=w1666, "Total IMD(%)"=w1665) -> (w1664:T1)
            n990 = local write "Analysis"(w1664) -> ()
          }
          frame #1 {
            n991 = property on="CurveUpdate" class="Bool (strict)"("Val(Sgnl)"=TRUE ("Value (Signaling)")) -> ()  [unwired: 2 in, 2 out]
          }
        }
      }
      event "Total DFD (%)": Value Change {
        n992 = event-data() -> ("NewVal"=w1668:bool)  [unwired: 6 out]
        n993 = flat-sequence {
          tunnel: w1668 -> [w1670]
          frame #0 {
            n994 = local read "Analysis"() -> (w1671:T1)
            n995 = Bundle By Name(cluster=w1671, "Total DFD(%)"=w1670) -> (w1669:T1)
            n996 = local write "Analysis"(w1669) -> ()
          }
          frame #1 {
            n997 = property on="CurveUpdate" class="Bool (strict)"("Val(Sgnl)"=TRUE ("Value (Signaling)")) -> ()  [unwired: 2 in, 2 out]
          }
        }
      }
      event "Total Diff": Value Change {
        n998 = event-data() -> ("NewVal"=w1673:bool)  [unwired: 6 out]
        n999 = flat-sequence {
          tunnel: w1673 -> [w1675]
          frame #0 {
            n1000 = local read "Analysis"() -> (w1676:T1)
            n1001 = Bundle By Name(cluster=w1676, "Total Diff"=w1675) -> (w1674:T1)
            n1002 = local write "Analysis"(w1674) -> ()
          }
          frame #1 {
            n1003 = property on="CurveUpdate" class="Bool (strict)"("Val(Sgnl)"=TRUE ("Value (Signaling)")) -> ()  [unwired: 2 in, 2 out]
          }
        }
      }
      event "Total DFD + Noise(%)": Value Change {
        n1004 = event-data() -> ("NewVal"=w1678:bool)  [unwired: 6 out]
        n1005 = flat-sequence {
          tunnel: w1678 -> [w1680]
          frame #0 {
            n1006 = local read "Analysis"() -> (w1681:T1)
            n1007 = Bundle By Name(cluster=w1681, "Total DFD+Noise(%)"=w1680) -> (w1679:T1)
            n1008 = local write "Analysis"(w1679) -> ()
          }
          frame #1 {
            n1009 = property on="CurveUpdate" class="Bool (strict)"("Val(Sgnl)"=TRUE ("Value (Signaling)")) -> ()  [unwired: 2 in, 2 out]
          }
        }
      }
      event "Total IMD + Noise(%)": Value Change {
        n1010 = event-data() -> ("NewVal"=w1683:bool)  [unwired: 6 out]
        n1011 = flat-sequence {
          tunnel: w1683 -> [w1685]
          frame #0 {
            n1012 = local read "Analysis"() -> (w1686:T1)
            n1013 = Bundle By Name(cluster=w1686, "Total IMD + Noise(%)"=w1685) -> (w1684:T1)
            n1014 = local write "Analysis"(w1684) -> ()
          }
          frame #1 {
            n1015 = property on="CurveUpdate" class="Bool (strict)"("Val(Sgnl)"=TRUE ("Value (Signaling)")) -> ()  [unwired: 2 in, 2 out]
          }
        }
      }
      event "Weighting": Value Change {
        n1016 = event-data() -> ("NewVal"=w1690:u16)  [unwired: 6 out]
        n1017 = local read "Algorithm"() -> (w1695:u16)
        n1018 = property on="Default Overlap" class="Bool (strict)"() -> ("Value"=w1700:bool)  [unwired: 2 in, 2 out]
        n1019 = Equal?(x=w1695, y=T10."Multitone") -> (x = y?=w1693:bool)
        n1020 = Equal?(x=w1695, y=T10."Transfer Function") -> (x = y?=w1692:bool)
        n1021 = Equal?(x=w1695, y=T10."Spectrum") -> (x = y?=w1699:bool)
        n1022 = Compound Arithmetic op=OR(w1699, w1693, w1692) -> (w1694:bool)
        n1023 = And(x=w1694, y=w1700) -> (x .and. y?=w1698:bool)
        n1024 = case shown="True" w1698 {
          tunnel: w1690 -> [_ w1710]
          tunnel: [w1703 w1709] -> w1689
          frame False {
            n1025 = property on="Overlap(%)" class="DigNum (strict)"() -> ("Value"=w1703:dbl)  [unwired: 2 in, 2 out]
          }
          frame True {
            n1026 = case shown="8" w1710 {
              tunnel: [0.0 ("Overlap(%)") 75.0 ("Overlap(%)") 85.0 ("Overlap(%)") 90.0 ("Overlap(%)") 90.0 ("Overlap(%)")] -> w1709
              frame 0, Default {
              }
              frame 1 {
              }
              frame 7 {
              }
              frame 8 {
              }
              frame 6 {
              }
            }
            n1027 = property on="Overlap(%)" class="DigNum (strict)"("Value"=w1709) -> ()  [unwired: 2 in, 2 out]
            n1028 = local read "Wave In Fs"() -> (w1708:dbl)
            n1029 = local read "Wave In Sn"() -> (w1706:i32)
            n1030 = property on="Freq.Resolution(Hz)" class="DigNum (strict)"() -> ("Value"=w1707:dbl)  [unwired: 2 in, 2 out]
            n1031 = call "CRYGet Frequency Resolution Param.vi"("Overlap(%)"=w1709, "Fs"=w1708, "Freq Resolution(Hz)"=w1707, "Samples"=w1706) -> ("No. of FFT"=w1704:i32, "Record Length(s)"=w1705:dbl)  [unwired: 4 in, 2 out]
            n1032 = property on="Record Length (s)" class="DigNum (strict)"("Value"=w1705) -> ()  [unwired: 2 in, 2 out]
            n1033 = property on="No.of FFTs" class="DigNum (strict)"("Value"=w1704) -> ()  [unwired: 2 in, 2 out]
          }
        }
        n1034 = property on="Weighting" class="Ring (strict)"() -> ("RingText.Text"=w1691:string)  [unwired: 2 in, 2 out]
        n1035 = local read "Analysis"() -> (w1702:T1)
        n1036 = Bundle By Name(cluster=w1702, "Weigting"=w1691, "Overlap"=w1689) -> (w1688:T1)
        n1037 = local write "Analysis"(w1688) -> ()
      }
      event "Freq.Resolution(Hz)": Value Change {
        n1038 = event-data() -> ("NewVal"=w1719:dbl)  [unwired: 6 out]
        n1039 = local read "Analysis"() -> (w1723:T1)
        n1040 = Bundle By Name(cluster=w1723, "Freq.Resolution"=w1719) -> (w1716:T1)
        n1041 = local read "Wave In Sn"() -> (w1718:i32)
        n1042 = local read "Wave In Fs"() -> (w1717:dbl)
        n1043 = property on="Overlap(%)" class="DigNum (strict)"() -> ("Value"=w1722:dbl)  [unwired: 2 in, 2 out]
        n1044 = local write "Analysis"(w1716) -> ()
        n1045 = call "CRYGet Frequency Resolution Param.vi"("Overlap(%)"=w1722, "Fs"=w1717, "Freq Resolution(Hz)"=w1719, "Samples"=w1718) -> ("No. of FFT"=w1721:i32, "Record Length(s)"=w1720:dbl)  [unwired: 4 in, 2 out]
        n1046 = property on="No.of FFTs" class="DigNum (strict)"("Value"=w1721) -> ()  [unwired: 2 in, 2 out]
        n1047 = property on="Record Length (s)" class="DigNum (strict)"("Value"=w1720) -> ()  [unwired: 2 in, 2 out]
      }
      event "Overlap(%)": Value Change {
        n1048 = event-data() -> ("NewVal"=w1725:dbl)  [unwired: 6 out]
        n1049 = local read "Wave In Sn"() -> (w1728:i32)
        n1050 = local read "Wave In Fs"() -> (w1727:dbl)
        n1051 = local read "Analysis"() -> (w1731:T1)
        n1052 = Bundle By Name(cluster=w1731, "Overlap"=w1725) -> (w1724:T1)
        n1053 = property on="Freq.Resolution(Hz)" class="DigNum (strict)"() -> ("Value"=w1726:dbl)  [unwired: 2 in, 2 out]
        n1054 = call "CRYGet Frequency Resolution Param.vi"("Overlap(%)"=w1725, "Fs"=w1727, "Freq Resolution(Hz)"=w1726, "Samples"=w1728) -> ("No. of FFT"=w1730:i32, "Record Length(s)"=w1729:dbl)  [unwired: 4 in, 2 out]
        n1055 = local write "Analysis"(w1724) -> ()
        n1056 = property on="Record Length (s)" class="DigNum (strict)"("Value"=w1729) -> ()  [unwired: 2 in, 2 out]
        n1057 = property on="No.of FFTs" class="DigNum (strict)"("Value"=w1730) -> ()  [unwired: 2 in, 2 out]
      }
      event "Fmin(Hz)": Value Change {
        n1058 = event-data() -> ("NewVal"=w1734:dbl)  [unwired: 6 out]
        n1059 = Less?(x=w1734, y=0.0) -> (x < y?=w1736:bool)
        n1060 = Select(t=0.0, s=w1736, f=w1734) -> (s? t:f=w1733:dbl)
        n1061 = property on="Fmin(Hz)" class="DigNum (strict)"("Value"=w1733) -> ()  [unwired: 2 in, 2 out]
        n1062 = local read "Analysis"() -> (w1738:T1)
        n1063 = Bundle By Name(cluster=w1738, "Fmin(Hz)"=w1733) -> (w1732:T1)
        n1064 = local write "Analysis"(w1732) -> ()
      }
      event "Fmax(Hz)": Value Change {
        n1065 = event-data() -> ("NewVal"=w1741:dbl)  [unwired: 6 out]
        n1066 = Less?(x=w1741, y=0.0) -> (x < y?=w1743:bool)
        n1067 = Select(t=0.0, s=w1743, f=w1741) -> (s? t:f=w1740:dbl)
        n1068 = property on="Fmax(Hz)" class="DigNum (strict)"("Value"=w1740) -> ()  [unwired: 2 in, 2 out]
        n1069 = local read "Analysis"() -> (w1745:T1)
        n1070 = Bundle By Name(cluster=w1745, "Fmax(Hz)"=w1740) -> (w1739:T1)
        n1071 = local write "Analysis"(w1739) -> ()
      }
      event "Scaling": Value Change {
        n1072 = event-data() -> ("NewVal"=w1747:i32)  [unwired: 6 out]
        n1073 = local read "Analysis"() -> (w1748:T1)
        n1074 = Bundle By Name(cluster=w1748, "Scaling"=w1747) -> (w1746:T1)
        n1075 = local write "Analysis"(w1746) -> ()
      }
      event "Discard Cycles": Value Change {
        n1076 = event-data() -> ("NewVal"=w1750:dbl)  [unwired: 6 out]
        n1077 = local read "Analysis"() -> (w1751:T1)
        n1078 = Bundle By Name(cluster=w1751, "discard cycles"=w1750) -> (w1749:T1)
        n1079 = local write "Analysis"(w1749) -> ()
      }
      event "Spectral Scaling*": Value Change {
        n1080 = event-data() -> ("NewVal"=w1753:u16)  [unwired: 6 out]
        n1081 = local read "Analysis"() -> (w1754:T1)
        n1082 = Bundle By Name(cluster=w1754, "Spectral Scaling"=w1753) -> (w1752:T1)
        n1083 = local write "Analysis"(w1752) -> ()
      }
      event "Auto-Spectrum(Stimulus)*": Value Change {
        n1084 = event-data() -> ("NewVal"=w1755:bool)  [unwired: 6 out]
        n1085 = flat-sequence {
          tunnel: w1755 -> [w1757]
          frame #0 {
            n1086 = local read "Analysis"() -> (w1758:T1)
            n1087 = Bundle By Name(cluster=w1758, "Auto Spectrum(Stimulus)*"=w1757) -> (w1756:T1)
            n1088 = local write "Analysis"(w1756) -> ()
          }
          frame #1 {
            n1089 = property on="CurveUpdate" class="Bool (strict)"("Val(Sgnl)"=TRUE ("Value (Signaling)")) -> ()  [unwired: 2 in, 2 out]
          }
        }
      }
      event "Auto-Spectrum(Response)*": Value Change {
        n1090 = event-data() -> ("NewVal"=w1760:bool)  [unwired: 6 out]
        n1091 = flat-sequence {
          tunnel: w1760 -> [w1762]
          frame #0 {
            n1092 = local read "Analysis"() -> (w1763:T1)
            n1093 = Bundle By Name(cluster=w1763, "Auto Spectrum(Response)*"=w1762) -> (w1761:T1)
            n1094 = local write "Analysis"(w1761) -> ()
          }
          frame #1 {
            n1095 = property on="CurveUpdate" class="Bool (strict)"("Val(Sgnl)"=TRUE ("Value (Signaling)")) -> ()  [unwired: 2 in, 2 out]
          }
        }
      }
      event "Cross-Spectrum*": Value Change {
        n1096 = event-data() -> ("NewVal"=w1765:bool)  [unwired: 6 out]
        n1097 = flat-sequence {
          tunnel: w1765 -> [w1767]
          frame #0 {
            n1098 = local read "Analysis"() -> (w1768:T1)
            n1099 = Bundle By Name(cluster=w1768, "Cross Spectrum*"=w1767) -> (w1766:T1)
            n1100 = local write "Analysis"(w1766) -> ()
          }
          frame #1 {
            n1101 = property on="CurveUpdate" class="Bool (strict)"("Val(Sgnl)"=TRUE ("Value (Signaling)")) -> ()  [unwired: 2 in, 2 out]
          }
        }
      }
      event "Coherent Power*": Value Change {
        n1102 = event-data() -> ("NewVal"=w1770:bool)  [unwired: 6 out]
        n1103 = flat-sequence {
          tunnel: w1770 -> [w1772]
          frame #0 {
            n1104 = local read "Analysis"() -> (w1773:T1)
            n1105 = Bundle By Name(cluster=w1773, "Coherent Power*"=w1772) -> (w1771:T1)
            n1106 = local write "Analysis"(w1771) -> ()
          }
          frame #1 {
            n1107 = property on="CurveUpdate" class="Bool (strict)"("Val(Sgnl)"=TRUE ("Value (Signaling)")) -> ()  [unwired: 2 in, 2 out]
          }
        }
      }
      event "Non-Coherent Power*": Value Change {
        n1108 = event-data() -> ("NewVal"=w1775:bool)  [unwired: 6 out]
        n1109 = flat-sequence {
          tunnel: w1775 -> [w1777]
          frame #0 {
            n1110 = local read "Analysis"() -> (w1778:T1)
            n1111 = Bundle By Name(cluster=w1778, "Non-Coherent Power*"=w1777) -> (w1776:T1)
            n1112 = local write "Analysis"(w1776) -> ()
          }
          frame #1 {
            n1113 = property on="CurveUpdate" class="Bool (strict)"("Val(Sgnl)"=TRUE ("Value (Signaling)")) -> ()  [unwired: 2 in, 2 out]
          }
        }
      }
      event "Frequency Response": Value Change {
        n1114 = event-data() -> ("NewVal"=w1780:bool)  [unwired: 6 out]
        n1115 = flat-sequence {
          tunnel: w1780 -> [w1782]
          frame #0 {
            n1116 = local read "Analysis"() -> (w1783:T1)
            n1117 = Bundle By Name(cluster=w1783, "Frequency Response"=w1782) -> (w1781:T1)
            n1118 = local write "Analysis"(w1781) -> ()
          }
          frame #1 {
            n1119 = property on="CurveUpdate" class="Bool (strict)"("Val(Sgnl)"=TRUE ("Value (Signaling)")) -> ()  [unwired: 2 in, 2 out]
          }
        }
      }
      event "Coherence (%)": Value Change {
        n1120 = event-data() -> ("NewVal"=w1785:bool)  [unwired: 6 out]
        n1121 = flat-sequence {
          tunnel: w1785 -> [w1787]
          frame #0 {
            n1122 = local read "Analysis"() -> (w1788:T1)
            n1123 = Bundle By Name(cluster=w1788, "Coherence (%)"=w1787) -> (w1786:T1)
            n1124 = local write "Analysis"(w1786) -> ()
          }
          frame #1 {
            n1125 = property on="CurveUpdate" class="Bool (strict)"("Val(Sgnl)"=TRUE ("Value (Signaling)")) -> ()  [unwired: 2 in, 2 out]
          }
        }
      }
      event "Non-Coherence (%)": Value Change {
        n1126 = event-data() -> ("NewVal"=w1790:bool)  [unwired: 6 out]
        n1127 = flat-sequence {
          tunnel: w1790 -> [w1792]
          frame #0 {
            n1128 = local read "Analysis"() -> (w1793:T1)
            n1129 = Bundle By Name(cluster=w1793, "Non-Coherence (%)"=w1792) -> (w1791:T1)
            n1130 = local write "Analysis"(w1791) -> ()
          }
          frame #1 {
            n1131 = property on="CurveUpdate" class="Bool (strict)"("Val(Sgnl)"=TRUE ("Value (Signaling)")) -> ()  [unwired: 2 in, 2 out]
          }
        }
      }
      event "Averaging Time(s)": Value Change {
        n1132 = event-data() -> ("NewVal"=w1797:dbl)  [unwired: 6 out]
        n1133 = Less?(x=w1797, y=0.0) -> (x < y?=w1799:bool)
        n1134 = Select(t=0.0, s=w1799, f=w1797) -> (s? t:f=w1796:dbl)
        n1135 = property on="Averaging Time(s)" class="DigNum (strict)"("Value"=w1796) -> ()  [unwired: 2 in, 2 out]
        n1136 = local read "Analysis"() -> (w1801:T1)
        n1137 = Bundle By Name(cluster=w1801, "Averaging Time"=w1796) -> (w1795:T1)
        n1138 = local write "Analysis"(w1795) -> ()
      }
      event "Max duration(s)": Value Change {
        n1139 = event-data() -> ("NewVal"=w1804:dbl)  [unwired: 6 out]
        n1140 = Less?(x=w1804, y=0.0) -> (x < y?=w1806:bool)
        n1141 = Select(t=0.0, s=w1806, f=w1804) -> (s? t:f=w1803:dbl)
        n1142 = local read "Analysis"() -> (w1808:T1)
        n1143 = Bundle By Name(cluster=w1808, "Max duration"=w1803) -> (w1802:T1)
        n1144 = property on="Max duration(s)" class="DigNum (strict)"("Value"=w1803) -> ()  [unwired: 2 in, 2 out]
        n1145 = local write "Analysis"(w1802) -> ()
      }
      event "Attack Threshold(dB)": Value Change {
        n1146 = event-data() -> ("NewVal"=w1810:dbl)  [unwired: 6 out]
        n1147 = local read "Analysis"() -> (w1811:T1)
        n1148 = Bundle By Name(cluster=w1811, "Attack Threshold"=w1810) -> (w1809:T1)
        n1149 = local write "Analysis"(w1809) -> ()
      }
      event "Min duration(s)": Value Change {
        n1150 = event-data() -> ("NewVal"=w1814:dbl)  [unwired: 6 out]
        n1151 = Less?(x=w1814, y=0.0) -> (x < y?=w1816:bool)
        n1152 = Select(t=0.0, s=w1816, f=w1814) -> (s? t:f=w1813:dbl)
        n1153 = property on="Min duration(s)" class="DigNum (strict)"("Value"=w1813) -> ()  [unwired: 2 in, 2 out]
        n1154 = local read "Analysis"() -> (w1818:T1)
        n1155 = Bundle By Name(cluster=w1818, "Min duration"=w1813) -> (w1812:T1)
        n1156 = local write "Analysis"(w1812) -> ()
      }
      event "Hysteresis Up(dB)": Value Change {
        n1157 = event-data() -> ("NewVal"=w1820:dbl)  [unwired: 6 out]
        n1158 = local read "Analysis"() -> (w1821:T1)
        n1159 = Bundle By Name(cluster=w1821, "Hysteresis Up"=w1820) -> (w1819:T1)
        n1160 = local write "Analysis"(w1819) -> ()
      }
      event "Signal-Noise Ratio (dB)": Value Change {
        n1161 = event-data() -> ("NewVal"=w1822:bool)  [unwired: 6 out]
        n1162 = flat-sequence {
          tunnel: w1822 -> [w1824]
          frame #0 {
            n1163 = local read "Analysis"() -> (w1825:T1)
            n1164 = Bundle By Name(cluster=w1825, "Signal-Noise Ratio (dB)"=w1824) -> (w1823:T1)
            n1165 = local write "Analysis"(w1823) -> ()
          }
          frame #1 {
            n1166 = property on="CurveUpdate" class="Bool (strict)"("Val(Sgnl)"=TRUE ("Value (Signaling)")) -> ()  [unwired: 2 in, 2 out]
          }
        }
      }
      event "Non-Coherent Distortion*": Value Change {
        n1167 = event-data() -> ("NewVal"=w1827:bool)  [unwired: 6 out]
        n1168 = flat-sequence {
          tunnel: w1827 -> [w1829]
          frame #0 {
            n1169 = local read "Analysis"() -> (w1830:T1)
            n1170 = Bundle By Name(cluster=w1830, "Non-Coherenct Distirtion*"=w1829) -> (w1828:T1)
            n1171 = local write "Analysis"(w1828) -> ()
          }
          frame #1 {
            n1172 = property on="CurveUpdate" class="Bool (strict)"("Val(Sgnl)"=TRUE ("Value (Signaling)")) -> ()  [unwired: 2 in, 2 out]
          }
        }
      }
      event "Record Length (s)": Value Change {
        n1173 = event-data() -> ("NewVal"=w1833:dbl)  [unwired: 6 out]
        n1174 = local read "Analysis"() -> (w1834:T1)
        n1175 = Bundle By Name(cluster=w1834, "Record Length"=w1833) -> (w1832:T1)
        n1176 = local write "Analysis"(w1832) -> ()
      }
      event "No.of FFTs": Value Change {
        n1177 = event-data() -> ("NewVal"=w1836:i32)  [unwired: 6 out]
        n1178 = local read "Analysis"() -> (w1837:T1)
        n1179 = Bundle By Name(cluster=w1837, "No.of FFTs"=w1836) -> (w1835:T1)
        n1180 = local write "Analysis"(w1835) -> ()
      }
      event "Windowed Resolution(Hz)": Value Change {
        n1181 = event-data() -> ("NewVal"=w1839:dbl)  [unwired: 6 out]
        n1182 = local read "Analysis"() -> (w1840:T1)
        n1183 = Bundle By Name(cluster=w1840, "Win Resolution"=w1839) -> (w1838:T1)
        n1184 = local write "Analysis"(w1838) -> ()
      }
      event "Help": Value Change {
        n1185 = event-data() -> ("NewVal"=w1842:string)  [unwired: 6 out]
        n1186 = local read "Analysis"() -> (w1843:T1)
        n1187 = Bundle By Name(cluster=w1843, "Help"=w1842) -> (w1841:T1)
        n1188 = local write "Analysis"(w1841) -> ()
      }
    }
    n1189 = global read "CRYMainGlobal.vi" "STOP"() -> (w53:bool)
    n1190 = Compound Arithmetic op=OR(w53, "stop") -> (w44:bool)
    n1191 = Compound Arithmetic op=OR("Manual Apply", "Apply") -> (w43:bool)
    n1192 = Bundle(w43, "units"="units", "Edit List"="Edit List", "Load Test"="Load Test", "Add Lib"="Add Lib", "OK"="OK", "Cancel"="Cancel") -> (w62:T23)  [unwired: 1 out]
    n1193 = Cluster To Array(cluster=w62) -> (array=w61:bool[])
    n1194 = Search 1D Array(1D array=w61, element=TRUE) -> (index of element=w59:i32)  [unwired: 1 out]
    n1195 = case shown="4" w59 {
      tunnel: w57 -> [w69 _ _ _ _ _ _ _]
      tunnel: w51 -> [w68 _ _ _ _ _ _ _]
      tunnel: w55 -> [_ _ _ w216 _ _ _ _]
      tunnel: w40 -> [_ _ _ w215 _ _ _ _]
      tunnel: w39 -> [_ _ _ w214 _ _ _ _]
      frame 0 {
        n1196 = global read "CRYMainGlobal.vi" "Access Level"() -> (w66:enum16{"Engineer", "Technician", "Operator"})
        n1197 = property on="Manual Apply" class="Bool (strict)"("Value"=FALSE ("Manual Apply")) -> ()  [unwired: 2 in, 2 out]
        n1198 = case shown="\"Operator\", Default" w66 {
          tunnel: w69 -> [w79 _]
          tunnel: w68 -> [w78 _]
          frame "Engineer" {
            n1199 = local read "Proper VI No"() -> (w73:i32)
            n1200 = local read "Analysis"() -> (w70:T1)
            n1201 = call "CRYFlatten Analysis.vi"("Analysis"=w70) -> ("Analysis flattened"=w76:string)  [unwired: 10 out]
            n1202 = Build Array(w73) -> (w74:i32[])
            n1203 = call "CRYGet Curve Library Data Name.vi"("nData"=w74, "sAction"="GetNamebyStep" ("sOption")) -> ("sNames"=w72:string[], "Type Out"=w71:string[])  [unwired: 6 in, 2 out]
            n1204 = call "CRYTest Input Param.vi"("Flattend Analysis"=w76) -> ("test result"=w77:bool)  [unwired: 10 out]
            n1205 = case shown="True" w77 {
              tunnel: w79 -> [_ w93]
              tunnel: w78 -> [_ w92]
              tunnel: w76 -> [_ w91]
              tunnel: w72 -> [_ w90]
              tunnel: w71 -> [_ w88]
              tunnel: w70 -> [_ w86]
              frame False {
                n1206 = local write "Apply"(FALSE ("Apply")) -> ()
              }
              frame True {
                n1207 = flat-sequence {
                  tunnel: w91 -> [w95]
                  tunnel: [w95] -> w85
                  tunnel: w93 -> [w105]
                  tunnel: w92 -> [w104]
                  tunnel: [w101] -> w89
                  tunnel: [w100] -> w87
                  tunnel: w85 -> [w99]
                  tunnel: [w99] -> w83
                  tunnel: [w98] -> w81
                  tunnel: w90 -> [w111]
                  tunnel: w89 -> [w110]
                  tunnel: w88 -> [w109]
                  tunnel: w87 -> [w108]
                  tunnel: [w107] -> w84
                  tunnel: w83 -> [w107]
                  tunnel: [w106] -> w82
                  tunnel: w81 -> [w106]
                  tunnel: w86 -> [w126]
                  tunnel: w84 -> [w123]
                  tunnel: w82 -> [w122]
                  frame #0 {
                    n1208 = property on="Changed Curve" class="Arr (strict)"() -> ("Value"=w94:string[][])  [unwired: 2 in, 2 out]
                    n1209 = global write "CRYMainGlobal.vi" "Changed Curve State"(w94) -> ()
                  }
                  frame #1 {
                    n1210 = call "CRYGet Current TS Steps.vi"() -> ("SelectStepNumber in Tree"=w102:i32, "Steps"=w103:T4[])  [unwired: 1 in, 9 out]
                    n1211 = Index Array(array=w103, index=w102) -> (element=w97:T4)
                    n1212 = Bundle By Name(cluster=w97, "Seq setup flattened"=w99) -> (w98:T4)
                    n1213 = Unbundle By Name(w97) -> ("StepName"=w96:string)
                    n1214 = call "CRYAnalysis.vi"("Setup in"=w98, "Step name"=w96, "Hardware in"=w105, "Calibration in"=w104) -> ("Types Out"=w100:string[], "Inserted Names Out"=w101:string[])  [unwired: 3 in, 7 out]
                  }
                  frame #2 {
                    n1215 = disable-structure shown="Enabled" {
                      disable-tunnel: w111 -> [w113 w117]
                      disable-tunnel: w110 -> [w112 w118]
                      disable-tunnel: w109 -> [_ w116]
                      disable-tunnel: w108 -> [_ w115]
                      frame Disabled {
                        n1216 = call "CRYReplace Curve Name of Steps.vi"("Step Category"="Analysis", "New Name"=w112, "Old Name"=w113) -> ()  [unwired: 8 in, 1 out]
                      }
                      frame Enabled {
                        n1217 = call "CRYChange Name by Step Editor.vi"("New Names Type"=w115, "Old Names Type"=w116, "Old Names"=w117, "New Names"=w118) -> ()  [unwired: 8 in]
                      }
                    }
                  }
                  frame #3 {
                    n1218 = Unbundle By Name(w126) -> ()  [unwired: 1 out]
                    n1219 = property on="Delay Method" class="Slide (strict)"() -> ("Value"=w129:u16)  [unwired: 2 in, 2 out]
                    n1220 = call "CRYReplace Analysis Curve Name.vi"("Setup in"=w122, "Step Setup In"=w123, "InsertSocket?"=FALSE, "Type In"="AddStep") -> ("New Custom Name( Channel case)"=w119:string[], "Signal Type"=w120:string, "New Custom Type( Channel case)"=w121:string[])  [unwired: 3 in, 2 out]
                    n1221 = call "CRYGet Changed Ana Curve Name.vi"("Old Name"=w119, "Signal Tyep"=w120, "Current Name"=w119, "New Custom Type( Channel case)"=w121, "Load?"=TRUE) -> ("Changed Name Table  out"=w128:string[][])  [unwired: 10 in]
                    n1222 = property on="Delay Treat" class="Slide (strict)"("Val(Sgnl)"=w129) -> ()  [unwired: 2 in, 2 out]
                    n1223 = property on="Changed Curve" class="Arr (strict)"("Value"=w128) -> ()  [unwired: 2 in, 2 out]
                    n1224 = property on="Old Name" class="Arr (strict)"("Value"=w119) -> ()  [unwired: 2 in, 2 out]
                  }
                  frame #4 {
                    n1225 = local write "Apply"(FALSE ("Apply")) -> ()
                  }
                }
              }
            }
          }
          frame "Operator", Default {
            n1226 = call "CRYGet Error Message.vi"("Kind"="Step Setup") -> ("Window Title"=w132:string)  [unwired: 5 in, 5 out]
            n1227 = call "CRYGet Access Level Message.vi"() -> ("Multibyte string"=w134:string)  [unwired: 11 in]
            n1228 = call "CRYMessage Dialog.vi"("Window Title"=w132, "YesNoCancel"=T7."OK", "Message Content"=w134) -> ()  [unwired: 7 in, 2 out]
            n1229 = local write "Apply"(FALSE ("Apply")) -> ()
          }
        }
      }
      frame 1 {
        n1230 = local read "Analysis"() -> (w140:T1)
        n1231 = Unbundle By Name(w140) -> ("use custom unit"=w139:bool)
        n1232 = Bundle("Scale visible?"=TRUE, "use custom unit"=w139) -> (w137:T24)  [unwired: 1 out]
        n1233 = local read "Common dB #"() -> (w143:u16)
        n1234 = local read "Y prefix"() -> (w146:string)
        n1235 = local read "Y unit"() -> (w145:string)
        n1236 = local read "Y data"() -> (w147:u16)
        n1237 = local read "Y dB ref"() -> (w144:dbl)
        n1238 = call "CRYUnits setup.vi"("unit prefix"=w146, "Scale visible?"=TRUE, "dB/Lin"=w147, "Unit:"=w145, "dB ref:"=w144, "Custom unit settings"=w137, "Common dB ref."=w143) -> ("New Scale"=w152:u16, "New unit prefix Lin"=w151:string, "New unit Lin"=w142:string, "New dB ref"=w150:dbl, "Common dB #"=w149:u16, "Use custom unit out"=w141:bool)  [unwired: 1 in, 2 out]
        n1239 = local write "Common dB #"(w149) -> ()
        n1240 = local write "Y prefix"(w151) -> ()
        n1241 = local write "Y data"(w152) -> ()
        n1242 = local write "Y dB ref"(w150) -> ()
        n1243 = local write "Y unit"(w142) -> ()
        n1244 = case shown="..0" w152 {
          tunnel: ["dB" w155] -> w136
          tunnel: w142 -> [_ w155]
          frame ..0 {
          }
          frame 1.. {
          }
        }
        n1245 = Bundle By Name(cluster=w140, "Y data"=w152, "Y prefix"=w151, "Y unit"=w142, "Y dB ref"=w150, "Unit"=w136, "use custom unit"=w141) -> (w153:T1)
        n1246 = local write "Unit"(w136) -> ()
        n1247 = property on="Analysis" class="Clust (strict)"("Val(Sgnl)"=w153) -> ()  [unwired: 2 in, 2 out]
      }
      frame 2 {
        n1248 = local read "Type"() -> (w156:u16)
        n1249 = case shown="2" w156 {
          frame 0, Default {
            n1250 = local read "har checkoffs"() -> (w159:bool[])
            n1251 = property on="Harmonics" class="LstBox (strict)"() -> ("Item Names"=w160:string[])  [unwired: 2 in, 2 out]
            n1252 = case shown="True" TRUE {
              tunnel: w159 -> [_ w175]
              tunnel: w160 -> [_ w174]
              tunnel: [bool[] [] ("Checkoffs out") w172] -> w157
              tunnel: [string[] [] ("Items out") w171] -> w158
              frame False {
              }
              frame True {
                n1253 = call "CRYHarmonics list editor.vi"("Checkoffs"=w175, "Items"=w174) -> ("Checkoffs out"=w172:bool[], "Symbols out"=w173:i32[], "Items out"=w171:string[])  [unwired: 7 out]
                n1254 = local write "har checkoffs"(w172) -> ()
                n1255 = property on="Harmonics" class="LstBox (strict)"("Item Names"=w171, "Item Symbols"=w173) -> ()  [unwired: 2 in, 2 out]
              }
            }
            n1256 = flat-sequence {
              tunnel: w158 -> [w165]
              tunnel: w157 -> [w164]
              frame #0 {
                n1257 = call "CRYHarmonics list to array.vi"("Checkoffs"=w164, "Harmonic list items"=w165) -> ("List items checked"=w166:string[], "Harmonics array out"=w163:dbl[])  [unwired: 8 out]
                n1258 = local write "Harmonics array out"(w163) -> ()
                n1259 = local read "Analysis"() -> (w167:T1)
                n1260 = Bundle By Name(cluster=w167, "Harmonics"=w163, "har list items"=w166) -> (w162:T1)
                n1261 = local write "Analysis"(w162) -> ()
              }
              frame #1 {
                n1262 = property on="CurveUpdate" class="Bool (strict)"("Val(Sgnl)"=TRUE ("Value (Signaling)")) -> ()  [unwired: 2 in, 2 out]
              }
            }
          }
          frame 1 {
            n1263 = local read "IM checkoffs"() -> (w176:bool[])
            n1264 = property on="Orders IM" class="LstBox (strict)"() -> ("Item Names"=w179:string[])  [unwired: 2 in, 2 out]
            n1265 = case shown="True" TRUE {
              tunnel: w179 -> [_ w194]
              tunnel: w176 -> [_ w193]
              tunnel: [string[] [] ("Items out") w192] -> w178
              tunnel: [bool[] [] ("Checkoffs out") w190] -> w177
              frame False {
              }
              frame True {
                n1266 = call "CRYHarmonics list editor.vi"("Checkoffs"=w193, "Items"=w194) -> ("Checkoffs out"=w190:bool[], "Symbols out"=w191:i32[], "Items out"=w192:string[])  [unwired: 7 out]
                n1267 = local write "IM checkoffs"(w190) -> ()
                n1268 = property on="Orders IM" class="LstBox (strict)"("Item Names"=w192, "Item Symbols"=w191) -> ()  [unwired: 2 in, 2 out]
              }
            }
            n1269 = flat-sequence {
              tunnel: w178 -> [w184]
              tunnel: w177 -> [w183]
              frame #0 {
                n1270 = call "CRYHarmonics list to array.vi"("Checkoffs"=w183, "Harmonic list items"=w184) -> ("List items checked"=w185:string[], "Harmonics array out"=w182:dbl[])  [unwired: 8 out]
                n1271 = local write "IM array out"(w182) -> ()
                n1272 = local read "Analysis"() -> (w186:T1)
                n1273 = Bundle By Name(cluster=w186, "Intermod"=w182, "IM list items"=w185) -> (w181:T1)
                n1274 = local write "Analysis"(w181) -> ()
              }
              frame #1 {
                n1275 = property on="CurveUpdate" class="Bool (strict)"("Val(Sgnl)"=TRUE ("Value (Signaling)")) -> ()  [unwired: 2 in, 2 out]
              }
            }
          }
          frame 2 {
            n1276 = local read "Diff checkoffs"() -> (w195:bool[])
            n1277 = property on="Orders Diff" class="LstBox (strict)"() -> ("Item Names"=w198:string[])  [unwired: 2 in, 2 out]
            n1278 = case shown="True" TRUE {
              tunnel: w198 -> [_ w213]
              tunnel: w195 -> [_ w212]
              tunnel: [string[] [] ("Items out") w211] -> w197
              tunnel: [bool[] [] ("Checkoffs out") w209] -> w196
              frame False {
              }
              frame True {
                n1279 = call "CRYHarmonics list editor.vi"("Checkoffs"=w212, "Items"=w213) -> ("Checkoffs out"=w209:bool[], "Symbols out"=w210:i32[], "Items out"=w211:string[])  [unwired: 7 out]
                n1280 = local write "Diff checkoffs"(w209) -> ()
                n1281 = property on="Orders Diff" class="LstBox (strict)"("Item Names"=w211, "Item Symbols"=w210) -> ()  [unwired: 2 in, 2 out]
              }
            }
            n1282 = flat-sequence {
              tunnel: w197 -> [w203]
              tunnel: w196 -> [w202]
              frame #0 {
                n1283 = call "CRYHarmonics list to array.vi"("Checkoffs"=w202, "Harmonic list items"=w203) -> ("List items checked"=w204:string[], "Harmonics array out"=w201:dbl[])  [unwired: 8 out]
                n1284 = local write "Diff array out"(w201) -> ()
                n1285 = local read "Analysis"() -> (w205:T1)
                n1286 = Bundle By Name(cluster=w205, "Diff"=w201, "Diff list items"=w204) -> (w200:T1)
                n1287 = local write "Analysis"(w200) -> ()
              }
              frame #1 {
                n1288 = property on="CurveUpdate" class="Bool (strict)"("Val(Sgnl)"=TRUE ("Value (Signaling)")) -> ()  [unwired: 2 in, 2 out]
              }
            }
          }
        }
      }
      frame 3 {
        n1289 = stacked-sequence {
          seq-local: [_ w338 _ _] -> [_ _ w427 _]
          seq-local: [_ w339 _ _] -> [_ _ w426 _]
          seq-local: [_ w332 _ _] -> [_ _ w425 _]
          tunnel: w216 -> [_ _ _ _]
          tunnel: w215 -> [_ _ _ _]
          tunnel: w214 -> [w217 _ _ _]
          frame #0 {
            n1290 = local read "Analysis"() -> (w236:T1)
            n1291 = call "CRYFlatten Analysis.vi"("Analysis"=w236) -> ("Analysis flattened"=w229:string)  [unwired: 10 in]
            n1292 = call "CRYGet Current TS Steps.vi"() -> ("SelectStepNumber in Tree"=w226:i32, "Steps"=w227:T4[])  [unwired: 1 in, 9 out]
            n1293 = flat-sequence {
              tunnel: w238 -> [w249]
              tunnel: w239 -> [w246]
              tunnel: w240 -> [w245]
              frame #0 {
                n1294 = property on="Changed Curve 2" class="Arr (strict)"() -> ("Value"=w251:string[][])  [unwired: 2 in, 2 out]
                n1295 = property on="Change Curve Name?" class="Bool (strict)"() -> ("Value"=w253:bool)  [unwired: 2 in, 2 out]
                n1296 = property on="Change Use Channel?" class="Bool (strict)"() -> ("Value"=w248:bool)  [unwired: 2 in, 2 out]
                n1297 = property on="Old Name" class="Arr (strict)"() -> ("Value"=w250:string[])  [unwired: 2 in, 2 out]
                n1298 = property on="Use Channel Name" class="Bool (strict)"() -> ("Value"=w247:bool)  [unwired: 2 in, 2 out]
                n1299 = call "CRYGet Changed Ana Curve Name.vi"("Old Name"=w250, "Signal Tyep"=w246, "Use Channel Name?"=w247, "Current Name"=w249, "Changed Name Table in"=w251, "New Custom Type( Channel case)"=w245, "Change State"=w253, "Change Use Channel"=w248) -> ("Changed Name Table  out"=→"Changed Curve 2":string[][])  [unwired: 7 in]
                n1300 = property on="Old Name" class="Arr (strict)"("Value"=w249) -> ()  [unwired: 2 in, 2 out]
              }
              frame #1 {
                n1301 = property on="Change Curve Name?" class="Bool (strict)"("Value"=FALSE ("Change Curve Name?")) -> ()  [unwired: 2 in, 2 out]
                n1302 = property on="Change Use Channel?" class="Bool (strict)"("Value"=FALSE ("Change Use Channel?")) -> ()  [unwired: 2 in, 2 out]
              }
            }
            n1303 = Index Array(array=w227, index=w226) -> (element=w225:T4)
            n1304 = call "CRYReplace Analysis Curve Name.vi"("Setup in"=w225, "Step Setup In"=w229, "InsertSocket?"=FALSE, "Type In"="AddStep") -> ("New Custom Name( Channel case)"=w238:string[], "Signal Type"=w239:string, "Curve Info Array Out"=w224:T14, "New Custom Type( Channel case)"=w240:string[])  [unwired: 3 in, 1 out]
            n1305 = for {
              tunnel: w224 -> [w259] mode=indexing
              tunnel: [w258] -> w237 mode=indexing
              tunnel: [w257] -> w231 mode=indexing
              tunnel: [w256] -> w232 mode=indexing
              n1306 = Unbundle By Name(w259) -> ("Custom Curve Names"=w258:string, "Custom Curve IDs"=w257:i32, "Default Curve Names"=w256:string)
            }
            n1307 = Bundle By Name(cluster=w236, "Custom Curve Names"=w237, "Custom Curve IDs"=w231, "Default Curve Names"=w232) -> (w235:T1)
            n1308 = call "CRYGet Upper Step Data.vi"("Type In"=enum16{"Curves", "Values", "Results", "WFM"}."WFM" ("Type"), "No.VI"=w217) -> ("Waveform Array"=w219:T12)  [unwired: 6 in, 3 out]
            n1309 = call "CRYGet Upper Step Data.vi"("Type In"=enum16{"Curves", "Values", "Results", "WFM"}."Values", "No.VI"=w217) -> ("Value array"=w221:T5)  [unwired: 9 out]
            n1310 = for {
              tunnel: w219 -> [w244] mode=indexing
              tunnel: [w243] -> w218 mode=indexing
              n1311 = Unbundle By Name(w244) -> ("Name"=w243:string)
            }
            n1312 = for {
              tunnel: w221 -> [w242] mode=indexing
              tunnel: [w241] -> w223 mode=indexing
              n1313 = Unbundle By Name(w242) -> ("Name"=w241:string)
            }
            n1314 = Build Array(w237) -> (w233:string[][])
            n1315 = local write "Analysis"(w235) -> ()
            n1316 = Transpose 2D Array(2D array=w233) -> (transposed array=w234:string[][])
            n1317 = property on="LR" class="Ring (strict)"("Strings []"=w223) -> ()  [unwired: 2 in, 2 out]
            n1318 = property on="Waveforms Out" class="Ring (strict)"("Strings []"=w218) -> ()  [unwired: 2 in, 2 out]
            n1319 = property on="Waveforms In" class="Ring (strict)"("Strings []"=w218) -> ()  [unwired: 2 in, 2 out]
            n1320 = property on="Custom Curve Names" class="Tbl (strict)"("Value"=w234) -> ()  [unwired: 2 in, 2 out]
          }
          frame #1 {
            n1321 = local read "Analysis"() -> (w284:T1)
            n1322 = Unbundle By Name(w284) -> ("Harmonics"=w338:dbl[], "har list items"=w410:string[], "THD(%)"=w408:bool, "Rub&Buzz"=w409:bool, "discard cycles"=w401:dbl, "Imp Ref resistor"=w400:dbl, "Y data"=w399:u16, "Y prefix"=w398:string, "Y unit"=w397:string, "Y dB ref"=w396:dbl, "autodelay ch"=w395:dbl, "stop ms"=w394:dbl, "Apply Correction Out"=w390:bool, "Apply Correction In"=w389:bool, "Harmonics @ meas.frq"=w388:bool, "THD Normalized(%)"=w387:bool, "Total Distortion"=w386:bool, "THD+Noise(%)"=w385:bool, "Rub&Buzz Norm'd(%)"=w384:bool, "Perceptual Rub&Buzz"=w306:bool, "Standard Error"=w307:bool, "Confidence Limits"=w383:bool, "Method"=w381:u16, "Total Noise"=w382:bool, "Total DFD(%)"=w378:bool, "Total IMD(%)"=w379:bool, "Total IM"=w380:bool, "Total DFD+Noise(%)"=w377:bool, "Total Diff"=w376:bool, "Std Err"=w279:dbl, "Fmin(Hz)"=w374:dbl, "Fmax(Hz)"=w373:dbl, "Freq.Resolution"=w372:dbl, "Overlap"=w371:dbl, "Weigting"=w320:string, "TSR Window Type"=w319:string, "Mic Ref resistor"=w280:dbl)
            n1323 = local write "Mic Resistor(ohm)"(w280) -> ()
            n1324 = local write "StopTime(s)"(w394) -> ()
            n1325 = local write "Rub & Buzz Norm'd(%)"(w384) -> ()
            n1326 = local write "Confidence Limits"(w383) -> ()
            n1327 = local write "Apply Correction Out"(w390) -> ()
            n1328 = local write "Apply Correction in"(w389) -> ()
            n1329 = local write "Harmonics @ meas.frq"(w388) -> ()
            n1330 = local write "THD Normalized(%)"(w387) -> ()
            n1331 = local write "Autodelay Channel"(w395) -> ()
            n1332 = local write "Total Distortion"(w386) -> ()
            n1333 = local write "Discard Cycles"(w401) -> ()
            n1334 = local write "Perceptual Rub & Buzz(phons)"(w306) -> ()
            n1335 = local write "Total Noise"(w382) -> ()
            n1336 = local write "Total DFD + Noise(%)"(w377) -> ()
            n1337 = local write "Rub & Buzz(%)"(w409) -> ()
            n1338 = local write "THD + Noise (%)"(w385) -> ()
            n1339 = local write "Total IMD(%)"(w379) -> ()
            n1340 = local write "Total IM"(w380) -> ()
            n1341 = local write "Y unit"(w397) -> ()
            n1342 = local write "Standard Error"(w307) -> ()
            n1343 = local write "Total DFD (%)"(w378) -> ()
            n1344 = local write "Total Diff"(w376) -> ()
            n1345 = local write "THD(%)"(w408) -> ()
            n1346 = local write "Y data"(w399) -> ()
            n1347 = local write "Y prefix"(w398) -> ()
            n1348 = local write "Y dB ref"(w396) -> ()
            n1349 = local write "Method"(w381) -> ()
            n1350 = property on="Harmonics" class="LstBox (strict)"() -> ("Item Names"=w407:string[])  [unwired: 2 in, 2 out]
            n1351 = local write "Reference Resistor(ohm)"(w400) -> ()
            n1352 = call "CRYGet Number to Window.vi"("TSR Window Name"=w319, "Weighting Name"=w320) -> ("TSR window"=w317:u16, "Weighting"=w318:u16)  [unwired: 2 in]
            n1353 = call "CRYHarmonics array to list.vi"("Harmonics array"=w410, "Items"=w407) -> ("Checkoffs out"=w341:bool[], "Symbols out"=w406:i32[], "Items out"=w340:string[])  [unwired: 7 out]
            n1354 = local write "TSR Window Type"(w317) -> ()
            n1355 = local write "Weighting"(w318) -> ()
            n1356 = Max & Min(x=w279, y=1.0) -> (max(x,y)=w277:dbl)  [unwired: 1 out]
            n1357 = local write "har checkoffs"(w341) -> ()
            n1358 = property on="Harmonics" class="LstBox (strict)"("Item Names"=w340, "Item Symbols"=w406) -> ()  [unwired: 2 in, 2 out]
            n1359 = local write "Fmin(Hz)"(w374) -> ()
            n1360 = local write "Fmax(Hz)"(w373) -> ()
            n1361 = local write "Overlap(%)"(w371) -> ()
            n1362 = local write "+/-"(w277) -> ()
            n1363 = local write "Freq.Resolution(Hz)"(w372) -> ()
            n1364 = Unbundle By Name(w284) -> ("IM list items"=w337:string[], "Intermod"=w339:dbl[], "Over-samples Res."=w370:dbl, "Use Channel Name"=w299:bool, "Spectral Scaling"=w369:u16, "Auto Spectrum(Response)*"=w368:bool, "Auto Spectrum(Stimulus)*"=w367:bool, "Cross Spectrum*"=w366:bool, "Coherent Power*"=w359:bool, "Frequency Response"=w360:bool, "Non-Coherent Power*"=w361:bool, "Coherence (%)"=w362:bool, "Non-Coherence (%)"=w363:bool, "Signal-Noise Ratio (dB)"=w364:bool, "Non-Coherenct Distirtion*"=w365:bool, "Averaging Time"=w358:dbl, "Max duration"=w357:dbl, "Min duration"=w356:dbl, "Attack Threshold"=w355:dbl, "Hysteresis Up"=w354:dbl, "Total IMD + Noise(%)"=w352:bool, "Unit"=w316:string, "Appliied Unit"=w350:u16, "Auto-Correlation(Stimulus)"=w349:bool, "Auto-Correlation(Response)"=w348:bool, "Deconvolved Response"=w347:bool, "impulse"=w346:bool, "Cross-Correlation"=w344:bool, "Scaling"=w343:i32, "Loose Particle waveform"=w311:bool, "Curve Resolution"=w275:u16, "Curve Resolution Hz"=w276:dbl, "Polarity"=w274:bool)
            n1365 = property on="Curve Step Resolution" class="Ring (strict)"("Val(Sgnl)"=w275) -> ()  [unwired: 2 in, 2 out]
            n1366 = property on="Polarity" class="Bool (strict)"("Value"=w274) -> ()  [unwired: 2 in, 2 out]
            n1367 = local write "Attack Threshold(dB)"(w355) -> ()
            n1368 = local write "Hysteresis Up(dB)"(w354) -> ()
            n1369 = local write "Over-samples Res.(Hz)"(w370) -> ()
            n1370 = local write "Min duration(s)"(w356) -> ()
            n1371 = local write "Averaging Time(s)"(w358) -> ()
            n1372 = local write "Max duration(s)"(w357) -> ()
            n1373 = local write "Scaling"(w343) -> ()
            n1374 = local write "Unit"(w316) -> ()
            n1375 = local write "Use Channel Name"(w299) -> ()
            n1376 = local write "Non-Coherence (%)"(w363) -> ()
            n1377 = local write "Spectral Scaling*"(w369) -> ()
            n1378 = local write "Cross-Spectrum*"(w366) -> ()
            n1379 = local write "impulse resp?"(w346) -> ()
            n1380 = local write "Cross-Correlation"(w344) -> ()
            n1381 = local write "Coherent Power*"(w359) -> ()
            n1382 = local write "Coherence (%)"(w362) -> ()
            n1383 = local write "Applied Units"(w350) -> ()
            n1384 = property on="Curve Resolution Hz" class="DigNum (strict)"("Value"=w276) -> ()  [unwired: 2 in, 2 out]
            n1385 = local write "Auto-Spectrum(Stimulus)*"(w367) -> ()
            n1386 = local write "Auto-Spectrum(Response)*"(w368) -> ()
            n1387 = local write "Auto-Correlation(Stimulus)"(w349) -> ()
            n1388 = local write "Signal-Noise Ratio (dB)"(w364) -> ()
            n1389 = local write "Non-Coherent Distortion*"(w365) -> ()
            n1390 = local write "Auto-Correlation(Response)"(w348) -> ()
            n1391 = local write "Non-Coherent Power*"(w361) -> ()
            n1392 = local write "Total IMD + Noise(%)"(w352) -> ()
            n1393 = local write "Deconvolved Response"(w347) -> ()
            n1394 = local write "Frequency Response"(w360) -> ()
            n1395 = property on="Loose Particle Waveform" class="Bool (strict)"("Value"=w311) -> ()  [unwired: 2 in, 2 out]
            n1396 = property on="Orders IM" class="LstBox (strict)"() -> ("Item Names"=w336:string[])  [unwired: 2 in, 2 out]
            n1397 = property on="Orders Diff" class="LstBox (strict)"() -> ("Item Names"=w331:string[])  [unwired: 2 in, 2 out]
            n1398 = call "CRYHarmonics array to list.vi"("Harmonics array"=w337, "Items"=w336) -> ("Checkoffs out"=w333:bool[], "Symbols out"=w334:i32[], "Items out"=w335:string[])  [unwired: 7 out]
            n1399 = local write "IM checkoffs"(w333) -> ()
            n1400 = property on="Orders IM" class="LstBox (strict)"("Item Names"=w335, "Item Symbols"=w334) -> ()  [unwired: 2 in, 2 out]
            n1401 = Unbundle By Name(w284) -> ("Custom Curve Names"=w300:string[], "Diff"=w332:dbl[], "Diff list items"=w327:string[], "Algorithm"=w315:u16, "start ms"=w393:dbl, "Win Resolution"=w322:dbl, "Imp"=w392:bool, "Distance Unit"=w391:u16, "delay"=w342:dbl, "ResponseMe"=w353:u16, "Envelope"=w402:bool, "Default Overlap"=w403:bool, "Advanced View"=w405:bool, "Loose Particle"=w312:bool, "Use default"=w313:bool, "Mic Current"=w404:bool, "M List Vaiues"=w351:u16, "Type"=w375:u16, "Delay Method"=w321:u16, "Averaging"=w345:u16, "distance"=w326:dbl, "samples"=w325:dbl, "Record Length"=w324:dbl, "Tab"=w314:i32, "Waveform Out"=w323:string, "Waveform In"=w293:string, "Help"=w310:string, "Imp Auto Mode"=w282:u16, "Mic Auto Mode"=w281:u16)
            n1402 = call "CRYHarmonics array to list.vi"("Harmonics array"=w327, "Items"=w331) -> ("Checkoffs out"=w328:bool[], "Symbols out"=w329:i32[], "Items out"=w330:string[])  [unwired: 7 out]
            n1403 = local write "Diff checkoffs"(w328) -> ()
            n1404 = property on="Orders Diff" class="LstBox (strict)"("Item Names"=w330, "Item Symbols"=w329) -> ()  [unwired: 2 in, 2 out]
            n1405 = property on="Mic Auto Mode" class="Slide (strict)"("Val(Sgnl)"=w281) -> ()  [unwired: 2 in, 2 out]
            n1406 = property on="Amp Auto Mode" class="Slide (strict)"("Val(Sgnl)"=w282) -> ()  [unwired: 2 in, 2 out]
            n1407 = Build Array(w300) -> (w309:string[][])
            n1408 = Transpose 2D Array(2D array=w309) -> (transposed array=w308:string[][])
            n1409 = property on="Default Overlap" class="Bool (strict)"("Val(Sgnl)"=w403) -> ()  [unwired: 2 in, 2 out]
            n1410 = property on="Waveforms In" class="Ring (strict)"() -> ("Strings []"=w264:string[])  [unwired: 2 in, 2 out]
            n1411 = property on="Waveforms Out" class="Ring (strict)"() -> ("Strings []"=w265:string[])  [unwired: 2 in, 2 out]
            n1412 = property on="Help" class="Str"("Value"=w310) -> ()  [unwired: 2 in, 2 out]
            n1413 = property on="Start Time(s)" class="DigNum (strict)"("Value"=w393) -> ()  [unwired: 2 in, 2 out]
            n1414 = property on="Windowed Resolution(Hz)" class="DigNum (strict)"("Value"=w322) -> ()  [unwired: 2 in, 2 out]
            n1415 = property on="Impedance" class="Bool (strict)"("Value"=w392) -> ()  [unwired: 2 in, 2 out]
            n1416 = property on="Distance Unit" class="Ring (strict)"("Value"=w391) -> ()  [unwired: 2 in, 2 out]
            n1417 = property on="s" class="DigNum (strict)"("Value"=w342) -> ()  [unwired: 2 in, 2 out]
            n1418 = property on="Response Measurement1" class="Slide (strict)"("Value"=w353) -> ()  [unwired: 2 in, 2 out]
            n1419 = property on="Envelope?" class="Bool (strict)"("Value"=w402) -> ()  [unwired: 2 in, 2 out]
            n1420 = property on="Advanced View" class="Bool (strict)"("Value"=w405) -> ()  [unwired: 2 in, 2 out]
            n1421 = property on="Loose Particle" class="Bool (strict)"("Value"=w312) -> ()  [unwired: 2 in, 2 out]
            n1422 = property on="Mic Current" class="Bool (strict)"("Value"=w404) -> ()  [unwired: 2 in, 2 out]
            n1423 = property on="Algorithm" class="Ring (strict)"("Value"=w315) -> ()  [unwired: 2 in, 2 out]
            n1424 = property on="Use default" class="Bool (strict)"("Value"=w313) -> ()  [unwired: 2 in, 2 out]
            n1425 = property on="Custom Curve Names" class="Tbl (strict)"("Value"=w308) -> ()  [unwired: 2 in, 2 out]
            n1426 = Search 1D Array(1D array=w264, element=w293) -> (index of element=w269:i32)  [unwired: 1 out]
            n1427 = Search 1D Array(1D array=w265, element=w323) -> (index of element=w267:i32)  [unwired: 1 out]
            n1428 = case shown="False" w313 {
              frame False {
                n1429 = property on="Custom Curve Names" class="Tbl (strict)"("Disabled"=u8 0) -> ()  [unwired: 2 in, 2 out]
              }
              frame True {
                n1430 = property on="Custom Curve Names" class="Tbl (strict)"("Disabled"=u8 2) -> ()  [unwired: 2 in, 2 out]
              }
            }
            n1431 = Less Than 0?(x=w269) -> (x < 0?=w271:bool)
            n1432 = Less Than 0?(x=w267) -> (x < 0?=w266:bool)
            n1433 = local write "Record Length (s)"(w324) -> ()
            n1434 = Select(t=0 ("index of element"), s=w271, f=w269) -> (s? t:f=w260:i32)
            n1435 = Select(t=0 ("index of element"), s=w266, f=w267) -> (s? t:f=w261:i32)
            n1436 = local write "distance"(w326) -> ()
            n1437 = local write "samples"(w325) -> ()
            n1438 = property on="Delay Treat" class="Slide (strict)"("Val(Sgnl)"=w321) -> ()  [unwired: 2 in, 2 out]
            n1439 = property on="Maxis" class="Slide (strict)"("Value"=w351) -> ()  [unwired: 2 in, 2 out]
            n1440 = property on="Type" class="Slide (strict)"("Value"=w375) -> ()  [unwired: 2 in, 2 out]
            n1441 = property on="Averaging1" class="Slide (strict)"("Value"=w345) -> ()  [unwired: 2 in, 2 out]
            n1442 = property on="Main Tab" class="TabCtl (strict)"("Value"=w314) -> ()  [unwired: 2 in, 2 out]
            n1443 = Index Array(array=w264, index=w260) -> (element=w262:string)
            n1444 = Index Array(array=w265, index=w261) -> (element=w263:string)
            n1445 = property on="Delay Method" class="Slide (strict)"("Val(Sgnl)"=w321) -> ()  [unwired: 2 in, 2 out]
            n1446 = call "CRYGet Curve Library Data.vi"("Type"=enum16{"Curves", "Values", "Results", "WFM"}."WFM", "Data Name"=w293) -> ("Wave"=w296:T13)  [unwired: 4 out]
            n1447 = local read "Analysis"() -> (w273:T1)
            n1448 = Bundle By Name(cluster=w273, "Waveform In"=w262, "Waveform Out"=w263) -> (w272:T1)
            n1449 = local read "Mode"() -> (w303:string)
            n1450 = property on="Changed Curve" class="Arr (strict)"() -> ("Value"=w301:string[][])  [unwired: 2 in, 2 out]
            n1451 = property on="Old Name" class="Arr (strict)"() -> ("Value"=w305:string[])  [unwired: 2 in, 2 out]
            n1452 = Unbundle By Name(w296) -> ("Test Info"=w295:string)
            n1453 = call "CRYFlatten Analysis.vi"("Analysis"=w284) -> ("Analysis flattened"=w283:string)  [unwired: 10 in]
            n1454 = case shown="\"Load\", \"Revert\"" w303 {
              tunnel: [TRUE FALSE] -> w302
              frame "False", Default {
              }
              frame "Load", "Revert" {
              }
            }
            n1455 = call "CRYGet Current TS Steps.vi"() -> ("SelectStepNumber in Tree"=w289:i32, "Steps"=w288:T4[])  [unwired: 1 in, 9 out]
            n1456 = local write "Analysis"(w272) -> ()
            n1457 = call "CRYUnflatten Test Infor.vi"("Falattend test infor"=w295) -> ("unflattened test infor data"=w294:T15)  [unwired: 9 out]
            n1458 = Index Array(array=w288, index=w289) -> (element=w287:T4)
            n1459 = call "CRYReplace Analysis Curve Name.vi"("Setup in"=w287, "Step Setup In"=w283, "InsertSocket?"=FALSE, "Type In"="AddStep") -> ("Signal Type"=w286:string, "New Custom Type( Channel case)"=w285:string[])  [unwired: 3 in, 3 out]
            n1460 = Unbundle By Name(w294) -> ("Signal Type"=w292:string)
            n1461 = case shown="True" w299 {
              tunnel: w300 -> [w411 w414]
              tunnel: [w411 w413] -> w298
              tunnel: w292 -> [_ w412]
              frame False {
              }
              frame True {
                n1462 = for {
                  tunnel: w414 -> [w416] mode=indexing
                  tunnel: [w417] -> w413 mode=indexing
                  tunnel: w412 -> [w415]
                  n1463 = Concatenate Strings(w416, " [" ("RecordDelay"), w415, "]" ("string")) -> (w417:string)
                }
              }
            }
            n1464 = call "CRYGet Changed Ana Curve Name.vi"("Old Name"=w305, "Signal Tyep"=w286, "Current Name"=w298, "Changed Name Table in"=w301, "New Custom Type( Channel case)"=w285, "Load?"=w302) -> ("Changed Name Table  out"=w304:string[][])  [unwired: 9 in]
            n1465 = property on="Changed Curve" class="Arr (strict)"("Value"=w304) -> ()  [unwired: 2 in, 2 out]
            n1466 = flat-sequence {
              tunnel: w304 -> [_]
              tunnel: w298 -> [w422]
              frame #0 {
                "Old Name" <- w422
              }
            }
            n1467 = property on="Waveforms Out" class="Ring (strict)"("Value"=w261) -> ()  [unwired: 2 in, 2 out]
            n1468 = property on="Waveforms In" class="Ring (strict)"("Value"=w260) -> ()  [unwired: 2 in, 2 out]
          }
          frame #2 {
            n1469 = control-ref of="Board Tab"() -> (w429:refnum<vi>)
            n1470 = control-ref of="This VI"() -> (w430:refnum<vi>)
            n1471 = call "CRYAlign Steps VI Center.vi"("Tab2"=w429, "Input/Output"=TRUE ("Preview"), "VIRef"=w430) -> ()  [unwired: 1 in, 8 out]
            n1472 = stacked-sequence {
              tunnel: w427 -> [w433 _]
              tunnel: w426 -> [w432 _]
              tunnel: w425 -> [w431 _]
              frame #0 {
                n1473 = local write "Harmonics array out"(w433) -> ()
                n1474 = local write "IM array out"(w432) -> ()
                n1475 = local write "Diff array out"(w431) -> ()
              }
              frame #1 {
                n1476 = property on="Algorithm" class="Ring (strict)"() -> ("Value"=w434:u16)  [unwired: 2 in, 2 out]
                n1477 = property on="Algorithm" class="Ring (strict)"("Val(Sgnl)"=w434) -> ()  [unwired: 2 in, 2 out]
              }
            }
          }
          frame #3 {
            n1478 = flat-sequence {
              frame #0 {
                n1479 = local write "Load Test"(FALSE ("Load Test")) -> ()
                n1480 = property on="Board Tab" class="TabCtl (strict)"("Visible"=TRUE) -> ()  [unwired: 2 in, 2 out]
              }
              frame #1 {
                n1481 = local read "AddStep"() -> (w437:bool)
                n1482 = local write "Add Lib"(w437) -> ()
                n1483 = case shown="False" w437 {
                  frame False {
                    n1484 = local read "Mode"() -> (w438:string)
                    n1485 = case shown="\"Load\", \"Revert\"" w438 {
                      frame "False", Default {
                      }
                      frame "Load", "Revert" {
                        n1486 = property on="Manual Apply" class="Bool (strict)"("Value"=TRUE ("Manual Apply")) -> ()  [unwired: 2 in, 2 out]
                      }
                    }
                  }
                  frame True {
                  }
                }
              }
              frame #2 {
                n1487 = local write "Mode"("" ("Mode")) -> ()
                n1488 = local write "AddStep"(FALSE ("AddStep")) -> ()
              }
            }
          }
        }
      }
      frame 4 {
        n1489 = local read "Proper VI No"() -> (w450:i32)
        n1490 = flat-sequence {
          tunnel: [w467] -> w462
          tunnel: [w465] -> w461
          tunnel: w450 -> [w463]
          tunnel: [w467] -> w460
          tunnel: [w463] -> w442
          tunnel: w462 -> [w477]
          tunnel: [w476] -> w459
          tunnel: w461 -> [w476]
          tunnel: [w475] -> w458
          tunnel: [w474] -> w457
          tunnel: w460 -> [w474]
          tunnel: [w473] -> w456
          tunnel: w451 -> [w472]
          tunnel: [w470] -> w449
          tunnel: [w469] -> w446
          tunnel: [w468] -> w443
          tunnel: w442 -> [w468]
          tunnel: w459 -> [w486]
          tunnel: w458 -> [w485]
          tunnel: [w484] -> w455
          tunnel: w457 -> [w484]
          tunnel: [w483] -> w454
          tunnel: w456 -> [w483]
          tunnel: w449 -> [w482]
          tunnel: [w482] -> w448
          tunnel: [w481] -> w447
          tunnel: w446 -> [w481]
          tunnel: [w480] -> w444
          tunnel: w443 -> [w480]
          tunnel: w455 -> [w501]
          tunnel: w454 -> [w500]
          tunnel: w448 -> [w493]
          tunnel: w447 -> [w491]
          tunnel: [w490] -> w445
          tunnel: w444 -> [w490]
          tunnel: w445 -> [w507]
          frame #0 {
            n1491 = Build Array(w463) -> (w466:i32[])
            n1492 = local read "Analysis"() -> (w467:T1)
            n1493 = call "CRYGet Curve Library Data Name.vi"("nData"=w466, "sAction"="GetNamebyStep" ("sOption")) -> ("sNames"=w465:string[])  [unwired: 6 in, 3 out]
          }
          frame #1 {
            n1494 = call "CRYFlatten Analysis.vi"("Analysis"=w477) -> ("Analysis flattened"=w478:string)  [unwired: 10 in]
            n1495 = call "CRYReplace Analysis Curve Name.vi"("Setup in"=w472, "Step Setup In"=w478, "InsertSocket?"=TRUE, "Type In"="AddStep") -> ("New Custom Name( Channel case)"=w470:string[], "Curve Info Array Out"=w473:T14, "Inserted Names Out"=w475:string[], "New Custom Type( Channel case)"=w469:string[])  [unwired: 3 in, 1 out]
          }
          frame #2 {
            n1496 = disable-structure shown="Enabled" {
              disable-tunnel: w486 -> [w488 _]
              disable-tunnel: w485 -> [w487 _]
              frame Disabled {
                n1497 = call "CRYReplace Curve Name of Steps.vi"("Step Category"="Analysis", "New Name"=w487, "Old Name"=w488) -> ()  [unwired: 8 in, 1 out]
              }
              frame Enabled {
                n1498 = call "CRYChange Name by Step Editor.vi"() -> ()  [unwired: 12 in]
              }
            }
          }
          frame #3 {
            n1499 = for {
              tunnel: w500 -> [w505] mode=indexing
              tunnel: [w504] -> w492 mode=indexing
              tunnel: [w503] -> w499 mode=indexing
              tunnel: [w502] -> w498 mode=indexing
              n1500 = Unbundle By Name(w505) -> ("Custom Curve Names"=w504:string, "Custom Curve IDs"=w503:i32, "Default Curve Names"=w502:string)
            }
            n1501 = call "CRYGet Changed Ana Curve Name.vi"("Current Name"=w493, "New Custom Type( Channel case)"=w491) -> ("Changed Name Table  out"=w494:string[][])  [unwired: 13 in]
            n1502 = Build Array(w492) -> (w497:string[][])
            n1503 = Transpose 2D Array(2D array=w497) -> (transposed array=w496:string[][])
            n1504 = property on="Changed Curve" class="Arr (strict)"("Value"=w494) -> ()  [unwired: 2 in, 2 out]
            n1505 = property on="Custom Curve Names" class="Tbl (strict)"("Value"=w496) -> ()  [unwired: 2 in, 2 out]
            n1506 = Bundle By Name(cluster=w501, "Custom Curve Names"=w492, "Custom Curve IDs"=w499, "Default Curve Names"=w498) -> (w495:T1)
            n1507 = property on="Old Name" class="Arr (strict)"("Value"=w493) -> ()  [unwired: 2 in, 2 out]
            n1508 = local write "Analysis"(w495) -> ()
          }
          frame #4 {
            n1509 = global read "CRYStepSetup Global.vi" "Load from AddStep"() -> (w508:bool)
            n1510 = case shown="True" w508 {
              tunnel: w507 -> [_ w510]
              frame False {
              }
              frame True {
                n1511 = global write "CRYStepSetup Global.vi" "Load from AddStep"(FALSE ("Load from AddStep")) -> ()
                n1512 = call "CRYStepData Manipulate.vi"("sAction"="Backup", "StepNo."=w510) -> ()  [unwired: 10 in]
              }
            }
            n1513 = local write "Add Lib"(FALSE ("Add Lib")) -> ()
          }
        }
        n1514 = call "CRYGet Current TS Steps.vi"() -> ("SelectStepNumber in Tree"=w452:i32, "Steps"=w453:T4[])  [unwired: 1 in, 9 out]
        n1515 = Index Array(array=w453, index=w452) -> (element=w451:T4)
      }
      frame 5 {
        n1516 = flat-sequence {
          frame #0 {
            n1517 = global read "CRYMainGlobal.vi" "Access Level"() -> (w513:enum16{"Engineer", "Technician", "Operator"})
            n1518 = case shown="\"Technician\", Default" w513 {
              frame "Engineer" {
                n1519 = flat-sequence {
                  frame #0 {
                    n1520 = local read "Analysis"() -> (w520:T1)
                    n1521 = local read "Proper VI No"() -> (w522:i32)
                    n1522 = call "CRYFlatten Analysis.vi"("Analysis"=w520) -> ("Analysis flattened"=w514:string)  [unwired: 10 out]
                    n1523 = call "CRYPreUpdate Sequence.vi"("EventName"="SequenceUpdate", "Proper VI No"=w522, "Project View Step Name Identifier Arg1"="", "Step flattened Arg2"=w514, "AllChangeFlg"=TRUE ("Name/Identifier")) -> ()  [unwired: 11 in]
                    n1524 = call "CRYGet Current TS Steps.vi"() -> ("SelectStepNumber in Tree"=w517:i32, "Steps"=w516:T4[])  [unwired: 1 in, 9 out]
                    n1525 = Index Array(array=w516, index=w517) -> (element=w515:T4)
                    n1526 = call "CRYReplace Analysis Curve Name.vi"("Setup in"=w515, "Step Setup In"=w514, "InsertSocket?"=TRUE, "Type In"="StepOK") -> ()  [unwired: 3 in, 5 out]
                  }
                  frame #1 {
                    n1527 = call "CRYChange Name by Step Editor.vi"() -> ()  [unwired: 12 in]
                  }
                }
              }
              frame "Technician", Default {
                n1528 = call "CRYGet Error Message.vi"("Kind"="Step Setup") -> ("Window Title"=w527:string)  [unwired: 5 in, 5 out]
                n1529 = call "CRYGet Access Level Message.vi"("sAction"="OK") -> ("Multibyte string"=w529:string)  [unwired: 10 in]
                n1530 = call "CRYMessage Dialog.vi"("Window Title"=w527, "YesNoCancel"=T7."OK", "Message Content"=w529) -> ()  [unwired: 7 in, 2 out]
              }
            }
          }
          frame #1 {
            n1531 = local write "OK"(FALSE ("OK")) -> ()
          }
        }
        n1532 = local write "stop"(TRUE ("stop")) -> ()
      }
      frame 6 {
        n1533 = flat-sequence {
          frame #0 {
            n1534 = local read "Proper VI No"() -> (w532:i32)
            n1535 = call "CRYStepData Manipulate.vi"("sAction"="Restore", "StepNo."=w532) -> ()  [unwired: 10 in]
          }
          frame #1 {
            n1536 = local write "Cancel"(FALSE ("Cancel")) -> ()
          }
        }
        n1537 = local write "stop"(TRUE ("stop")) -> ()
      }
      frame Default {
      }
    }
  }
  n1538 = flat-sequence {
    tunnel: w3 -> [_]
    frame #0 {
      n1539 = control-ref of="This VI"() -> (w1844:refnum<vi>)
      n1540 = call "CRYWork Before Step Close.vi"("StepVI Ref"=w1844) -> ()  [unwired: 11 in]
    }
    frame #1 {
      "EndFlag" <- TRUE ("EndFlag")
    }
  }
